vi "Position_TOTAL_R25test1111.vi"(5 "Distance Between \nCameras  (*unit)":sgl=2.3) -> (12 "dX, dY\nLeft Cam":cluster{"X":sgl[], "Y":sgl[]}={"X"=[-1.0065897, 0.099401906, 1.1628555, 2.2500029, 0.0], "Y"=[10.716516, 10.801518, 10.883252, 10.9668045, 0.0]}, 13 "Position Valid":bool=TRUE, 14 "Left Camera Real Coordinates":cluster{"X":sgl, "Y":sgl}={"X"=10.842023, "Y"=1.3735824}, 16 "dX, dY\nRight Cam":cluster{"X":sgl[], "Y":sgl[]}={"X"=[-2.8840373, -1.7780458, -0.7145921, 0.3725553, -1.8774476], "Y"=[9.387911, 9.472914, 9.554648, 9.638201, -1.3286046]}, 18 "Robot Coordinates":cluster{"X":sgl, "Y":sgl}={"X"=10.17772, "Y"=2.3123062}, 19 "Orietnation\n(current)":sgl=-30.94054 format="%#_13g")   [LabVIEW 2015]
uses:
  <vilib>/Analysis/coordinate.llb/2D Cartesian Coordinate Rotation (Array).vi
  <vilib>/myRIO/Common/Instrument Driver Framework/myRIO v1.0/DIO/vis/myRIO v1.0 Close DIO.vi
  <vilib>/myRIO/Common/Instrument Driver Framework/myRIO v1.0/DIO/vis/myRIO v1.0 Unreserve DIO.vi
  <vilib>/myRIO/Common/Instrument Driver Framework/myRIO v1.0/DIO/vis/myRIO v1.0 Build MUX Configuration DIO.vi
  <vilib>/myRIO/Common/Instrument Driver Framework/myRIO v1.0/Resource Manager/vis/myRIO v1.0 Unreserve Channel List.vi
  <vilib>/myRIO/Common/Instrument Driver Framework/myRIO v1.0/Resource Manager/vis/myRIO v1.0 Create Configuration List.vi
  <vilib>/myRIO/Common/Instrument Driver Framework/myRIO v1.0/Resource Manager/vis/myRIO v1.0 Unreserve Channel.vi
  <vilib>/myRIO/Common/Instrument Driver Framework/myRIO v1.0/Resource Manager/vis/myRIO v1.0 Build Mutex Name.vi
  <vilib>/Instr/_visa.llb/VISA Configure Serial Port (Instr).vi
  <vilib>/myRIO/Common/Instrument Driver Framework/myRIO v1.0/DIO/vis/myRIO v1.0 Shutdown DIO.vi
  <vilib>/Utility/error.llb/Error Cluster From Error Code.vi
  <vilib>/myRIO/Common/Instrument Driver Framework/myRIO v1.0/Resource Manager/vis/myRIO v1.0 Configure IO.vi
  <vilib>/myRIO/Common/Instrument Driver Framework/Utilities/vis/Configuration Manager.vi
  <vilib>/myRIO/Common/Instrument Driver Framework/Utilities/vis/IO Manager.vi
  <vilib>/myRIO/Common/Instrument Driver Framework/myRIO v1.0/myRIO v1.0 Close.vi
  <vilib>/Analysis/NI_AALPro.lvlib
  <vilib>/myRIO/Instrument Drivers/Onboard IO/DIO/DIO.lvlib
panel:
  in  "Boolean":bool
  in  "Skip Startup - LEFT":bool[](array[boolean])=[FALSE, TRUE, FALSE, FALSE, TRUE, FALSE, FALSE, TRUE]
  in  "Startup GP per Case - LEFT 2":u16[](array[numeric])=[920, 0, 260, 700, 0, 200, 650, 0, 358]
  in  "Start up Template State\n- LEFT":i32=1
  out "Current Template - Right":T1(ring)
  out "Current Template - Left":T1(ring)
  in  "Tab Control 2":T2(tab)
  out "Beacon Coordinates - Right Image":T3={"Beacon Position - X px"=[88.975365, 121.85722, 157.60713, 192.74931, 229.82234], "Beacon Position - Y px"=[106.21975, 102.49595, 103.61968, 103.22959, 103.920715]}
  out "Beacon Coordinates - Left Image":T3={"Beacon Position - X px"=[96.57839, 127.0317, 159.93825, 190.94315, 221.86247], "Beacon Position - Y px"=[111.67795, 107.306076, 106.92789, 105.73433, 104.09002]}
  in  "Image Width (px)":sgl=320.0
  in  "Image Height (px)":sgl=240.0
  in  "Cam AOV Horizontal (deg)":sgl=58.0
  in  "Cam AOV Vertical (deg)":sgl=45.0
  out "Angle to Pixel Ratios":T4={"Angle to Pixel\nRatio - Horizontal"=0.18125, "Angle to Pixel\nRatio - Vertical"=0.1875} {"Angle to Pixel\nRatio - Vertical" format="%#_13g"; "Angle to Pixel\nRatio - Horizontal" format="%#_13g"}
  in  "Num of Beacons (Total)":i8=5
  out "Left Data\nInput Flag\n- Internal":bool
  out "Right Data\nInput Flag\n- Internal":bool
  out "This Servo \nAngle - Left":sgl=52.96875
  in  "Valid Angles - L":bool[](array[boolean])=[TRUE, TRUE, TRUE, TRUE, TRUE]
  in  "Valid Angles -R":bool[](array[boolean])=[TRUE, TRUE, TRUE, TRUE, TRUE]
  in  "Beacon Angles - L":sgl[](array[numeric])=[64.19745, 58.642975, 52.682835, 47.05908, 41.446476]
  in  "Beacon Angles -R":sgl[](array[numeric])=[71.43643, 65.46979, 58.9926, 52.62266, 45.904842]
  out "This Servo \nAngle - Right":sgl=58.76953
  in  "Position Calc\nReady":bool=TRUE
  out "Array":sgl[](array[numeric])=[9.555056, 8.575206, 8.036942, 7.810829, 6.6351933]
  out "Array 2":sgl[](array[numeric])=[5.5039287, 6.210328, 7.1312, 8.266513, 8.73579]
  out "Array 3":sgl[](array[numeric])=[3.2039287, 3.9103284, 4.8311996, 5.9665127, 6.4357905]
  in  "stop":bool
  in  "Startup GP per Case - RIGHT":u16[](array[numeric])
  in  "Startup GP per Case - LEFT":u16[](array[numeric])
  in  "Servo Algorithm\nCycle Time(ms)":i32=25
  in  "Move Servo\nThreshold (deg)":sgl=2.0 format="%#_13g"
  in  "SERVO ENABLE":bool=TRUE
  in  "Max Write\nTx Attempts":u8=3
  in  "Max Read\nTx Attempts":u8=3
  in  "close comms":bool
  in  "Servo Comm\nLoop Time (ms)":i32=20
  out "dT - Comm Loop":u32=21
  in  "Left Servo\nID":string="\u0000"
  in  "Servo Comm\nWait Time - (ms)":i32
  in  "Right Servo\nID":string="\u0001"
  in  "Search Step Size\n(deg)":sgl=15.0 format="%#_13g"
  out "Last Orientation":sgl=-35.285717
  out "Last Position":cluster{"X":sgl, "Y":sgl}={"X"=10.147585, "Y"=2.64441}
  in  "Compliance Slope":u8=128
  in  "Search Step Size":u16=50
  in  "Mounting Offset - Left":sgl=-45.0
  in  "Minimum Delta \nServo Threshold":i16=3
  in  "Maximum Move \nServo Threshold":i16=300
  in  "Wait Tick Threshold":i32=10
  in  "Min Num Frames\nper Search":i32=5
  in  "Middle Beacon\nCoordinates":cluster{"X":sgl, "Y":sgl}={"X"=0.0, "Y"=2.5}
  in  "Max Recovery\nSearch Attempts":u16=3
  in  "Max Recovery Count\n(Recovery Search)":u16=20
  in  "Mounting Offset - Right":sgl=45.0
  in  "Tracking Timeout\nThreshold":i32=10
  in  "Timeout to \nEnable Reactive Predict":u16=5
  out "Beacon Scales - Right":sgl[](array[numeric])=[50.81787, 54.150085, 54.01553, 51.723366, 54.605507]
  out "Beacon Scales - Left":sgl[](array[numeric])=[46.59789, 48.180458, 47.842606, 46.504417, 45.297752]
  in  "Recovery Parallel\nSearch Offset":u16=50
  in  "Max # Pan Moves":u16=20
  in  "Current Angle\n - Right (internal)":sgl=58.76953
  in  "Current Angle\n - Left (internal)":sgl=52.96875
  in  "Servo Goal Position\n - Left":u16=360
  in  "Servo Goal Position\n - Right":u16=667
  out "Move Servo - R":bool
  out "Move Servo - L":bool
  out "Current L (10bit)":u16=232
  out "Servo Moving - L":bool
  out "Servo Moving - R":bool
  out "Current R (10bit)":u16=559
  out "deltaMoveServo\n- L":i16
  out "Move Respond - L":bool
  out "Move Respond - R":bool
  out "deltaMoveServo\n- R":i16
  out "Current Main State - Left":T5(ring)=enum."Tracking"
  in  "Initial Main State - Left":T5(ring)
  in  "Image Lock - Left":bool=TRUE
  in  "Track Angle Valid - Left":bool=TRUE
  out "New Data  Flag\nLeft Servo":bool
  in  "Tracking Angle - Left":sgl=52.933372
  in  "Search Direction - in - L":bool
  out "Frames Processed\nCount - in -L":i32
  out "Recovery Mode Count - in Left":u16
  in  "Image Lock - Right":bool
  out "Recovery Search\nmove Count - in - L":u16
  out "Recovery Search\nAttempt Count - in - L":u16
  out "Current Move Delta - L":u16
  out "Next Main State - Left":T5(ring)=enum."Tracking"
  in  "Recovery Search\nDirection - L":bool=TRUE
  out "Last Track Angle - L":sgl=52.96875
  in  "Initial Main State- Right":T5(ring)
  out "Current Main State - Right":T5(ring)=enum."Tracking"
  in  "Track Angle Valid  - Right":bool
  out "New Data  Flag\nRight Servo":bool
  in  "Tracking Angle - Right":sgl=58.953144
  out "Recovery Search\nAttempt Count - Right":u16
  out "Recovery Search\nmove Count - Right":u16
  out "Frames Processed\nCount - in Right":i32
  out "Recovery Mode Count in Right":i32
  in  "Recovery Search\nDirection - R":bool
  out "Next Main State - Right":T5(ring)=enum."Tracking"
  in  "Search Direction - in - Right":bool=TRUE
  out "Tracking Timeout\nCount - L":i32
  out "Tracking Timeout\nCount - R":i32
  out "Current Tracking State - Left":enum16{"Track", "Reactive Predict", ""}(ring)
  in  "Initial Tracking State - Left":enum16{"Track", "Reactive Predict", ""}(ring)
  out "Next Tracking State - Left":enum16{"Track", "Reactive Predict", ""}(ring)
  in  "Initial Tracking State - Right":enum16{"Track", "Reactive Predict", ""}(ring)
  out "Current Tracking State - Right 2":enum16{"Track", "Reactive Predict", ""}(ring)
  out "Next Tracking State - Right":enum16{"Track", "Reactive Predict", ""}(ring)
  in  "Initial Recovery State - L":enum16{"Generic Sweep", "Recovery Search"}(ring)=enum."Recovery Search"
  in  "Initial Recovery State  - Right":enum16{"Generic Sweep", "Recovery Search"}(ring)=enum."Recovery Search"
  out "Current Recovery State - Right":enum16{"Generic Sweep", "Recovery Search"}(ring)=enum."Recovery Search"
  out "Next Recovery State - Right":enum16{"Generic Sweep", "Recovery Search"}(ring)=enum."Recovery Search"
  out "Next Recovery State - Left":enum16{"Generic Sweep", "Recovery Search"}(ring)=enum."Recovery Search"
  out "Current Recovery State -L":enum16{"Generic Sweep", "Recovery Search"}(ring)=enum."Recovery Search"
  out "Current Move Delta - R":u16
  in  "Mining Alignment\nEnabled":bool
  in  "Real Beacon\n - Coordinates":cluster{"X":dbl[], "Y":dbl[]}={"X"=[0.0, 0.0, 0.0, 0.0, 0.0, 0.0], "Y"=[0.5, 1.5, 2.5, 3.5, 4.5, 0.0]}
  out "LOCAL\nBeacon Coordinates\nRelative to Robot":cluster{"dX_beacon":sgl[], "dY_beacon":sgl[]}={"dX_beacon"=[5.5039287, 6.210328, 7.1312, 8.266513, 8.73579], "dY_beacon"=[9.555056, 8.575206, 8.036942, 7.810829, 6.6351933]}
  out "Local Coordinates - Calculated":cluster{sgl[], sgl[]}(graph)={[5.5039287, 6.210328, 7.1312, 8.266513, 8.73579], [9.555056, 8.575206, 8.036942, 7.810829, 6.6351933]}
  out "Distance to LBF":sgl[](array[numeric])=[0.024284193, 0.015691843, 0.008273765, 0.028971607, 0.03291407]
  out "Right Camera Real Coordinate":cluster{"X":sgl, "Y":sgl}={"X"=9.513418, "Y"=3.25103}
  out "Post Filtering\n- Valid Beacons":bool[](array[boolean])=[TRUE, TRUE, TRUE, TRUE, FALSE]
  in  "Distance\nBetween Beacons":sgl=1.0 format="%#_13g"
  in  "Distance\nBetween Beacons \n- Tolerance":sgl=0.5 format="%#_13g"
  in  "Distance Threshold\nRef Triangles (*unit)":sgl=30.0
  out "All Object Coordinates \n- Local":cluster{"X":sgl[], "Y":sgl[]}={"X"=[2.3, 5.368779, 6.320682, 7.235974, 8.171657, 0.0], "Y"=[0.0, 9.329155, 8.759661, 8.21207, 7.6522775, 0.0]}
  out "Local Coordinates - Normalized":cluster{sgl[], dbl[]}(graph)={[2.3, 5.368779, 6.320682, 7.235974, 8.171657, 0.0], [0.0, 9.329154968261719, 8.759660720825195, 8.21207046508789, 7.65227746963501, 0.0]}
  out "All Object Coordinates \n- Local - Rotated":cluster{"X":sgl[], "Y":sgl[]}={"X"=[1.8774476, -1.0065897, 0.099401906, 1.1628555, 2.2500029, 0.0], "Y"=[1.3286046, 10.716516, 10.801518, 10.883252, 10.9668045, 0.0]}
  out "Local Coordinates - Rotated":cluster{dbl[], dbl[]}(graph)={[1.8774476489648846, -1.0065896210507148, 0.09940190570174412, 1.1628555490135675, 2.250002943734801, 0.0], [1.3286045709883498, 10.716515276262749, 10.801518262128845, 10.883252530212562, 10.966804865321656, 0.0]}
  out "Right_Flag 2":bool
  out "Beacons Found\n- Right (Bool Array)":bool[](array[boolean])=[TRUE, TRUE, TRUE, TRUE, TRUE]
  out "RIGHT Beacon Position - Y px (IN)":sgl[](array[numeric])=[106.21975, 102.49595, 103.61968, 103.22959, 103.920715]
  out "RIGHT Beacon Coord - X px (IN)":sgl[](array[numeric])=[88.975365, 121.85722, 157.60713, 192.74931, 229.82234]
  out "Left_Flag 2":bool
  out "Beacons Found\n- Left (Bool Array) 2":bool[](array[boolean])=[TRUE, TRUE, TRUE, TRUE, TRUE]
  out "LEFT Beacon Coord - X px (IN) 2":sgl[](array[numeric])=[96.57839, 127.0317, 159.93825, 190.94315, 221.86247]
  out "LEFT Beacon Position - Y px (IN) 2":sgl[](array[numeric])=[111.67795, 107.306076, 106.92789, 105.73433, 104.09002]
  in  "Fetch Input\n(mSec)":u32=20 caption="Update Camera Input\n(mSec)"
  in  "Max Std Dev (5)":sgl=0.1 format="%#_13g"
  out "Position \nLock Status":bool=TRUE
  out "Real Position in Course 2":cluster{"X":dbl[], "Y":dbl[]}(graph)={"X"=[10.147584990557128], "Y"=[2.644409845240164]}
  out "Robot Coordinates - Avgd":cluster{"X":sgl, "Y":sgl}={"X"=10.147585, "Y"=2.64441}
  in  "Max Std Dev (4)":sgl=0.1 format="%#_13g"
  in  "Max Std Dev (3)":sgl=0.2 format="%#_13g"
  in  "New Position\nWeight (X coord)":sgl=0.8 format="%#_13g"
  in  "Max X (arena)":sgl=35.0
  in  "Max Y (arena)":sgl=15.0
  in  "History Size":u8=15
  out "Orientation Avgd":sgl=-35.285717
  in  "New Position \nThreshold":sgl=2.0
  out "Robot Coordinates\nHistory":cluster{sgl, sgl}[](array[cluster])=[{10.147585, 2.64441}, {10.056327, 2.8351064}, {10.020484, 2.7815769}, {10.034186, 2.7172103}, {0.0, 0.0}, {10.036168, 2.7859242}, {9.938812, 2.8961887}, {10.1160965, 2.6632404}, {10.016709, 2.7454932}, {10.037537, 2.8544023}, {10.017025, 2.7817721}, {9.997087, 2.8064857}, {10.065648, 2.6537364}, {10.084976, 2.6750228}, {10.082739, 2.688601}]
  out "Orientation\nHistory":sgl[](array[numeric])=[-35.285717, -36.86449, -36.153664, -35.44657, 0.0, -37.6105, -36.02637, -35.82032, -36.08894, -37.01076, -36.293255, -36.40525, -35.738438, -35.683483, -35.770218]
  out "Position Valid\nHistory":bool[](array[boolean])=[TRUE, TRUE, TRUE, TRUE, FALSE, TRUE, TRUE, TRUE, TRUE, TRUE, TRUE, TRUE, TRUE, TRUE, TRUE]
  in  "Moving Average\nWindow Length":u8=10
  in  "New Orientation \nThreshold":sgl=10.0
  in  "Triangle Based\nWeight":sgl format="%#_13g"
  out "Scale Based\nWeight":sgl=1.0 format="%#_13g"
  out "New Position\nWeight (Y coord)":sgl=0.3 format="%#_13g"
  out "New Orientation\nWeight":sgl=0.2
  out "dT":dbl=144.111
  in  "Position Calc\nTimer":u32=100 caption="Position Calc Timer"
  out "inches":dbl
  out "dA2 3":sgl=44.126 format="%#_13g"
  out "Valid Beacon Sets_":bool[](array[boolean])=[TRUE, TRUE, TRUE, TRUE, TRUE]
  in  "Check Shared Var Timer":u32=50 caption="Main Loop\n Timer (ms)"
  out "dA2 2":sgl=48.543114 format="%#_13g"
  out "dA2 4":sgl=48.543114 format="%#_13g"
  out "Last Track Angle - R":sgl=59.941406
  in  "Recovery Search\nDirection - L 2":bool
  in  "Max Recovery Count\n(Recovery Search) 2":u16
  in  "Max Recovery\nSearch Attempts 2":u16
  in  "Image Lock - Right 2":bool
  # "SETTINGS"
  # "IMAGE TO ANGLE VARIABLES"
  # "INPUTS"
  # "OUTPUT VALUES"
  # "CONFIG"
  # "SERVO CONTROL VARIABLES"
  # "SERVO CONTROL VARIABLES"
  # "CONFIG"
  # "SHARED VARIABLE INPUTS"
  # "LOCAL VARIABLE INPUTS"
  # "INTERNRAL VARIABLES"
  # "MISC"
  # "SERVO IDs"
  # "CONTROL DELAYS"
  # "COMM LOOP DELAY"
  # "COMM PROTOCOL"
  # "INDEX Correspondance: \n\n0 - 3  --> Side 1 / N, S, E, W\n4 - 7 -->  Side 2 / N, S, E, W\n9 --> Straight ahead (90deg)"
  # "Make function of distance^^"
  # "LEFT SERVO"
  # "RIGHT SERVO"
  # "Main State Machine"
  # "Recovery State Machine"
  # "Current Track Angle Inputs"
  # "Servo Status Inputs"
  # "Main State Machine Inputs"
  # "Recovery State Machine Inputs"
  # "Current Track Angle Inputs"
  # "Servo Status Inputs"
  # "Tracking State Machine Inputs"
  # "Tracking State Machine Inputs"
  # "POSITION CALCULATION VARIABLES"
  # "OUTPUT VALUES"
  # "CONFIG VALUES"
  # "FILTER CONFIG VALUES"
  # "FEEDBACK INPUT VALUES"
  # "INPUT VALUES"
  # "INTERMEDIATE VALUES"
  # "Use moving average for previous orientation thresholds"
  # "*********************"
  # "unfiltered"
  # "Inter Beacon Distance Filtering"
  # "NOTE: Must be 1 bigger than amount of beacons"
  # "NOTE: Must be 1 bigger than amount of beacons"
  # "VISION PROCESSEING INPUTS"
  # "update to coordinate outlier filtering R2"
  # "NEW FILTER VALS"
  # "MOVING AVERAGE\nVARIABLES"
  # "DISTANCE SOURCE WEIGHT"
  # "*****  I made this 0\n         bc it seems to be \n        more stable"
  # "Recovery State Machine Feedback"
  # "SEARCH ROUTINE VARIABLES"
types:
  T1 = enum16{"Range 1", "Range 2", "Range 3", "Range 0"}
  T2 = enum32{"image to angle ", "Empty", "servo control - Config", "left and right servo - Status", "Position Calc - Debug Data", "Position Calc - Debug Data 2", "Vision Processing INputs", "ROBOT POSITION", "Random"}
  T3 = cluster{"Beacon Position - X px":sgl[], "Beacon Position - Y px":sgl[]}
  T4 = cluster{"Angle to Pixel\nRatio - Horizontal":sgl, "Angle to Pixel\nRatio - Vertical":sgl}
  T5 = enum16{"Start Up Search", "Tracking", "Recovery Mode", ""}
  T6 = cluster{"Lock":bool, "Current Valid":bool, "Current Template":enum16{"Range 1", "Range 2", "Range 3", "Range 0"}, "Tracking Coordinates":cluster{"X":dbl, "Y":dbl}, "Setting Values":cluster{"Min Score":dbl, "Min Scale":dbl, "Max Scale":dbl, "Curve Parameters":cluster{"Min Length":i32, "Row Search Step":i32, "Col Search Step":i32}}}
  T7 = cluster{"Array of Double":dbl[], "Array of Double":dbl[]}
  T8 = enum16{"Sub - 2", "Sub - 3", "Sub - 4", "Normal - 5"}
  T9 = typedef "DIO.lvlib/DIO Reference.ctl" = cluster{"myRIO Reference":T10, "DIO Channels List":T14}
  T10 = typedef "myRIO Generic Hardware Reference.ctl" = cluster{"myRIO Model":T11, "myRIO Hardware Reference":T12}
  T11 = typedef "Hardware Version Enum.ctl" = enum16{"Unknown", "myRIO-1900", "myRIO-1950", "roboRIO"}
  T12 = typedef "myRIO v1.0 Reference.ctl" = cluster{"Generic FPGA Reference":T13, "Allow multiple opens":bool}
  T13 = typedef "Generic FPGA Reference.ctl" = refnum<k20>
  T14 = typedef "DIO Channels List.ctl" = T15[]
  T15 = typedef "DIO Channels Enum.ctl" = enum16{"Not Connected", "C/DIO0", "C/DIO1", "C/DIO2", "C/DIO3", "C/DIO4", "C/DIO5", "C/DIO6", "C/DIO7", "A/DIO0", "A/DIO1", "A/DIO2", "A/DIO3", "A/DIO4", "A/DIO5", "A/DIO6", "A/DIO7", "A/DIO8", "A/DIO9", "A/DIO10", "A/DIO11", "A/DIO12", "A/DIO13", "A/DIO14", "A/DIO15", "B/DIO0", "B/DIO1", "B/DIO2", "B/DIO3", "B/DIO4", "B/DIO5", "B/DIO6", "B/DIO7", "B/DIO8", "B/DIO9", "B/DIO10", "B/DIO11", "B/DIO12", "B/DIO13", "B/DIO14", "B/DIO15", "LED0", "LED1", "LED2", "LED3", "Button0", "DIO/DIO0", "DIO/DIO1", "DIO/DIO2", "DIO/DIO3", "DIO/DIO4", "DIO/DIO5", "DIO/DIO6", "DIO/DIO7", "DIO/DIO8", "DIO/DIO9", "SPI/CS0", "SPI/CS1", "SPI/CS2", "SPI/CS3", "LED RADIO (Green)", "LED RADIO (Red)", "LED COMM (Green)", "LED COMM (Red)", "LED MODE (Green)", "LED MODE (Red)"}
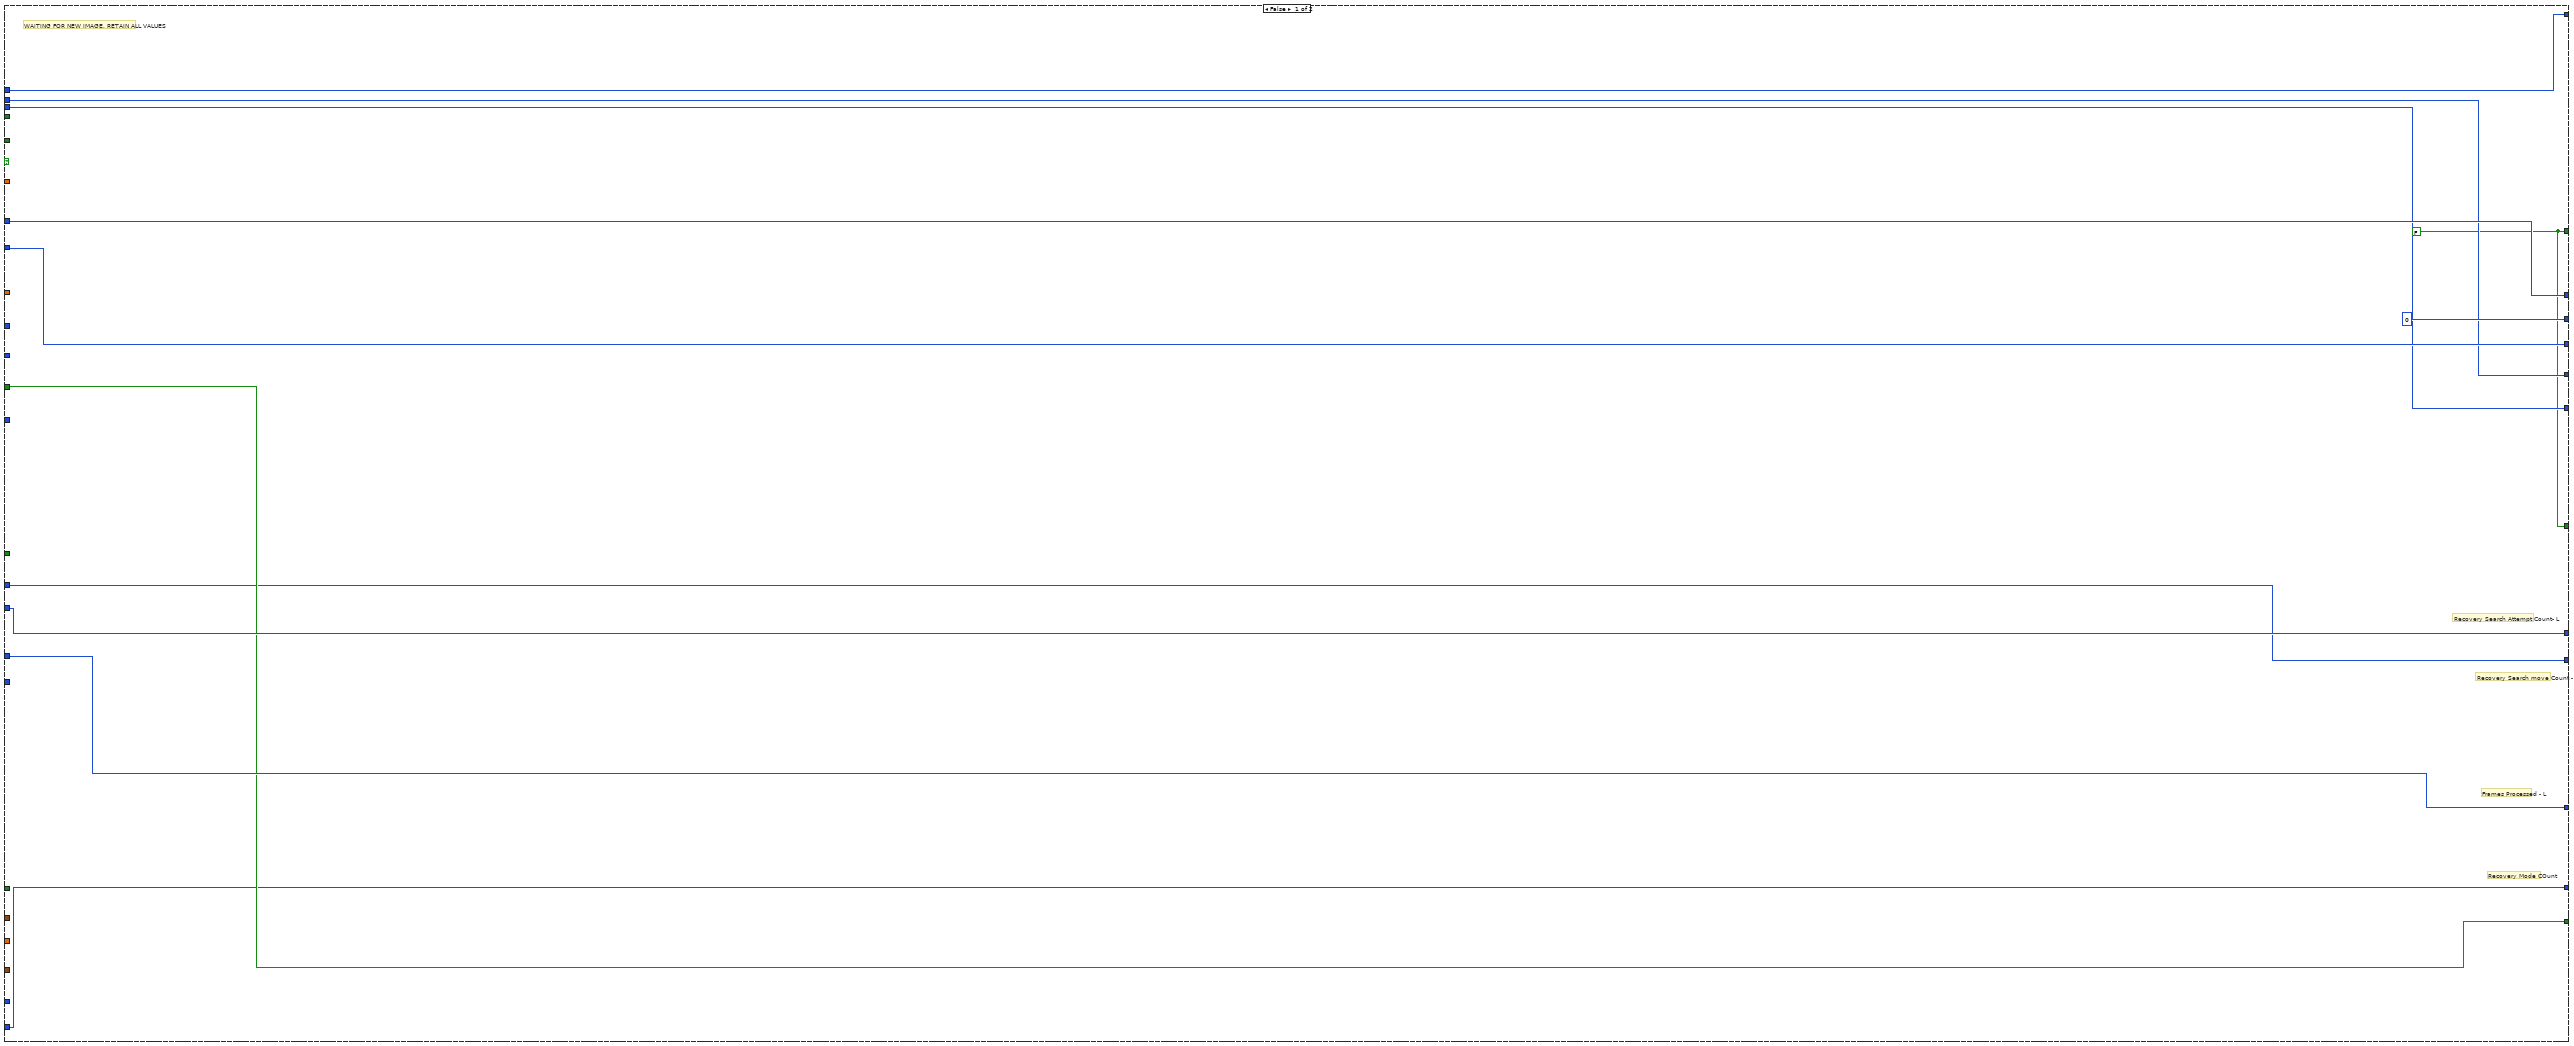
[diagram p2: hidden frame]
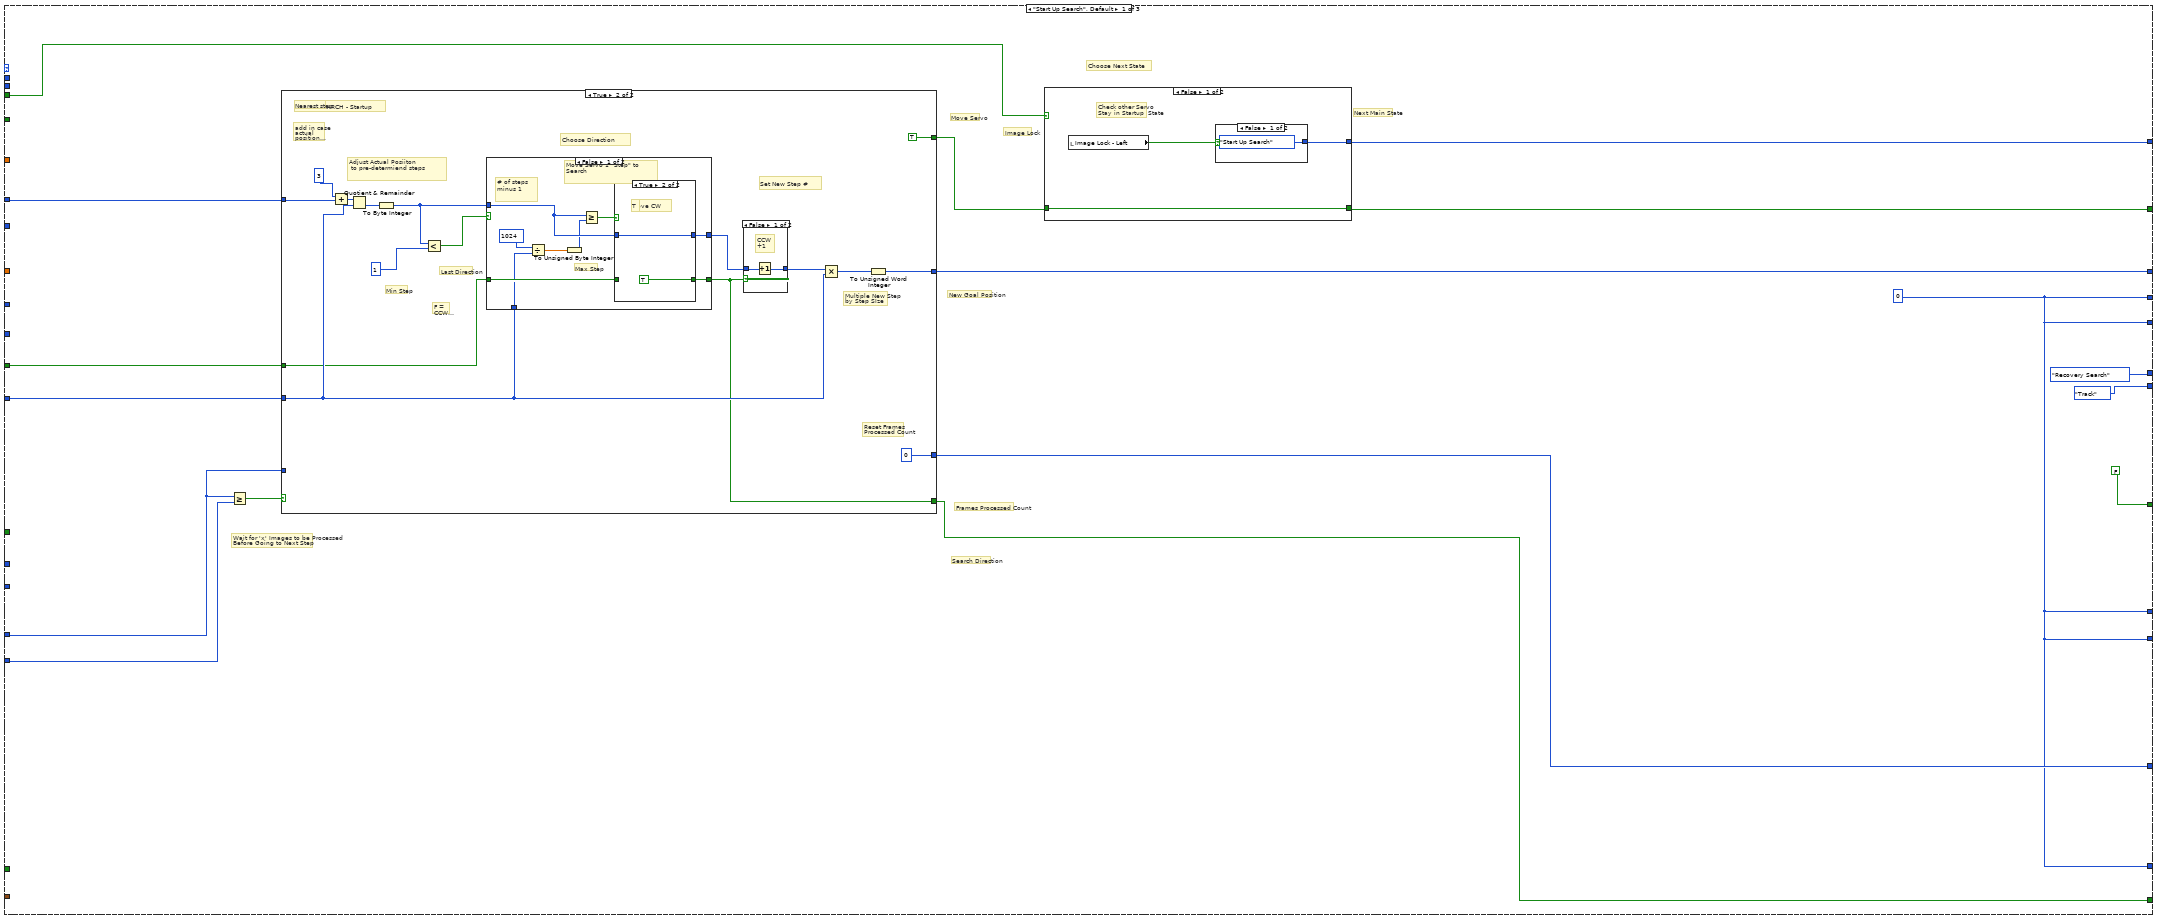
[diagram p3: hidden frame]
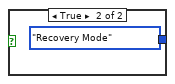
[diagram p4: hidden frame]
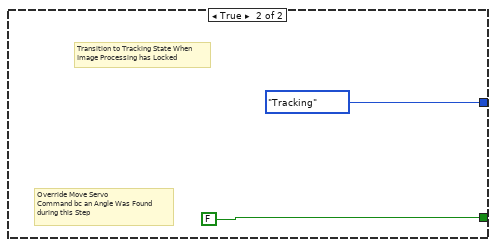
[diagram p5: hidden frame]
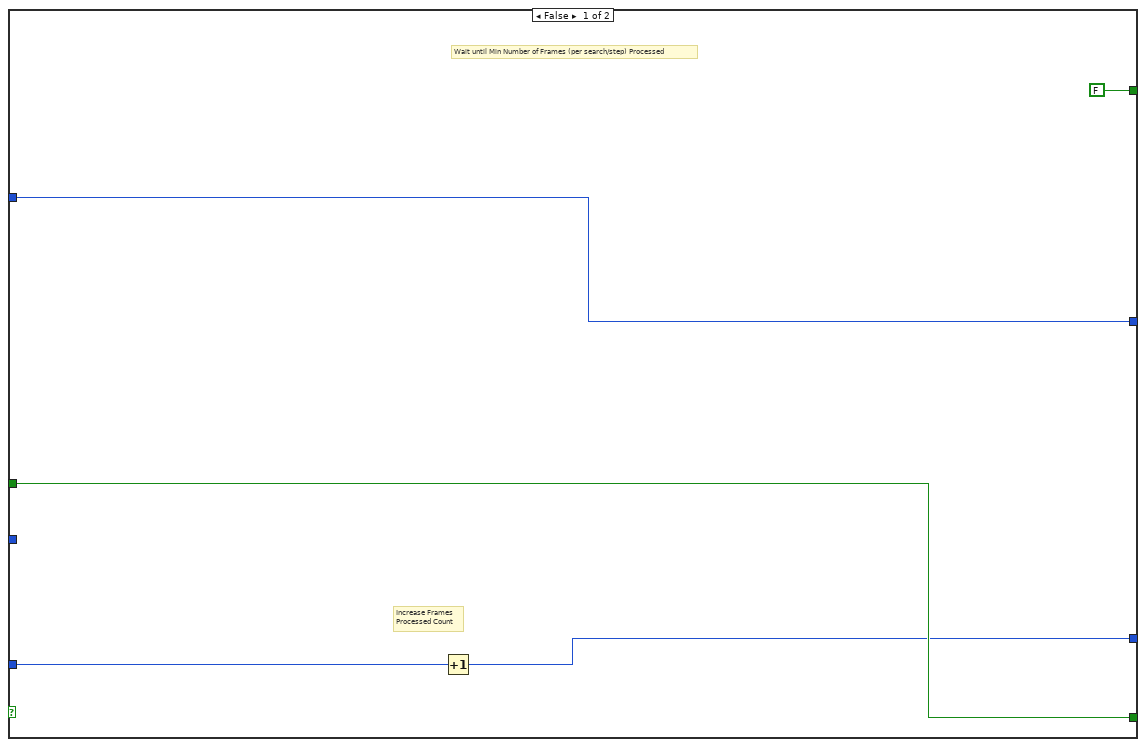
[diagram p6: hidden frame]
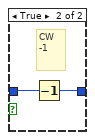
[diagram p7: hidden frame]
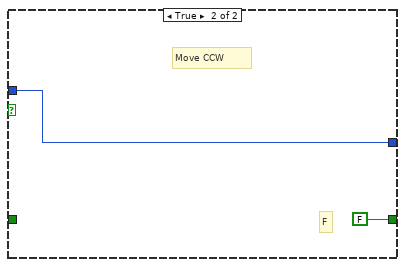
[diagram p9: hidden frame]
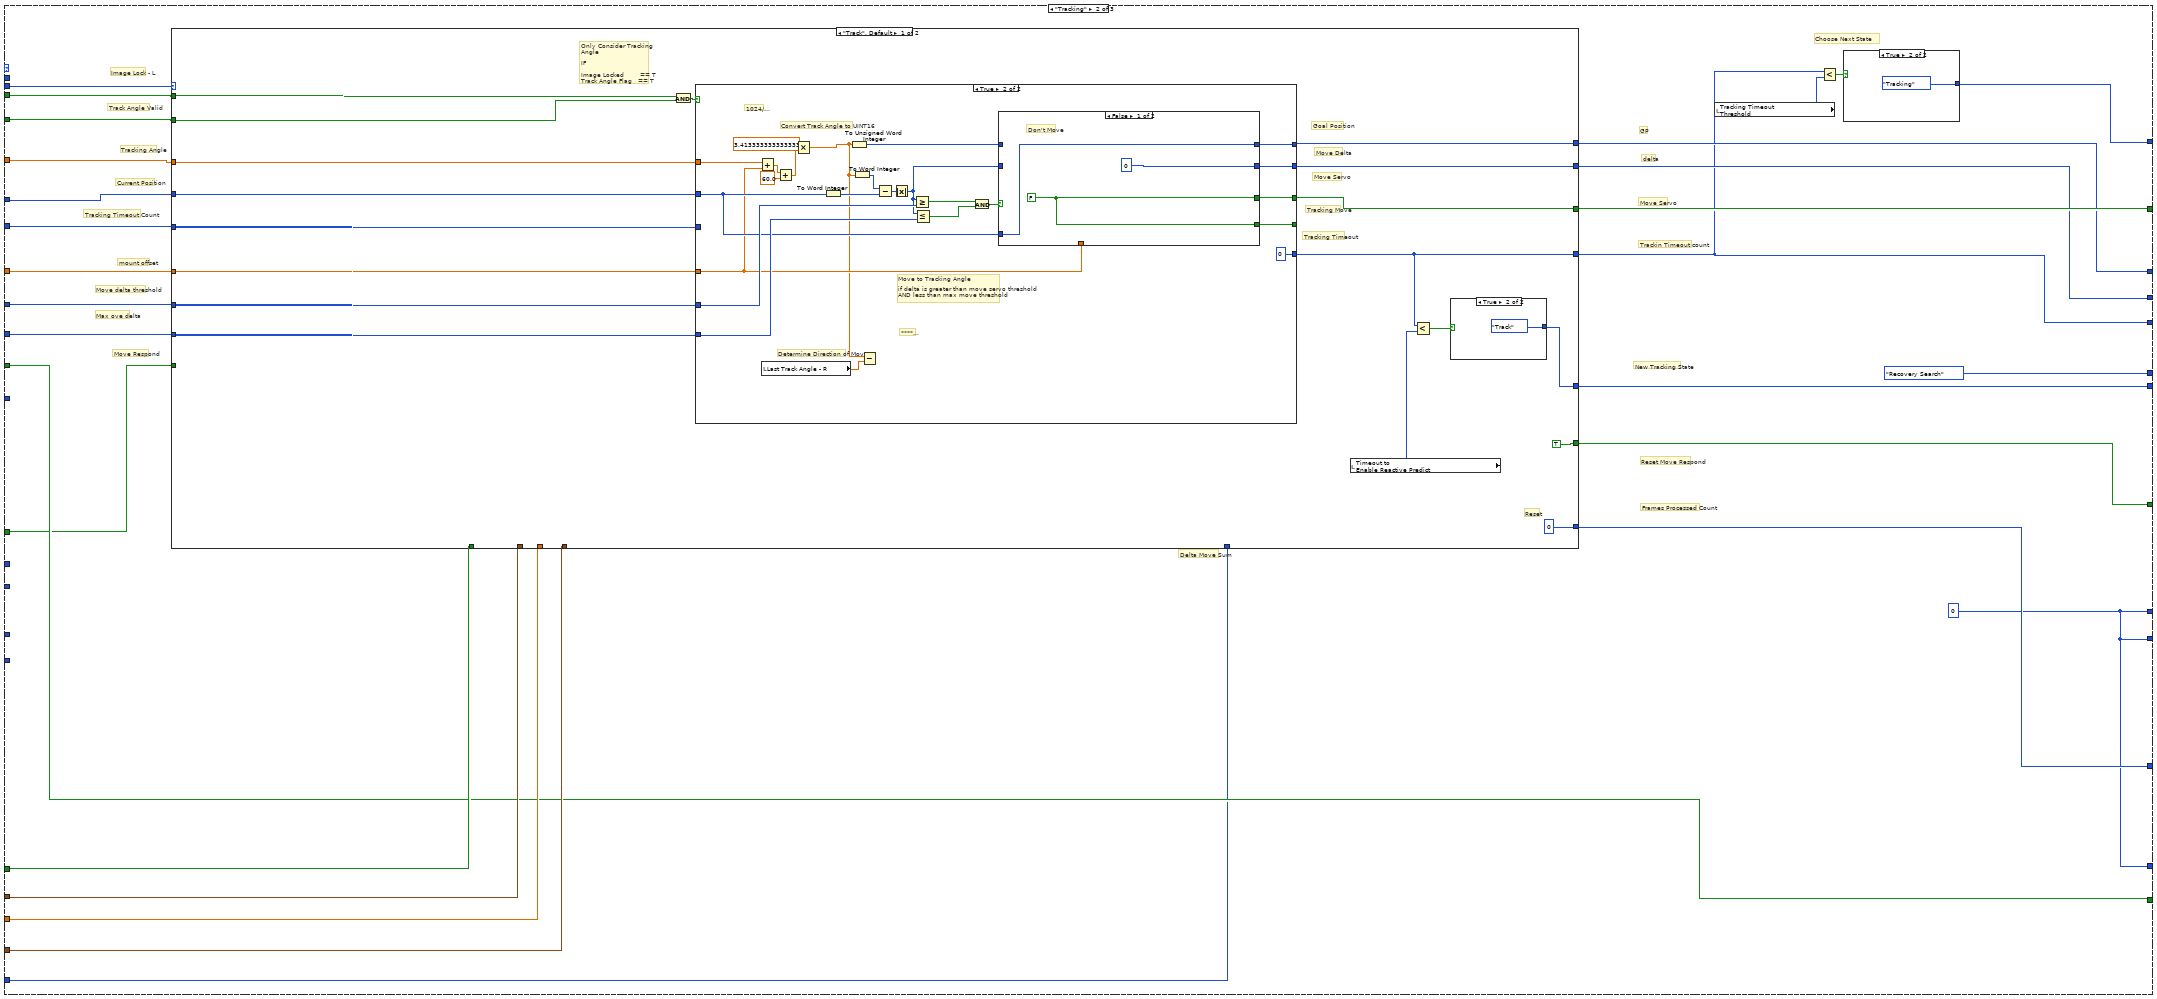
[diagram p10: hidden frame]
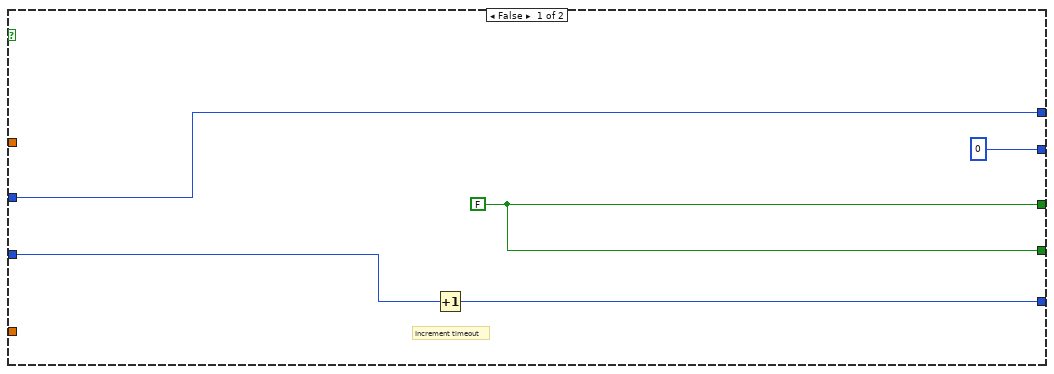
[diagram p11: hidden frame]
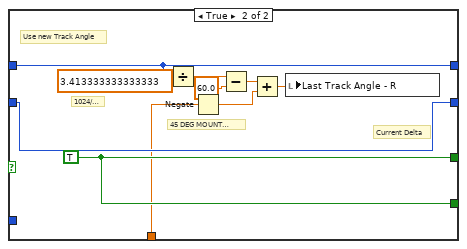
[diagram p12: hidden frame]
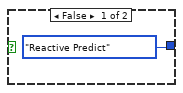
[diagram p13: hidden frame]
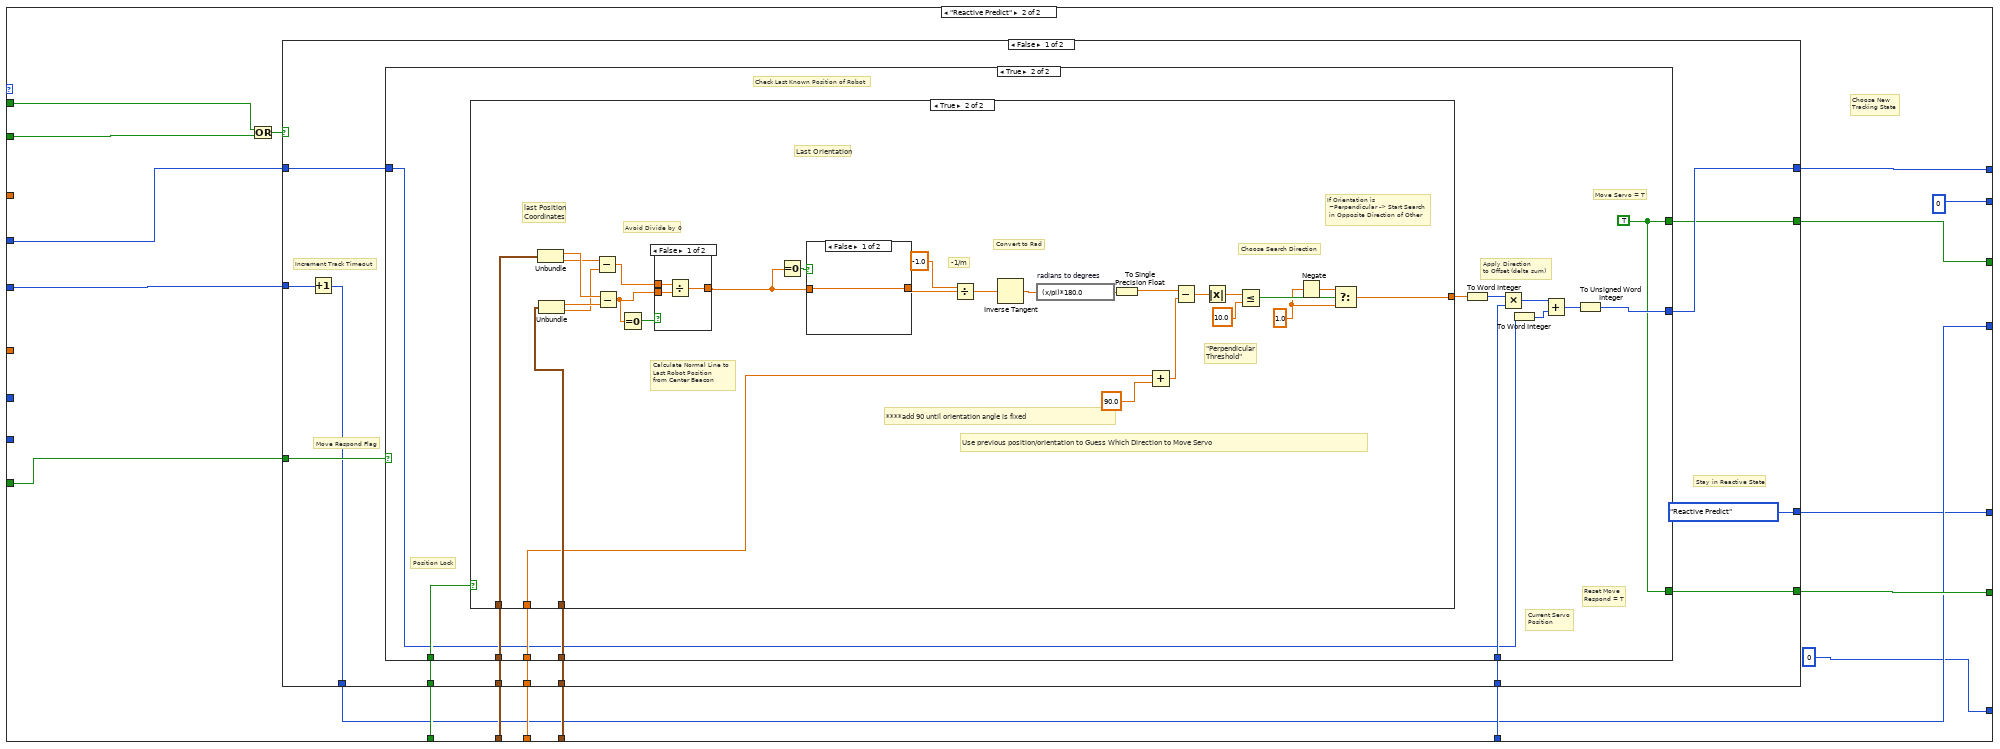
[diagram p14: hidden frame]
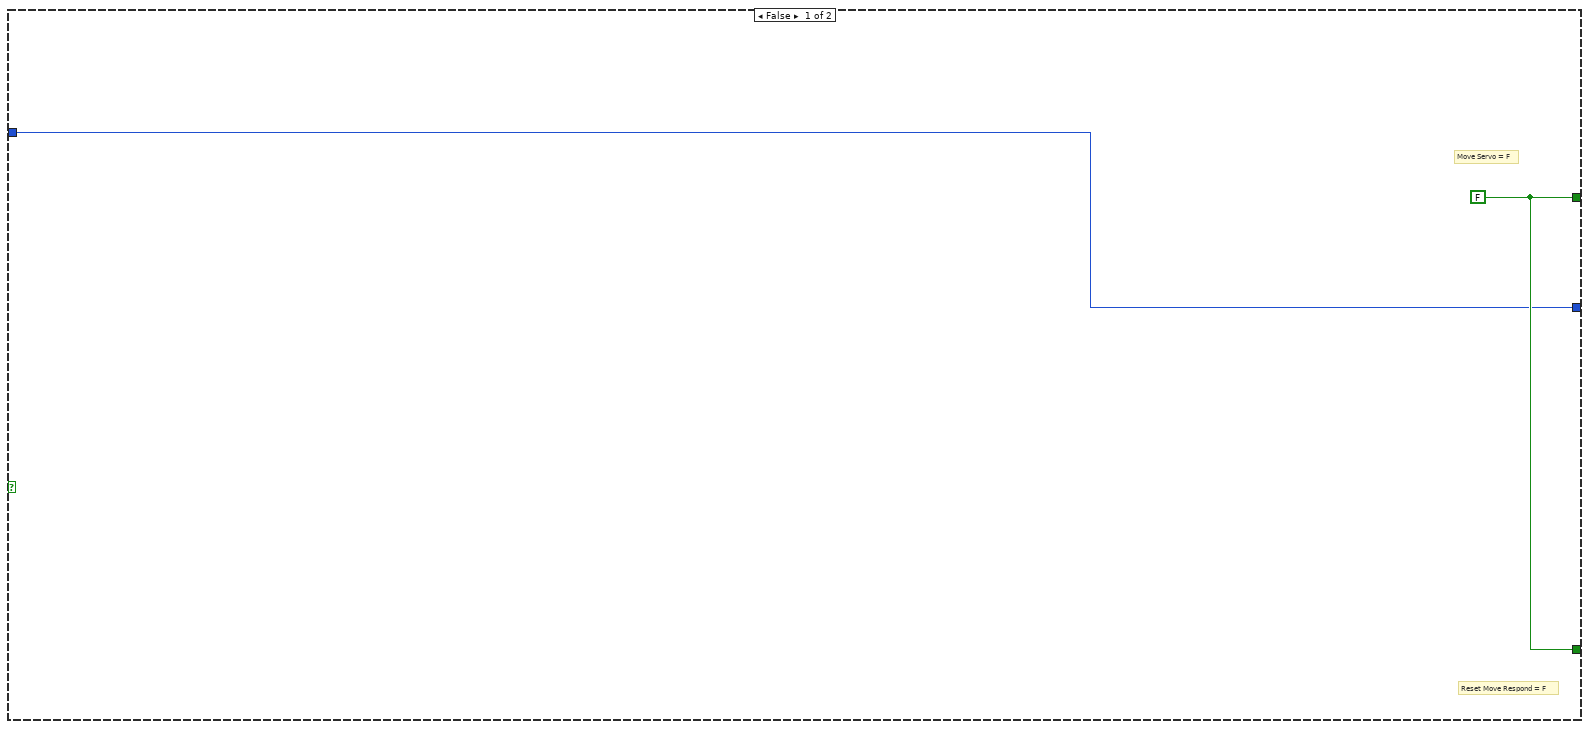
[diagram p15: hidden frame]
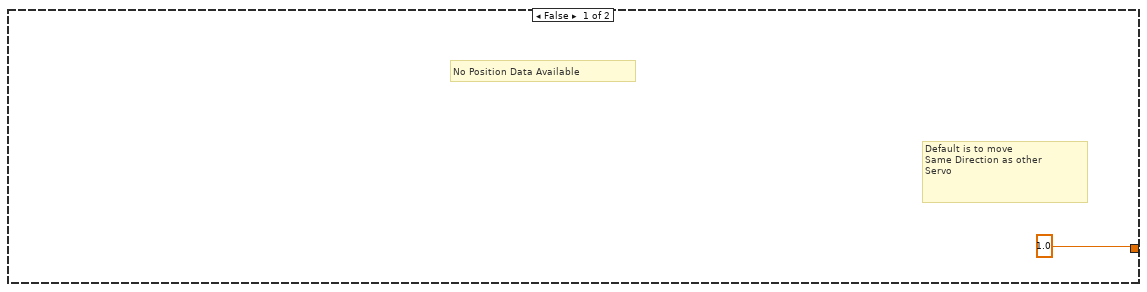
[diagram p16: hidden frame]
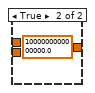
[diagram p17: hidden frame]
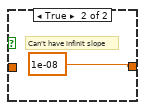
[diagram p18: hidden frame]
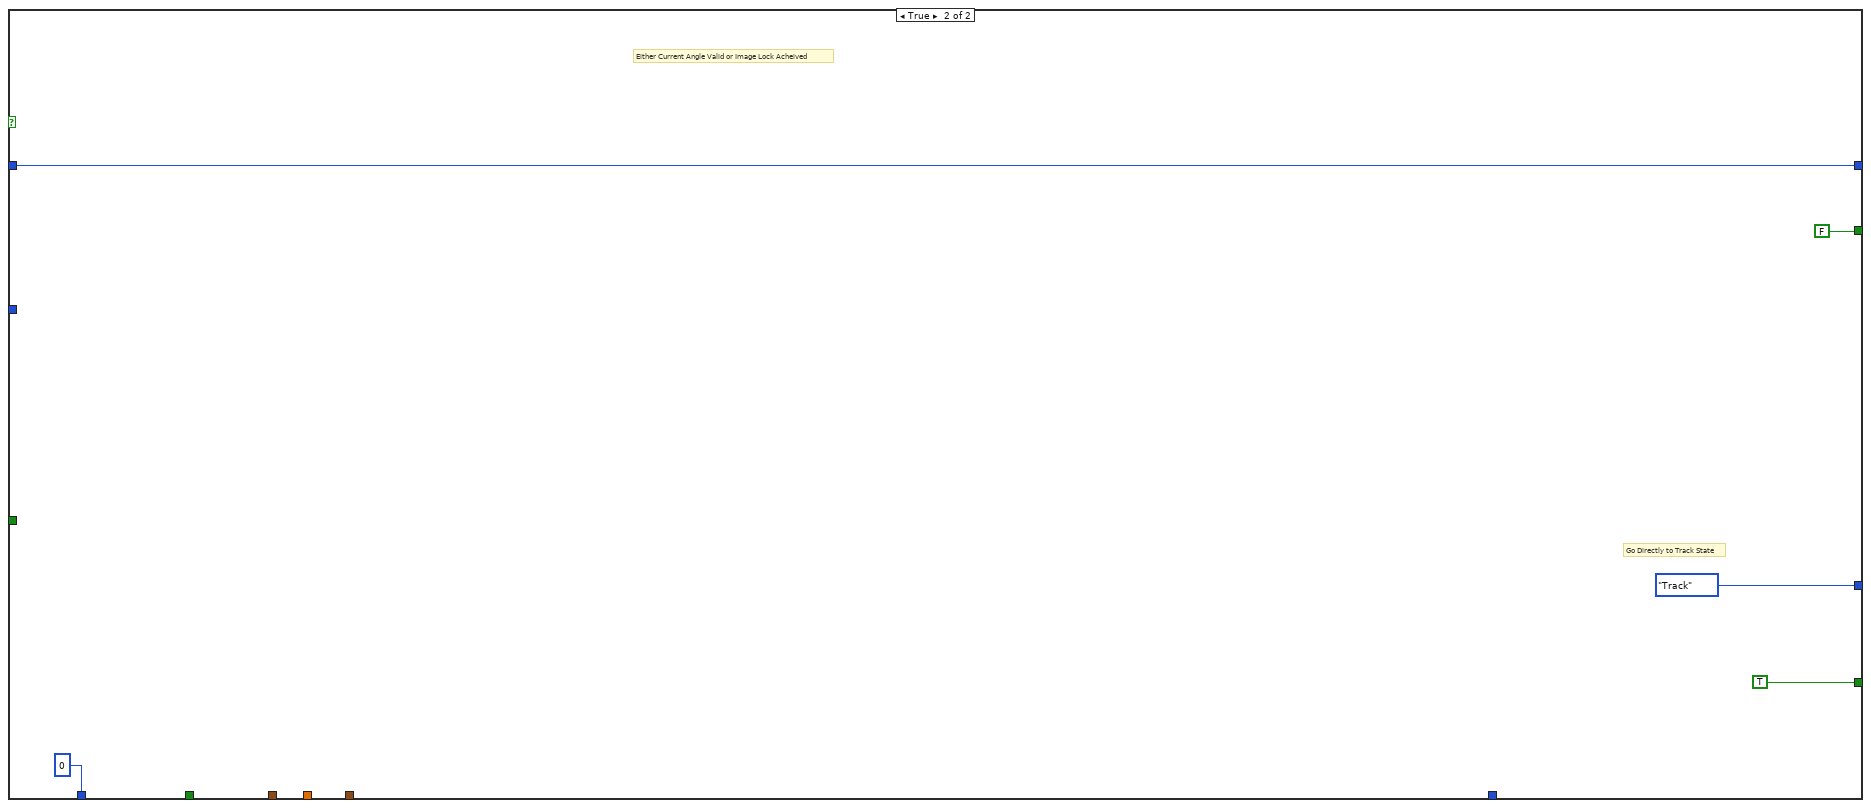
[diagram p19: hidden frame]
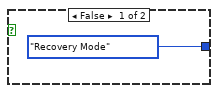
[diagram p20: hidden frame]
diagram:
  (unwired) enum16{"Generic Sweep", "Recovery Search"}."Recovery Search"
  w12 = 0 ("Frames Processed\nCount - in")
  w13 = 0 ("Frames Processed\nCount - in")
  w2 = FALSE
  w34 = sgl 0.0
  # "SERVO CONTROL FLAGS"
  # "***"
  # "Next Tracking State"
  # "Tracking Timeout Count"
  # "Search Direction - L"
  # "Next Recovery State"
  # "Move Respond"
  # "Recovery Mode Count - L"
  # "Delta Move Sum - L"
  # "Wait Tick Count - L"
  # "Frames Processed - L"
  # "Recovery Search move Count - L"
  # "Recovery Search Attempt Count- L"
  # "Next Main State"
  # "Search Direction - L"
  # "Next Recovery State"
  # "INPUTS - Local vars"
  # "Recovery Mode Count - L"
  # "Delta Move Sum - L"
  # "Frames Processed\nLeft"
  # "Move Respond - R"
  # "Initial Search Direction\n- Right"
  # "Move Respond"
  # "Recovery Mode Count - L"
  # "Delta Move Sum - L"
  # "Wait Tick Count - L"
  # "Frames Processed - L"
  # "Recovery Search move Count - L"
  # "Recovery Search Attempt Count- L"
  # "Next Main State"
  # "Settings -- Update in a slow loop"
  # "Recovery Mode Count - L"
  # "Delta Move Sum - L"
  # "Frames Processed\nLeft"
  # "Move Respond - L"
  # "Replace these with\nconstants"
  # "Initial Search Direction\n- Left"
  # "Read Inputs when Available"
  # "# of Physical Beacons"
  # "Right Data Internal Falg"
  # "Left Data Internal Falg"
  # "Initialize Shift Arrays"
  # "Robot Position (cluster)\nShift Array"
  # "Robot Position (cluster)\nShift Array"
  # "Position Valid Shift Array"
  # "Orientation Shift Array"
  # "Position Valid Shift Array"
  # "Orientation Shift Array"
  # "Servo Communication (to Servo- UART))"
  # "Internal Local Variables"
  # "Servo Control Logic"
  # "Local Variables"
  # "Images to Robot Position Calculation Process"
  # "SERVO MOTOR CONTROL"
  # "SERVO MOTOR CONTROL"
  n1 = Divide(x="Cam AOV Horizontal (deg)", y="Image Width (px)") -> (x/y=w25:sgl)
  n2 = Divide(x="Cam AOV Vertical (deg)", y="Image Height (px)") -> (x/y=w26:sgl)
  n3 = Bundle(w25, w26) -> (w20:cluster{sgl, sgl})  [unwired: 1 in]
  "Angle to Pixel Ratios" <- w20
  n4 = disable-structure shown="Disabled" {
    frame Disabled {
      # "Always Read Incoming Flags & Store"
      n5 = while {
        tunnel: "Check Shared Var Timer" -> [w46]
        stop <- FALSE stop-if-true
        n6 = shared-variable "myRIO-1900\\Lib1.lvlib\\RIGHT_FLAG"() -> (→"Right_Flag 2":bool)  [unwired: 1 in, 1 out]
        n7 = shared-variable "myRIO-1900\\Lib1.lvlib\\Left_Flag"() -> (→"Left_Flag 2":bool)  [unwired: 1 in, 1 out]
        n8 = call "Wait8"("Count(mSec)"=w46) -> ()  [unwired: 1 out]
      }
    }
    frame Enabled {
    }
  }
  n9 = while {
    shift-right: [w55] -> _
    shift-left: w2 -> [w60]
    shift-right: [w54] -> _
    shift-left: w2 -> [w58]
    tunnel: w20 -> [w56]
    tunnel: "Num of Beacons (Total)" -> [w57]
    stop <- FALSE stop-if-true
    # "Wait for Both Internal Flags"
    n10 = call "Wait6"("Count(mSec)"="Fetch Input\n(mSec)") -> ()  [unwired: 1 out]
    n11 = shared-variable "RT myRIO Target - Overlord\\Localization_Variables_r0.lvlib\\RIGHT_FLAG"() -> (w51:bool)  [unwired: 1 in, 1 out]
    n12 = shared-variable "RT myRIO Target - Overlord\\Localization_Variables_r0.lvlib\\Left_Flag"() -> (w52:bool)  [unwired: 1 in, 1 out]
    n13 = case shown="True" w51 {
      tunnel: w57 -> [_ w79]
      tunnel: w56 -> [_ w77]
      tunnel: [w61 w67] -> w49
      tunnel: w58 -> [w61 _]
      frame False {
        # "Don't Update Servo Position\nbc we're waiting on new Data to\ncome in and the servo position\nwas set at the previous set of data"
      }
      frame True {
        w67 = TRUE
        # "Store Values"
        # "Raise Internal Flag"
        # "If New Data Available"
        # "From Shift Reg"
        # "Perforrm Indivudual Angle Calculation"
        # "Pull Down Individual Flag"
        n14 = shared-variable "RT myRIO Target - Overlord\\Localization_Variables_r0.lvlib\\RIGHT_BEACON_X_array"() -> (w73:dbl[])  [unwired: 1 in, 1 out]
        "RIGHT Beacon Coord - X px (IN)" <- w73
        n15 = shared-variable "RT myRIO Target - Overlord\\Localization_Variables_r0.lvlib\\Image Lock - R"() -> (w68:bool)  [unwired: 1 in, 1 out]
        n16 = shared-variable "RT myRIO Target - Overlord\\Localization_Variables_r0.lvlib\\RIGHT_BEACON_Scales"() -> (→"Beacon Scales - Right":sgl[])  [unwired: 1 in, 1 out]
        n17 = shared-variable "RT myRIO Target - Overlord\\Localization_Variables_r0.lvlib\\Info - Right"() -> (w65:T6)  [unwired: 1 in, 1 out]
        n18 = shared-variable "RT myRIO Target - Overlord\\Localization_Variables_r0.lvlib\\RIGHT_BEACON_Y_array"() -> (w72:dbl[])  [unwired: 1 in, 1 out]
        "RIGHT Beacon Position - Y px (IN)" <- w72
        n19 = shared-variable "RT myRIO Target - Overlord\\Localization_Variables_r0.lvlib\\RIGHT_BEACON_BOOL_array"() -> (w71:bool[])  [unwired: 1 in, 1 out]
        "Beacons Found\n- Right (Bool Array)" <- w71
        n20 = Unbundle By Name(w65) -> ("Tracking Coordinates"=w64:cluster{"X":dbl, "Y":dbl}, "Current Valid"=w63:bool, "Current Template"=→"Current Template - Right":T1)
        n21 = local write "Image Lock - Right"(w68) -> ()
        n22 = Bundle("Array of Double"=w73, "Array of Double"=w72) -> (w70:T7)  [unwired: 1 in]
        "Beacon Coordinates - Right Image" <- w70
        n23 = shared-variable "RT myRIO Target - Overlord\\Localization_Variables_r0.lvlib\\Right Servo Angle_Image"() -> (w69:dbl)  [unwired: 1 in, 1 out]
        "This Servo \nAngle - Right" <- w69
        n24 = shared-variable "RT myRIO Target - Overlord\\Localization_Variables_r0.lvlib\\RIGHT_FLAG"(FALSE) -> ()  [unwired: 1 in, 1 out]
        n25 = feedback #1() -> (w81:sgl[])  [unwired: 1 in]
        n26 = feedback #2() -> (w80:bool[])  [unwired: 1 in]
        n27 = call "Angle Calc_Individual Process R4.vi"("Angle to Pixel Ratios"=w77, "Previous Angles"=w81, "Num of Beacons"=w79, "Beacon Coordinates - Image"=w70, "Current Servo Angle"=w69, "Beacons Found (Bool Array)"=w71, "Previous Valid Angles"=w80, "Tracking Coordinates"=w64) -> ("Servo Goal Angle"=w76:sgl, "Valid Beacons (Bool Array)\nPosition Calc"=w75:bool[], "Angle Of Beacons \nRelative to Robot"=w74:sgl[])  [unwired: 4 in, 1 out]
        n28 = feedback-in #1(w74) -> ()
        n29 = feedback-in #2(w75) -> ()
        n30 = local write "Tracking Angle - Right"(w76) -> ()
        n31 = local write "Beacon Angles -R"(w74) -> ()
        n32 = local write "Valid Angles -R"(w75) -> ()
        n33 = local write "Track Angle Valid  - Right"(w63) -> ()
        n34 = local write "New Data  Flag\nRight Servo"(w67) -> ()
      }
    }
    "Right Data\nInput Flag\n- Internal" <- w49
    n35 = case shown="True" w52 {
      tunnel: [w82 w88] -> w48
      tunnel: w60 -> [w82 _]
      tunnel: w56 -> [_ w92]
      tunnel: w57 -> [_ w91]
      frame False {
        # "Don't Update Servo Position\nbc we're waiting on new Data to\ncome in and the servo position\nwas set at the previous set of data"
      }
      frame True {
        w88 = TRUE
        # "Store Values"
        # "Raise Internal Flag"
        # "If New Data Available"
        # "Perforrm Indivudual Angle Calculation"
        # "Pull Down Individual Flag"
        n36 = shared-variable ".\\Localization_Variables_r0.lvlib\\LEFT_BEACON_X_array"() -> (w98:dbl[])  [unwired: 1 in, 1 out]
        "LEFT Beacon Coord - X px (IN) 2" <- w98
        n37 = shared-variable "RT myRIO Target - Overlord\\Localization_Variables_r0.lvlib\\LEFT_BEACON_Scales"() -> (→"Beacon Scales - Left":sgl[])  [unwired: 1 in, 1 out]
        n38 = shared-variable "RT myRIO Target - Overlord\\Localization_Variables_r0.lvlib\\LEFT_BEACON_Y_array"() -> (w99:dbl[])  [unwired: 1 in, 1 out]
        "LEFT Beacon Position - Y px (IN) 2" <- w99
        n39 = shared-variable "RT myRIO Target - Overlord\\Localization_Variables_r0.lvlib\\LEFT_BEACON_BOOL_array"() -> (w100:bool[])  [unwired: 1 in, 1 out]
        "Beacons Found\n- Left (Bool Array) 2" <- w100
        n40 = shared-variable "RT myRIO Target - Overlord\\Localization_Variables_r0.lvlib\\Image Lock - L"() -> (w89:bool)  [unwired: 1 in, 1 out]
        n41 = shared-variable "RT myRIO Target - Overlord\\Localization_Variables_r0.lvlib\\Info - Left"() -> (w86:T6)  [unwired: 1 in, 1 out]
        n42 = Unbundle By Name(w86) -> ("Tracking Coordinates"=w85:cluster{"X":dbl, "Y":dbl}, "Current Valid"=w84:bool, "Current Template"=→"Current Template - Left":T1)
        n43 = local write "Image Lock - Left"(w89) -> ()
        n44 = Bundle("Array of Double"=w98, "Array of Double"=w99) -> (w96:T7)  [unwired: 1 in]
        "Beacon Coordinates - Left Image" <- w96
        n45 = shared-variable "RT myRIO Target - Overlord\\Localization_Variables_r0.lvlib\\Left Servo Angle_Image"() -> (w90:dbl)  [unwired: 1 in, 1 out]
        "This Servo \nAngle - Left" <- w90
        n46 = shared-variable "RT myRIO Target - Overlord\\Localization_Variables_r0.lvlib\\Left_Flag"(FALSE) -> ()  [unwired: 1 in, 1 out]
        n47 = feedback #3() -> (w102:sgl[])  [unwired: 1 in]
        n48 = feedback #4() -> (w101:bool[])  [unwired: 1 in]
        n49 = call "Angle Calc_Individual Process R4.vi"("Angle to Pixel Ratios"=w92, "Previous Angles"=w102, "Num of Beacons"=w91, "Beacon Coordinates - Image"=w96, "Current Servo Angle"=w90, "Beacons Found (Bool Array)"=w100, "Previous Valid Angles"=w101, "Tracking Coordinates"=w85) -> ("Servo Goal Angle"=w95:sgl, "Valid Beacons (Bool Array)\nPosition Calc"=w94:bool[], "Angle Of Beacons \nRelative to Robot"=w93:sgl[])  [unwired: 4 in, 1 out]
        n50 = feedback-in #3(w93) -> ()
        n51 = feedback-in #4(w94) -> ()
        n52 = local write "Beacon Angles - L"(w93) -> ()
        n53 = local write "Valid Angles - L"(w94) -> ()
        n54 = local write "Tracking Angle - Left"(w95) -> ()
        n55 = local write "Track Angle Valid - Left"(w84) -> ()
        n56 = local write "New Data  Flag\nLeft Servo"(w88) -> ()
      }
    }
    "Left Data\nInput Flag\n- Internal" <- w48
    n57 = And(x=w48, y=w49) -> (x .and. y?=w59:bool)
    n58 = case shown="True" w59 {
      selector: w59 -> [_ w105]
      tunnel: w48 -> [w104 _]
      tunnel: [w104 w106] -> w55
      tunnel: [w103 w106] -> w54
      tunnel: w49 -> [w103 _]
      frame False {
      }
      frame True {
        w106 = FALSE
        # "Reset Internal Data Flags"
        # "Position Data\nReady Enabled"
        n59 = local write "Position Calc\nReady"(w105) -> ()
      }
    }
  }
  n60 = Bundle(w34, w34) -> (w37:cluster{sgl, sgl})  [unwired: 1 in]
  n61 = Initialize Array(w34, "History Size") -> (w32:sgl[])
  n62 = Initialize Array(w37, "History Size") -> (w33:cluster{sgl, sgl}[])
  n63 = Initialize Array(FALSE, "History Size") -> (w31:bool[])
  n64 = call "Tick Count4"() -> ("Tick Count(uSec)"=w30:u32)
  n65 = while {
    shift-right: [w117] -> _
    shift-left: w32 -> [w114]
    shift-right: [w116] -> _
    shift-left: w31 -> [w115]
    shift-right: [w118] -> _
    shift-left: w33 -> [w109]
    shift-right: [w110] -> _
    shift-left: w30 -> [w111]
    stop <- "stop" stop-if-true
    n66 = call "Wait5"("Count(mSec)"="Position Calc\nTimer") -> ()  [unwired: 1 out]
    n67 = case shown="True" "Position Calc\nReady" {
      selector: "Position Calc\nReady" -> [_ w209]
      tunnel: w109 -> [_ w227]
      tunnel: w109 -> [w127 w222]
      tunnel: w114 -> [w129 w221]
      tunnel: w115 -> [w128 w220]
      tunnel: [w129 w226] -> w117
      tunnel: [w128 w224] -> w116
      tunnel: [w127 w225] -> w118
      tunnel: w115 -> [_ w219]
      tunnel: w114 -> [_ w218]
      tunnel: [w126 w214] -> w112
      tunnel: w111 -> [_ w214]
      tunnel: [FALSE TRUE] -> w113
      tunnel: w109 -> [_ w211]
      frame False {
        n68 = call "Tick Count5"() -> ("Tick Count(uSec)"=w126:u32)
      }
      frame True {
        w147 = 0.0 ("y")
        # "***************************"
        # "dY"
        # "dX"
        # "Valid"
        # "Find Local Coordinates"
        # "Valid COunt"
        # "Make sure 2+ Data Sets are Still available"
        # "Check 1st element\nwith rest of elements"
        # "Make Sure all Pointed \nIn Same Direction"
        # "For Each Valid Beacon\nCalculate Distance from Each Camera to Each Beacon"
        # "Find Common Beacons\nAmong Cameras"
        # "Currently will only\ncalculate position if 2+ \nbeacons are available \nfrom both cameras"
        # "System is in Normal (long range) State"
        # "Average Both Data Sets"
        # "Estimate Distance for each Available Beacon Angle\nPER Camera, indivduallly"
        # "At least 2+ Avaialbe"
        # "CALCULATE AVERAGE ORIENTATION"
        # "Update Outputs\nif Current Calc is Invalid\n(shouldn't matter)"
        # "Estimate Orienation Based on Previous Position"
        # "****# of previous in history that must be true\nin order for position to be considered \"locked\""
        # "New Position is Valid if both \nOrientation and Positions\nis within range of previous"
        # "Robot Position\n Shift Array"
        # "Position Valid Shift Array"
        # "Orientation Shift Array"
        # "Orientation Value"
        # "Shift & Insert Current Position Valid"
        # "Position Valid\n(orientation)"
        # "Position Valid\n(position)"
        # "Update Shift Registers"
        # "Shift & Insert Current Calculated Orientation"
        # "Shift & Insert Current Robot Position"
        # "UPDATE FINAL OUTPUT\n VALUES"
        n69 = local read "Num of Beacons (Total)"() -> (w192:i8)
        n70 = Not(x=w209) -> (.not. x?=w210:bool)
        n71 = local write "Position Calc\nReady"(w210) -> ()
        n72 = disable-structure shown="Disabled" {
          frame Disabled {
            w274 = T8."Normal - 5" ("Initial State")
            # "***********do for both"
            # "sTATE"
            n73 = local read item#-1() -> (w278)
            n74 = local read item#-1() -> (w277)
            n75 = Equal?(x=w278, y=w274) -> (x = y?=w276:bool)
            n76 = Equal?(x=w277, y=w274) -> (x = y?=w275:bool)
            n77 = And(x=w276, y=w275) -> ()  [unwired: 1 out]
          }
          frame Enabled {
          }
        }
        n78 = local read "Current Template - Left"() -> (w151:T1)
        n79 = local read "Current Template - Right"() -> (w150:T1)
        n80 = local read "Beacon Scales - Left"() -> (w198:sgl[])
        n81 = local read "Beacon Scales - Right"() -> (w195:sgl[])
        n82 = for {
          N: w192 -> [_]
          tunnel: "Valid Angles - L" -> [w412] mode=indexing
          tunnel: "Beacon Angles - L" -> [w419] mode=indexing
          tunnel: w198 -> [w420] mode=indexing
          tunnel: "Valid Angles -R" -> [w405] mode=indexing
          tunnel: "Beacon Angles -R" -> [w418] mode=indexing
          tunnel: w195 -> [w417] mode=indexing
          tunnel: "Distance Between \nCameras  (*unit)" -> [w416]
          tunnel: [w411] -> w189 mode=indexing
          tunnel: [w410] -> w188 mode=indexing
          tunnel: [w409] -> w190 mode=indexing
          tunnel: [w408] -> w155 mode=indexing
          tunnel: [w407] -> w154 mode=indexing
          tunnel: [w406] -> w153 mode=indexing
          tunnel: w151 -> [w404]
          tunnel: w150 -> [w403]
          # "dY"
          # "dX"
          # "Valid"
          # "If Both Cameras are using Same Beacon Data,\nAverage the 2 independently esitmated positions"
          # "dY"
          # "dX"
          # "dY"
          # "dX"
          n83 = case shown="True" w412 {
            tunnel: w419 -> [_ w497]
            tunnel: [w484 w488] -> w414
            tunnel: [w484 w489] -> w413
            tunnel: w420 -> [_ w487]
            tunnel: w404 -> [_ w486]
            frame False {
              w484 = sgl 0.0
              # "Current Data Set Was Not Valid\nFill with 0\nWill not be used later"
            }
            frame True {
              # "Estimate Distance"
              # "Negate dX if A2>90"
              # "Find LOCAL Coordinate of Each Beacon"
              # "Current - Valid Data Set"
              n84 = call "Beacon_Scale_to_Distance_R0.vi"("Scale - In"=w487, "Current Template - In"=w486) -> ("Distance - Out"=w485:sgl)  [unwired: 9 in]
              n85 = Less?(x=w497, y=sgl 90.0) -> (x < y?=w499:bool)
              n86 = case shown="False" w499 {
                tunnel: w497 -> [w506 w508]
                tunnel: [w504 w509] -> w496
                tunnel: [FALSE TRUE] -> w491
                frame False {
                  # "Negative Y"
                  # "A2 is > 90"
                  n87 = Subtract(x=w506, y=sgl 90.0) -> (x-y=w504:sgl)
                }
                frame True {
                  # "Positive Y"
                  # "A2 is < 90"
                  n88 = Subtract(x=sgl 90.0, y=w508) -> (x-y=w509:sgl)
                }
              }
              "dA2 2" <- w496
              n89 = expression code="(x/180.0)*pi" "degrees to radians"(w496) -> (w494:sgl)
              n90 = expression code="(x/180.0)*pi" "degrees to radians"(w496) -> (w495:sgl)
              n91 = Cosine(x=w494) -> (cos(x)=w492:sgl)
              n92 = Sine(x=w495) -> (sin(x)=w493:sgl)
              n93 = Multiply(x=w485, y=w492) -> (x*y=w489:sgl)
              n94 = Multiply(x=w485, y=w493) -> (x*y=w490:sgl)
              n95 = case shown="True" w491 {
                tunnel: w490 -> [w501 w502]
                tunnel: [w500 w502] -> w488
                frame False {
                  n96 = Negate(x=w501) -> (-x=w500:sgl)
                }
                frame True {
                }
              }
            }
          }
          n97 = case shown="True" w405 {
            tunnel: w418 -> [_ w470]
            tunnel: [w455 w461] -> w407
            tunnel: [w455 w460] -> w408
            tunnel: w417 -> [_ w457]
            tunnel: w416 -> [_ w462]
            tunnel: [w455 w459] -> w406
            tunnel: w403 -> [_ w458]
            frame False {
              w455 = sgl 0.0
              # "Current Data Set Was Not Valid\nFill with 0\nWill not be used later"
            }
            frame True {
              # "Add delta for\nRIGHT camera ONLY"
              # "Estimate Distance"
              # "Negate dX if A2>90"
              # "Find LOCAL Coordinate of Each Beacon"
              # "Current - Valid Data Set"
              n98 = call "Beacon_Scale_to_Distance_R0.vi"("Scale - In"=w457, "Current Template - In"=w458) -> ("Distance - Out"=w456:sgl)  [unwired: 9 in]
              n99 = Less?(x=w470, y=sgl 90.0) -> (x < y?=w472:bool)
              n100 = case shown="False" w472 {
                tunnel: w470 -> [w479 w481]
                tunnel: [w477 w482] -> w469
                tunnel: [FALSE TRUE] -> w464
                frame False {
                  # "Negative Y"
                  # "A2 is > 90"
                  n101 = Subtract(x=w479, y=sgl 90.0) -> (x-y=w477:sgl)
                }
                frame True {
                  # "Positive Y"
                  # "A2 is < 90"
                  n102 = Subtract(x=sgl 90.0, y=w481) -> (x-y=w482:sgl)
                }
              }
              "dA2 3" <- w469
              n103 = expression code="(x/180.0)*pi" "degrees to radians"(w469) -> (w467:sgl)
              n104 = expression code="(x/180.0)*pi" "degrees to radians"(w469) -> (w468:sgl)
              n105 = Cosine(x=w467) -> (cos(x)=w465:sgl)
              n106 = Sine(x=w468) -> (sin(x)=w466:sgl)
              n107 = Multiply(x=w456, y=w465) -> (x*y=w460:sgl)
              n108 = Multiply(x=w456, y=w466) -> (x*y=w463:sgl)
              n109 = case shown="True" w464 {
                tunnel: w463 -> [w474 w475]
                tunnel: [w473 w475] -> w459
                frame False {
                  n110 = Negate(x=w474) -> (-x=w473:sgl)
                }
                frame True {
                }
              }
              n111 = Add(x=w462, y=w459) -> (x+y=w461:sgl)
            }
          }
          n112 = And(x=w412, y=w405) -> (x .and. y?=w415:bool)
          n113 = case shown="False" w415 {
            tunnel: w414 -> [w428 w454]
            tunnel: w413 -> [w425 w453]
            tunnel: w407 -> [w427 w452]
            tunnel: w408 -> [w426 w451]
            tunnel: [w423 w447] -> w411
            tunnel: [w422 w446] -> w410
            tunnel: w412 -> [w424 _]
            tunnel: w405 -> [w429 _]
            tunnel: [w421 TRUE] -> w409
            frame False {
              n114 = Exclusive Or(1:w429, 2:w424) -> (0:w430:bool)
              n115 = case shown="True" w430 {
                tunnel: w428 -> [_ w438]
                tunnel: w427 -> [_ w435]
                tunnel: w426 -> [_ w434]
                tunnel: w425 -> [_ w436]
                tunnel: w424 -> [_ w440]
                tunnel: [w431 w439] -> w423
                tunnel: [w431 w437] -> w422
                tunnel: [FALSE TRUE] -> w421
                frame False {
                  w431 = sgl 0.0
                  # "None are valid,"
                }
                frame True {
                  # "Only 1 beacon is valid,\nUse the valid beacon"
                  n116 = case shown="False" w440 {
                    tunnel: [w442 w444] -> w439
                    tunnel: w438 -> [_ w444]
                    tunnel: [w441 w443] -> w437
                    tunnel: w436 -> [_ w443]
                    tunnel: w435 -> [w442 _]
                    tunnel: w434 -> [w441 _]
                    frame False {
                      # "Left is invalid,\nRight MUST be valid"
                    }
                    frame True {
                      # "Left is Valid"
                    }
                  }
                }
              }
            }
            frame True {
              w448 = sgl 2.0 ("y")
              # "Both are Valid"
              n117 = Add(x=w454, y=w452) -> (x+y=w449:sgl)
              n118 = Add(x=w453, y=w451) -> (x+y=w450:sgl)
              n119 = Divide(x=w450, y=w448) -> (x/y=w446:sgl)
              n120 = Divide(x=w449, y=w448) -> (x/y=w447:sgl)
            }
          }
        }
        "Array" <- w155
        "Array 2" <- w154
        "Array 3" <- w153
        n121 = And(x="Valid Angles - L", y="Valid Angles -R") -> (x .and. y?=w180:bool[])
        n122 = Boolean To (0,1)(Boolean=w180) -> (0, 1=w177:i16[])
        n123 = Add Array Elements(numeric array=w177) -> (sum=w178:i16)
        n124 = Greater?(x=w178, y=1) -> (0:w176:bool)
        n125 = for {
          N: w192 -> [_]
          tunnel: w176 -> [w339]
          tunnel: "Beacon Angles - L" -> [w338] mode=indexing
          tunnel: "Beacon Angles -R" -> [w337] mode=indexing
          tunnel: "Distance Between \nCameras  (*unit)" -> [w336]
          tunnel: "Distance Threshold\nRef Triangles (*unit)" -> [w335]
          tunnel: [w334] -> w163 mode=indexing
          tunnel: [w333] -> _ mode=indexing
          tunnel: [w332] -> w162 mode=indexing
          tunnel: [w331] -> _ mode=indexing
          tunnel: [w330] -> w164 mode=indexing
          tunnel: [w329] -> w170 mode=indexing
          n126 = case shown="True" w339 {
            tunnel: w338 -> [w344 w354]
            tunnel: w337 -> [w343 w353]
            tunnel: w336 -> [_ w345]
            tunnel: w335 -> [_ w346]
            tunnel: [w344 w352] -> w334
            tunnel: [w343 w351] -> w333
            tunnel: [FALSE w350] -> w332
            tunnel: [w341 w349] -> w331
            tunnel: [w341 w348] -> w330
            tunnel: [0 w347] -> w329
            frame False {
              w341 = sgl 1.0
            }
            frame True {
              # "Build Reference Triangle"
              n127 = call "Position Calc_Build Reference Triangle_R1.vi"("A2_in"=w354, "A3_in"=w353, "S1 (Length Between\n Cameras - inches)"=w345, "Distance\nThreshold"=w346) -> ("S2"=w349:sgl, "S3"=w348:sgl, "Direction"=w347:i8, "A2"=w352:sgl, "A3"=w351:sgl, "Accept"=w350:bool)  [unwired: 6 in]
            }
          }
        }
        n128 = for {
          N: w192 -> [_]
          tunnel: w162 -> [w324] mode=indexing
          tunnel: w170 -> [w328] mode=indexing
          tunnel: [w328] -> w172 mode=indexing if=w324
          shift-right: [w327] -> w166
          shift-left: 0 -> [w325]
          # "Only add to array\nif valid distance"
          n129 = Increment(x=w325) -> (x+1=w326:i32)
          n130 = Select(t=w326, s=w324, f=w325) -> (s? t:f=w327:i32)
        }
        n131 = Index Array(array=w172, index=0) -> (element=w173:i32)
        n132 = Equal?(x=w172, y=w173) -> (x = y?=w174:bool[])
        n133 = And Array Elements(Boolean array=w174) -> (logical AND=w168:bool)
        n134 = Greater?(x=w166, y=1) -> (0:w167:bool)
        n135 = And(x=w168, y=w167) -> (x .and. y?=w161:bool)
        n136 = case shown="True" w161 {
          tunnel: w192 -> [w281 w290]
          tunnel: w164 -> [_ w289]
          tunnel: w163 -> [_ w288]
          tunnel: w162 -> [_ w287]
          tunnel: [w280 w286] -> w191
          tunnel: [w279 w285] -> w187
          tunnel: [w279 w284] -> w186
          frame False {
            # "Build Array for False"
            n137 = for {
              N: w281 -> [_]
              tunnel: [sgl 0.0] -> w279 mode=indexing
              tunnel: [FALSE] -> w280 mode=indexing
            }
          }
          frame True {
            n138 = for {
              N: w290 -> [_]
              tunnel: w288 -> [w296] mode=indexing
              tunnel: w289 -> [w295] mode=indexing
              tunnel: [w294] -> w285 mode=indexing
              tunnel: [w293] -> w284 mode=indexing
              tunnel: [w292] -> w286 mode=indexing
              tunnel: w287 -> [w291] mode=indexing
              n139 = case shown="True" w291 {
                selector: w291 -> [w298 w302]
                tunnel: w296 -> [_ w310]
                tunnel: [w297 w300] -> w294
                tunnel: [w297 w301] -> w293
                tunnel: w295 -> [_ w299]
                tunnel: [w298 w302] -> w292
                frame False {
                  w297 = sgl 0.0
                  # "Current Data Set Was Not Valid\nFill with 0\nWill not be used later"
                }
                frame True {
                  # "dY"
                  # "dX"
                  # "Negate dX if A2>90"
                  # "Find LOCAL Coordinate of Each Beacon"
                  # "Current - Valid Data Set"
                  n140 = Less?(x=w310, y=sgl 90.0) -> (x < y?=w312:bool)
                  n141 = case shown="False" w312 {
                    tunnel: w310 -> [w319 w321]
                    tunnel: [w317 w322] -> w309
                    tunnel: [FALSE TRUE] -> w304
                    frame False {
                      # "Negative Y"
                      # "A2 is > 90"
                      n142 = Subtract(x=w319, y=sgl 90.0) -> (x-y=w317:sgl)
                    }
                    frame True {
                      # "Positive Y"
                      # "A2 is < 90"
                      n143 = Subtract(x=sgl 90.0, y=w321) -> (x-y=w322:sgl)
                    }
                  }
                  "dA2 4" <- w309
                  n144 = expression code="(x/180.0)*pi" "degrees to radians"(w309) -> (w307:sgl)
                  n145 = expression code="(x/180.0)*pi" "degrees to radians"(w309) -> (w308:sgl)
                  n146 = Cosine(x=w307) -> (cos(x)=w305:sgl)
                  n147 = Sine(x=w308) -> (sin(x)=w306:sgl)
                  n148 = Multiply(x=w299, y=w305) -> (x*y=w301:sgl)
                  n149 = Multiply(x=w299, y=w306) -> (x*y=w303:sgl)
                  n150 = case shown="True" w304 {
                    tunnel: w303 -> [w314 w315]
                    tunnel: [w313 w315] -> w300
                    frame False {
                      n151 = Negate(x=w314) -> (-x=w313:sgl)
                    }
                    frame True {
                    }
                  }
                }
              }
            }
          }
        }
        n152 = Subtract(x=sgl 1.0, y="Triangle Based\nWeight") -> (x-y=w183:sgl)
        "Scale Based\nWeight" <- w183
        n153 = for {
          N: w192 -> [_]
          tunnel: w191 -> [w359] mode=indexing
          tunnel: w190 -> [w358] mode=indexing
          tunnel: w189 -> [w363] mode=indexing
          tunnel: w188 -> [w362] mode=indexing
          tunnel: w187 -> [w365] mode=indexing
          tunnel: w186 -> [w364] mode=indexing
          tunnel: "Triangle Based\nWeight" -> [w361]
          tunnel: w183 -> [w360]
          tunnel: [w357] -> w160 mode=indexing
          tunnel: [w356] -> w182 mode=indexing
          tunnel: [w355] -> w181 mode=indexing
          # "If Beacon info \nis available from\nboth"
          n154 = And(x=w359, y=w358) -> (x .and. y?=w366:bool)
          n155 = case shown="True" w366 {
            selector: w366 -> [_ w392]
            tunnel: w365 -> [w373 w400]
            tunnel: w364 -> [w371 w401]
            tunnel: w363 -> [w369 w399]
            tunnel: w362 -> [w368 w398]
            tunnel: w361 -> [_ w402]
            tunnel: w360 -> [_ w397]
            tunnel: [w372 w390] -> w355
            tunnel: [w374 w391] -> w356
            tunnel: w359 -> [w375 _]
            tunnel: w358 -> [w370 _]
            tunnel: [w367 w392] -> w357
            frame False {
              n156 = case shown="False" w375 {
                selector: w375 -> [_ w387]
                tunnel: [w380 w389] -> w374
                tunnel: w373 -> [_ w389]
                tunnel: [w378 w388] -> w372
                tunnel: w371 -> [_ w388]
                tunnel: w370 -> [w381 _]
                tunnel: w369 -> [w379 _]
                tunnel: w368 -> [w377 _]
                tunnel: [w376 w387] -> w367
                frame False {
                  n157 = case shown="False" w381 {
                    selector: w381 -> [w382 w384]
                    tunnel: [w383 w386] -> w380
                    tunnel: w379 -> [_ w386]
                    tunnel: [w383 w385] -> w378
                    tunnel: w377 -> [_ w385]
                    tunnel: [w382 w384] -> w376
                    frame False {
                      w383 = sgl 0.0
                      # "None avail"
                    }
                    frame True {
                    }
                  }
                }
                frame True {
                }
              }
            }
            frame True {
              n158 = Multiply(x=w400, y=w402) -> (x*y=w396:sgl)
              n159 = Multiply(x=w401, y=w402) -> (x*y=w394:sgl)
              n160 = Multiply(x=w399, y=w397) -> (x*y=w395:sgl)
              n161 = Multiply(x=w398, y=w397) -> (x*y=w393:sgl)
              n162 = Add(x=w396, y=w395) -> (x+y=w391:sgl)
              n163 = Add(x=w394, y=w393) -> (x+y=w390:sgl)
            }
          }
        }
        "Valid Beacon Sets_" <- w160
        n164 = Boolean To (0,1)(Boolean=w160) -> (0, 1=w203:i16[])
        n165 = Add Array Elements(numeric array=w203) -> (sum=w202:i16)
        n166 = Greater?(x=w202, y=i16 1) -> (0:w200:bool)
        n167 = case shown="True" w200 {
          tunnel: w227 -> [_ w601]
          tunnel: [0.0 ("f") w600] -> w223
          tunnel: [w513 w599] -> w141
          tunnel: w219 -> [_ w520]
          tunnel: w218 -> [_ w598]
          tunnel: [FALSE w597] -> w139
          tunnel: [FALSE w596] -> w137
          tunnel: w211 -> [_ w595]
          tunnel: [sgl 0.0 w593] -> w204
          tunnel: "Distance Between \nCameras  (*unit)" -> [_ w532]
          tunnel: w182 -> [_ w531]
          tunnel: w181 -> [_ w530]
          tunnel: w160 -> [_ w529]
          tunnel: w192 -> [_ w528]
          frame False {
            w512 = 0.0 ("f")
            n168 = Bundle("f"=w512, "f"=w512) -> (w513:cluster{"f":dbl, "f":dbl})  [unwired: 1 in]
          }
          frame True {
            w565 = sgl 2.0
            w582 = 0
            # "Current Orientaiton"
            # "Valid Position Ccount\n(within moving avg\nwinfow)"
            # "Valid Position Ccount"
            # "Only Apply This Filtering \nif 3 or More Beacons Still Valid"
            # "Orientation Value"
            # "Orientation Valid"
            # "Y (current)"
            # "X (current)"
            # "Number of Valid\nPrevious Orientations"
            # "More than 1 Previous\nValid Positions"
            # "More than\n2previous position\navailable"
            # "Choose Beacon Set\nwith Lowest Std Dev"
            # "Y value cannot be negative"
            # "Find New # Of Valid Beacons"
            # "Adjust/Normalize\nLocal Beacon Positions\nusing Line of Best fit"
            # "# Valid\nData Sets"
            # "cam, y"
            # "cam, x"
            # "Calculate dX and dY\nfor right cam"
            # "Average dX and dY from each (valid) beacon to find position of each camera\n\nthen average all  positions for each camera find center between"
            # "Convert Slope\nto Radians"
            # "*rotate CCW in rad"
            # "Rotate Coordinate\n System by Slope"
            n169 = Boolean To (0,1)(Boolean=w520) -> (0, 1=w549:i16[])
            n170 = Initialize Array(u8 0, "Moving Average\nWindow Length") -> (w525:u8[])
            n171 = Add Array Elements(numeric array=w549) -> (sum=w519:i16)
            n172 = Greater?(x=w519, y=0) -> (0:w522:bool)
            n173 = while {
              shift-right: [w603] -> w523
              shift-left: w525 -> [w605]
              tunnel: w520 -> [w610] mode=indexing
              shift-right: [w609] -> w521
              shift-left: u8 0 -> [w611]
              tunnel: "Moving Average\nWindow Length" -> [w602]
              i -> [w604]
              stop <- w606 stop-if-true
              # "Grab Last 2 Valid Position Indexes"
              n174 = case shown="True" w610 {
                tunnel: w611 -> [w613 w615]
                tunnel: [w613 w618] -> w609
                tunnel: w605 -> [w612 w617]
                tunnel: w604 -> [_ w616]
                tunnel: [w612 w614] -> w603
                frame False {
                }
                frame True {
                  # "Update Index\nto use"
                  # "Increment\nValid Count"
                  n175 = Replace Array Subset(array=w617, new element=w616, index=w615) -> (w614:u8[])
                  n176 = Increment(x=w615) -> (x+1=w618:u8)
                }
              }
              n177 = Greater Or Equal?(x=w609, y=w602) -> (x >= y?=w608:bool)
              n178 = Greater Or Equal?(x=w604, y=w602) -> (x >= y?=w607:bool)
              n179 = Or(x=w608, y=w607) -> (x .or. y?=w606:bool)
            }
            n180 = Bundle(w531, w530) -> (→"LOCAL\nBeacon Coordinates\nRelative to Robot" →"Local Coordinates - Calculated":cluster{sgl[], sgl[]})  [unwired: 1 in]
            n181 = call "Coordinate_Outlier_Filtering_R2.vi"("Num of Beacons"=w528, "Max Std Dev(all 5)"="Max Std Dev (5)", "X in"=w531, "Valid Data\nSets in"=w529, "Y in"=w530, "Max Std Dev( 4 )"="Max Std Dev (4)", "Max Std Dev (3)"="Max Std Dev (3)") -> ("Y out"=w542:sgl[], "X out"=w543:sgl[], "Valid Beacons\nout"=w540:bool[], "Slope out"=w548:dbl)  [unwired: 3 in, 2 out]
            n182 = Inverse Tangent(1:w548) -> (0:w561:dbl)
            n183 = expression code="(x/pi)*180.0" "radians to degrees"(w561) -> (w547:dbl)
            n184 = Boolean To (0,1)(Boolean=w540) -> (0, 1=w539:i16[])
            n185 = To Single Precision Float(number=w547) -> (single precision float=w593:sgl)
            n186 = case shown="True" w522 {
              tunnel: [w628 w649] -> w596
              tunnel: w598 -> [_ w651]
              tunnel: w593 -> [w629 w646]
              tunnel: [w627 w650] -> w600
              tunnel: w595 -> [_ _]
              tunnel: w523 -> [_ w647]
              tunnel: w521 -> [_ w638]
              frame False {
                # "Since no history available,\ncheck that current is with 0-360"
                # "Use Current Orientation bc \nPrevious are not available"
                # "New Position\nValid"
                n187 = In Range and Coerce(upper limit=sgl 360.0, x=w629, lower limit=sgl -360.0 ("upper limit")) -> (In Range?=w628:bool)  [unwired: 1 out]
                n188 = Select(t=w629, s=w628, f=sgl 0.0) -> (s? t:f=w627:sgl)
              }
              frame True {
                # "Calculate New, Weighted\nOrientation"
                # "Moving Average Out"
                n189 = local read "Last Position"() -> (w636:cluster{"X":sgl, "Y":sgl})
                n190 = Unbundle By Name(w636) -> ("X"=w633:sgl)
                n191 = call "Scaling and Mapping2"("Signals"=w633) -> ("Scaled Signals"=w635:dynamicdata)  [unwired: 9 in, 1 out]
                n192 = for {
                  N: w638 -> [_]
                  shift-right: [w675] -> w644
                  shift-left: 0.0 -> [w674]
                  tunnel: w647 -> [w673] mode=indexing
                  tunnel: w651 -> [w671]
                  # "Fetch Last Valid Values\nand Sum"
                  n193 = Index Array(array=w671, index=w673) -> (element=w672:sgl)
                  n194 = Add(x=w672, y=w674) -> (x+y=w675:dbl)
                }
                n195 = To Single Precision Float(number=w635) -> (single precision float=w634:sgl)
                "New Orientation\nWeight" <- w634
                n196 = Subtract(x=sgl 1.0, y=w634) -> (x-y=w643:sgl)
                n197 = Multiply(x=w646, y=w634) -> (x*y=w641:sgl)
                n198 = Multiply(x=w643, y=w644) -> (x*y=w639:dbl)
                n199 = To Double Precision Float(number=w638) -> (double precision float=w637:dbl)
                n200 = Divide(x=w639, y=w637) -> (x/y=w640:dbl)
                n201 = Add(x=w641, y=w640) -> (x+y=w642:dbl)
                n202 = Greater Than 0?(x=w638) -> (x > 0?=w648:bool)
                n203 = case shown="True" w648 {
                  tunnel: w642 -> [w655 w661]
                  tunnel: w647 -> [_ w668]
                  tunnel: w651 -> [_ w667]
                  tunnel: [w654 w660] -> w650
                  tunnel: [w653 w663] -> w649
                  frame False {
                    # "No Pevious is Available to Compare\ncheck that current is real angle"
                    n204 = In Range and Coerce(upper limit=sgl 360.0, x=w655, lower limit=sgl -360.0 ("upper limit")) -> (In Range?=w653:bool)  [unwired: 1 out]
                    n205 = Select(t=w655, s=w653, f=sgl 0.0) -> (s? t:f=w654:dbl)
                  }
                  frame True {
                    # "Check That New Value\nis within Range of Old\n(avg)"
                    # "(X1 - X2)^2"
                    # "Previous"
                    # "Pevious is Available to Compare"
                    n206 = Index Array(array=w668, index=u8 0) -> (element=w669:u8)
                    n207 = Index Array(array=w667, index=w669) -> (element=w666:sgl)
                    n208 = Subtract(x=w666, y=w661) -> (x-y=w665:dbl)
                    n209 = Absolute Value(x=w665) -> (abs(x)=w664:dbl)
                    n210 = Less Or Equal?(x=w664, y="New Orientation \nThreshold") -> (x <= y?=w663:bool)
                    n211 = Select(t=w661, s=w663, f=sgl 0.0) -> (s? t:f=w660:dbl)
                  }
                }
              }
            }
            n212 = Add Array Elements(numeric array=w539) -> (sum=w538:i16)
            n213 = Greater?(x=w538, y=i16 2) -> (0:w536:bool)
            n214 = case shown="True" w536 {
              tunnel: w528 -> [_ w626]
              tunnel: w540 -> [w619 w625]
              tunnel: w543 -> [_ w624]
              tunnel: w542 -> [_ w623]
              tunnel: [w619 w622] -> w541
              tunnel: "Distance\nBetween Beacons" -> [_ w621]
              tunnel: "Distance\nBetween Beacons \n- Tolerance" -> [_ w620]
              frame False {
                # "Don't apply filtering,\nnot enough data points"
              }
              frame True {
                # "This will filter beacons if they are calculate to be \ntoo close to each other. The beacon(s) that is\n discarded is chosen based distance between each/every\nbeacon,. Capable of filtering as long as 1/2 of sample\nset has uniform distances (between beacons)."
                # "Validate Distance Between\nEach Beacon"
                n215 = call "Beacon_Filtering_Inter_Beacon_Distance_R1.vi"("Num of Beacons"=w626, "Inter Beacon\nReal Distance"=w621, "X in"=w624, "Inter Beacon\ndelta Threshold"=w620, "Y in"=w623, "Valid Data\nSets in"=w625) -> ("Beacons Valid - Out"=w622:bool[])  [unwired: 9 in]
              }
            }
            "Post Filtering\n- Valid Beacons" <- w541
            n216 = Increment(x=w528) -> (x+1=w583:i8)
            n217 = for {
              N: w583 -> [_]
              tunnel: [w794] -> w584 mode=indexing
              tunnel: w543 -> [w790]
              tunnel: w542 -> [w793]
              tunnel: [w792] -> w585 mode=indexing
              tunnel: w532 -> [w789]
              i -> [w791]
              # "Build Array's of Coordinates\nFor All Objects"
              n218 = Greater Than 0?(x=w791) -> (x > 0?=w795:bool)
              n219 = case shown="True" w795 {
                tunnel: [w797 w803] -> w794
                tunnel: w790 -> [w800 _]
                tunnel: w793 -> [w799 _]
                tunnel: [w796 0.0] -> w792
                tunnel: w791 -> [w801 _]
                tunnel: w789 -> [_ w803]
                frame True {
                  # "Rest of Array is\nBeacon Coordinates"
                  n220 = Decrement(x=w801) -> (x-1=w798:i32)
                  n221 = Index Array(array=w800, index=w798) -> (element=w797:sgl)
                  n222 = Index Array(array=w799, index=w798) -> (element=w796:sgl)
                }
                frame False {
                  # "First object is the\nother Camera\n\nthis coordinate\nis simply:\nx = 0\ny = distance btween cams"
                }
              }
            }
            n223 = Bundle(w584, w585) -> (→"All Object Coordinates \n- Local" →"Local Coordinates - Normalized":cluster{sgl[], dbl[]})  [unwired: 1 in]
            n224 = expression code="(x/180.0)*pi" "degrees to radians"(w600) -> (w546:dbl)
            n225 = call-poly <vilib>:"2D Cartesian Coordinate Rotation.vi"("theta"=w546, "Y"=w585, "X"=w584) -> ("Y Out"=w562:dbl[], "X Out"=w563:dbl[])  [unwired: 6 in, 1 out]
            n226 = Bundle("X Out"=w563, "Y Out"=w562) -> (→"All Object Coordinates \n- Local - Rotated" →"Local Coordinates - Rotated":cluster{"X Out":dbl[], "Y Out":dbl[]})  [unwired: 1 in]
            n227 = Index Array(array=w562, index=w582) -> (element=w558:dbl)
            n228 = Index Array(array=w563, index=w582) -> (element=w581:dbl)
            n229 = for {
              N: w528 -> [_]
              tunnel: w562 -> [w785]
              tunnel: w563 -> [w786]
              tunnel: w581 -> [w784]
              tunnel: w558 -> [w783]
              tunnel: [w782] -> w555 mode=indexing
              tunnel: [w781] -> w554 mode=indexing
              tunnel: [w780] -> w533 mode=indexing
              tunnel: [w779] -> w556 mode=indexing
              i -> [w788]
              n230 = Increment(x=w788) -> (x+1=w787:i32)
              n231 = Index Array(array=w785, index=w787) -> (element=w779:dbl)
              n232 = Index Array(array=w786, index=w787) -> (element=w780:dbl)
              n233 = Subtract(x=w779, y=w783) -> (x-y=w781:dbl)
              n234 = Subtract(x=w780, y=w784) -> (x-y=w782:dbl)
            }
            n235 = Bundle(w555, w554) -> (→"dX, dY\nRight Cam":cluster{dbl[], dbl[]})  [unwired: 1 in]
            n236 = Bundle(w533, w556) -> (→"dX, dY\nLeft Cam":cluster{dbl[], dbl[]})  [unwired: 1 in]
            n237 = Unbundle("Real Beacon\n - Coordinates") -> ("X"=w579:dbl[], "Y"=w559:dbl[])
            n238 = Boolean To (0,1)(Boolean=w541) -> (0, 1=w557:i16[])
            n239 = for {
              N: w528 -> [_]
              tunnel: w541 -> [w765] mode=indexing
              tunnel: w579 -> [w762] mode=indexing
              tunnel: w559 -> [w761] mode=indexing
              tunnel: w533 -> [w764] mode=indexing
              tunnel: w556 -> [w760] mode=indexing
              tunnel: w555 -> [w763] mode=indexing
              tunnel: w554 -> [w759] mode=indexing
              tunnel: [w758] -> w578 mode=indexing
              tunnel: [w757] -> w577 mode=indexing
              tunnel: [w756] -> w576 mode=indexing
              tunnel: [w755] -> w575 mode=indexing
              n240 = case shown="True" w765 {
                tunnel: w764 -> [_ w778]
                tunnel: w763 -> [_ w777]
                tunnel: w762 -> [_ w768]
                tunnel: w761 -> [_ w767]
                tunnel: w760 -> [_ w776]
                tunnel: w759 -> [_ w769]
                tunnel: [w766 w774] -> w758
                tunnel: [w766 w773] -> w757
                tunnel: [w766 w772] -> w756
                tunnel: [w766 w771] -> w755
                frame False {
                  w766 = sgl 0.0
                  # "Add Nothing"
                }
                frame True {
                  # "realX = beaconX + dY\nrealY = beaconY + (-dx)"
                  # "Right Cam"
                  # "Left Cam"
                  # "dX = -dX\nSwap dX, dY"
                  # "Translate to Real Coordinates\nOnly Apply for Valid Beacons"
                  n241 = Negate(x=w778) -> (-x=w775:dbl)
                  n242 = Negate(x=w777) -> (-x=w770:dbl)
                  n243 = Add(x=w768, y=w776) -> (x+y=w774:dbl)
                  n244 = Add(x=w767, y=w775) -> (x+y=w773:dbl)
                  n245 = Add(x=w768, y=w769) -> (x+y=w772:dbl)
                  n246 = Add(x=w767, y=w770) -> (x+y=w771:dbl)
                }
              }
            }
            n247 = Add Array Elements(numeric array=w557) -> (sum=w560:i16)
            n248 = Add Array Elements(numeric array=w578) -> (sum=w574:dbl)
            n249 = Add Array Elements(numeric array=w577) -> (sum=w573:dbl)
            n250 = Add Array Elements(numeric array=w576) -> (sum=w572:dbl)
            n251 = Add Array Elements(numeric array=w575) -> (sum=w571:dbl)
            n252 = Divide(x=w574, y=w560) -> (x/y=w570:dbl)
            n253 = Divide(x=w573, y=w560) -> (x/y=w568:dbl)
            n254 = Divide(x=w572, y=w560) -> (x/y=w569:dbl)
            n255 = Divide(x=w571, y=w560) -> (x/y=w567:dbl)
            n256 = Bundle(w570, w568) -> (→"Left Camera Real Coordinates":cluster{dbl, dbl})  [unwired: 1 in]
            n257 = Bundle(w569, w567) -> (→"Right Camera Real Coordinate":cluster{dbl, dbl})  [unwired: 1 in]
            n258 = Add(x=w570, y=w569) -> (x+y=w566:dbl)
            n259 = Add(x=w568, y=w567) -> (x+y=w564:dbl)
            n260 = Divide(x=w566, y=w565) -> (x/y=w517:dbl)
            n261 = Divide(x=w564, y=w565) -> (x/y=w518:dbl)
            n262 = Bundle(w517, w518) -> (→"Robot Coordinates":cluster{dbl, dbl})  [unwired: 1 in]
            n263 = Less Than 0?(x=w518) -> ()  [unwired: 1 out]
            n264 = case shown="True" w522 {
              tunnel: w519 -> [_ _]
              tunnel: w517 -> [w680 w704]
              tunnel: [w681 w714] -> w597
              tunnel: w601 -> [_ w708]
              tunnel: w518 -> [w679 w691]
              tunnel: [w678 w718] -> w599
              tunnel: "Max X (arena)" -> [w677 w713]
              tunnel: "Max Y (arena)" -> [w676 w712]
              tunnel: w523 -> [_ w710]
              tunnel: w521 -> [_ w709]
              frame False {
                # "New Position\nValid"
                # "Since no history available,\ncheck that current is within\nthe bounds of the arena size"
                # "Use Current Position bc \nPrevious are not available"
                n265 = In Range and Coerce(upper limit=w677, x=w680, lower limit=sgl 0.0 ("upper limit")) -> (In Range?=w683:bool)  [unwired: 1 out]
                n266 = In Range and Coerce(upper limit=w676, x=w679, lower limit=sgl 0.0 ("upper limit")) -> (In Range?=w682:bool)  [unwired: 1 out]
                n267 = Bundle(w680, w679) -> (w678:cluster{dbl, dbl})  [unwired: 1 in]
                n268 = And(x=w683, y=w682) -> (x .and. y?=w681:bool)
              }
              frame True {
                w711 = 0.0
                # "Change Y weight depending\non previous X position in course"
                # "If needed, make seperate FOR Loop for \nY only... Using more previous values than X"
                # "New Y"
                # "New X"
                # "Only consider if velocity is\ngreater than certain speed"
                # "Weighted Robot \nCoordinates"
                # "Position\nValid\n(current)"
                n269 = local read "Last Position"() -> (w689:cluster{"X":sgl, "Y":sgl})
                n270 = Unbundle By Name(w689) -> ("X"=w688:sgl)
                n271 = for {
                  N: w709 -> [_]
                  shift-right: [w727] -> w707
                  shift-left: w711 -> [w726]
                  shift-right: [w725] -> w692
                  shift-left: w711 -> [w724]
                  tunnel: w710 -> [w722] mode=indexing
                  tunnel: w708 -> [w720]
                  # "Fetch Last Valid Values\nand Sum"
                  n272 = Index Array(array=w720, index=w722) -> (element=w721:cluster{sgl, sgl})
                  n273 = Unbundle(w721) -> (w723:sgl, w719:sgl)
                  n274 = Add(x=w719, y=w724) -> (x+y=w725:dbl)
                  n275 = Add(x=w723, y=w726) -> (x+y=w727:dbl)
                }
                n276 = call "Scaling and Mapping"("Signals"=w688) -> ("Scaled Signals"=w687:dynamicdata)  [unwired: 9 in, 1 out]
                n277 = To Single Precision Float(number=w687) -> (single precision float=w686:sgl)
                "New Position\nWeight (Y coord)" <- w686
                n278 = Subtract(x=sgl 1.0, y="New Position\nWeight (X coord)") -> (x-y=w706:sgl)
                n279 = Subtract(x=sgl 1.0, y=w686) -> (x-y=w690:sgl)
                n280 = To Single Precision Float(number=w709) -> (single precision float=w698:sgl)
                n281 = Multiply(x=w706, y=w707) -> (x*y=w699:dbl)
                n282 = Multiply(x=w692, y=w690) -> (x*y=w700:dbl)
                n283 = Divide(x=w699, y=w698) -> (x/y=w696:dbl)
                n284 = Divide(x=w700, y=w698) -> (x/y=w697:dbl)
                n285 = Multiply(x="New Position\nWeight (X coord)", y=w704) -> (x*y=w702:dbl)
                n286 = Multiply(x=w691, y=w686) -> (x*y=w701:dbl)
                n287 = Add(x=w702, y=w696) -> (x+y=w695:dbl)
                n288 = Add(x=w701, y=w697) -> (x+y=w694:dbl)
                n289 = Greater Than 0?(x=w709) -> (x > 0?=w717:bool)
                n290 = case shown="True" w717 {
                  tunnel: w695 -> [w732 w739]
                  tunnel: w694 -> [w731 w738]
                  tunnel: w710 -> [_ w751]
                  tunnel: w708 -> [_ w750]
                  tunnel: [w729 w739] -> w716
                  tunnel: [w728 w738] -> w715
                  tunnel: [w733 w740] -> w714
                  tunnel: w713 -> [w735 _]
                  tunnel: w712 -> [w734 _]
                  frame False {
                    w730 = sgl 0.0 ("upper limit")
                    # "Check that within bounds of arena"
                    # "No Pevious is Available to Compare"
                    n291 = In Range and Coerce(upper limit=w735, x=w732, lower limit=w730) -> (In Range?=w737:bool)  [unwired: 1 out]
                    n292 = In Range and Coerce(upper limit=w734, x=w731, lower limit=w730) -> (In Range?=w736:bool)  [unwired: 1 out]
                    n293 = And(x=w737, y=w736) -> (x .and. y?=w733:bool)
                    n294 = Select(t=w732, s=w733, f=w730) -> (s? t:f=w729:dbl)
                    n295 = Select(t=w731, s=w733, f=w730) -> (s? t:f=w728:dbl)
                  }
                  frame True {
                    # "New"
                    # "(Y1 - Y2)^2"
                    # "(X1 - X2)^2"
                    # "Previous"
                    # "Pevious is Available to Compare"
                    n296 = Index Array(array=w751, index=u8 0) -> (element=w753:u8)
                    n297 = Index Array(array=w750, index=w753) -> (element=w752:cluster{sgl, sgl})
                    n298 = Unbundle(w752) -> (w742:sgl, w741:sgl)
                    n299 = Subtract(x=w742, y=w739) -> (x-y=w747:dbl)
                    n300 = Subtract(x=w738, y=w741) -> (x-y=w746:dbl)
                    n301 = Square(x=w747) -> (x^2=w745:dbl)
                    n302 = Square(x=w746) -> (x^2=w744:dbl)
                    n303 = Add(x=w745, y=w744) -> (x+y=w748:dbl)
                    n304 = Square Root(x=w748) -> (sqrt(x)=w743:dbl)
                    n305 = Less Or Equal?(x=w743, y="New Position \nThreshold") -> (x <= y?=w740:bool)
                  }
                }
                n306 = Bundle("upper limit"=w716, "upper limit"=w715) -> (w718:cluster{"upper limit":dbl, "upper limit":dbl})  [unwired: 1 in]
              }
            }
          }
        }
        "Orietnation\n(current)" <- w204
        n307 = local read "Current Template - Left"() -> (w135:T1)
        n308 = local read "Current Template - Left"() -> (w133:T1)
        n309 = Equal?(x=w135, y=w133) -> (x = y?=w131:bool)
        n310 = Equal?(x=w133, y=T1."Range 0" ("Current Template - Left")) -> (x = y?=w130:bool)
        n311 = And(x=w131, y=w130) -> (x .and. y?=w132:bool)
        n312 = case shown="False" w132 {
          tunnel: [w230 w248] -> w138
          tunnel: [w229 w247] -> w136
          tunnel: w139 -> [w230 _]
          tunnel: w137 -> [w229 _]
          tunnel: [w228 w244] -> w140
          tunnel: w141 -> [w228 _]
          frame False {
            # "Disabled  -- ignore and pass all values thru"
          }
          frame True {
            w256 = 0 ("index")
            # "At Least 1?"
            # "# valid (0,1,2)"
            # "Only Stores in index\n0 for this special case"
            # "Curve Fitting for Range 0"
            # "Latch Y position"
            n313 = local read "Beacons Found\n- Left (Bool Array) 2"() -> (w265:bool[])
            n314 = local read "Beacons Found\n- Right (Bool Array)"() -> (w266:bool[])
            n315 = local read "Beacon Scales - Right"() -> (w257:sgl[])
            n316 = local read "Beacon Scales - Left"() -> (w258:sgl[])
            n317 = Index Array(array=w265, index=w256) -> (element=w264:bool)
            n318 = Index Array(array=w266, index=w256) -> (element=w259:bool)
            n319 = Index Array(array=w258, index=w256) -> (element=w237:sgl)
            n320 = Index Array(array=w257, index=w256) -> (element=w232:sgl)
            n321 = Equal To 0?(x=w232) -> (x = 0?=w234:bool)
            n322 = Select(t=1.0, s=w234, f=w232) -> (s? t:f=w231:dbl)
            n323 = Power Of X(1:w231, 2:-0.826) -> (0:w243:dbl)
            n324 = Select(t=sgl 1.0, s=w264, f=sgl 0.0) -> (s? t:f=w255:sgl)
            n325 = Power Of X(1:w237, 2:-0.826) -> (0:w238:dbl)
            n326 = Select(t=sgl 1.0, s=w259, f=sgl 0.0) -> (s? t:f=w254:sgl)
            n327 = Multiply(x=93.909, y=w243) -> (x*y=w236:dbl)
            n328 = Multiply(x=w254, y=w236) -> (x*y=w252:dbl)
            n329 = Multiply(x=93.909, y=w238) -> (x*y=w235:dbl)
            n330 = Multiply(x=w255, y=w235) -> (x*y=w253:dbl)
            n331 = Add(x=w255, y=w254) -> (x+y=w249:sgl)
            n332 = Add(x=w253, y=w252) -> (x+y=w251:dbl)
            n333 = local read "Last Position"() -> (w267:cluster{"X":sgl, "Y":sgl})
            n334 = Greater Than 0?(x=w249) -> (x > 0?=w250:bool)
            n335 = case shown="False" w250 {
              selector: w250 -> [w268 w270]
              tunnel: w251 -> [_ w273]
              tunnel: w249 -> [_ w272]
              tunnel: [sgl 0.0 w271] -> w245
              tunnel: [w268 w270] -> w248
              tunnel: [w268 w270] -> w247
              frame False {
              }
              frame True {
                # "Avg Values"
                n336 = Divide(x=w273, y=w272) -> (x/y=w271:dbl)
              }
            }
            n337 = Unbundle(w267) -> ("Y"=w246:sgl)  [unwired: 1 out]
            n338 = Bundle(w245, "Y"=w246) -> (w244:cluster{dbl, "Y":sgl})  [unwired: 1 in]
          }
        }
        n339 = And(x=w138, y=w136) -> (x .and. y?=w156:bool)
        "Position Valid" <- w156
        n340 = Exclusive Or(1:w136, 2:w138) -> (0:w212:bool)
        n341 = case shown="True" w156 {
          tunnel: [w810 w813] -> w157
          tunnel: [w811 w812] -> w149
          tunnel: w223 -> [_ w813]
          tunnel: w140 -> [_ w812]
          tunnel: w212 -> [_ _]
          frame False {
            w810 = sgl 0.0 ("f")
            n342 = Bundle("f"=w810, "f"=w810) -> (w811:cluster{"f":sgl, "f":sgl})  [unwired: 1 in]
          }
          frame True {
            # "For Servos"
            "Last Orientation" <- w813
            "Last Position" <- w812
          }
        }
        "Robot Coordinates - Avgd" <- w149
        "Orientation Avgd" <- w157
        n343 = local read "History Size"() -> (w206:u8)
        n344 = Decrement(x=w206) -> (x-1=w207:u8)
        n345 = for {
          N: w206 -> [_]
          shift-right: [w851] -> w225
          shift-left: w222 -> [w850]
          tunnel: w149 -> [w849]
          tunnel: w207 -> [w848]
          i -> [w847]
          n346 = Subtract(x=w848, y=w847) -> (x-y=w846:i32)
          n347 = Equal To 0?(x=w846) -> (x = 0?=w845:bool)
          n348 = case shown="False" w845 {
            tunnel: w846 -> [w853 w858]
            tunnel: w850 -> [w856 w859]
            tunnel: [w854 w860] -> w851
            tunnel: w849 -> [_ w857]
            frame False {
              n349 = Decrement(x=w853) -> (x-1=w852:i32)
              n350 = Index Array(array=w856, index=w852) -> (element=w855:cluster{sgl, sgl})
              n351 = Replace Array Subset(array=w856, new element=w855, index=w853) -> (w854:cluster{sgl, sgl}[])
            }
            frame True {
              n352 = Replace Array Subset(array=w859, new element=w857, index=w858) -> (w860:cluster{sgl, sgl}[])
            }
          }
        }
        n353 = Unbundle(w149) -> ("upper limit"=w159:dbl, "upper limit"=w158:dbl)
        n354 = shared-variable "RT myRIO Target - Overlord\\Localization_Variables_r0.lvlib\\loc_x"(w159) -> ()  [unwired: 1 in, 1 out]
        n355 = shared-variable "RT myRIO Target - Overlord\\Localization_Variables_r0.lvlib\\loc_y"(w158) -> ()  [unwired: 1 in, 1 out]
        n356 = shared-variable "RT myRIO Target - Overlord\\Localization_Variables_r0.lvlib\\loc_theta"(w157) -> ()  [unwired: 1 in, 1 out]
        n357 = shared-variable "RT myRIO Target - Overlord\\Localization_Variables_r0.lvlib\\loc_flag"(w156) -> ()  [unwired: 1 in, 1 out]
        n358 = Decrement(x=w206) -> (x-1=w208:u8)
        n359 = for {
          N: w206 -> [_]
          shift-right: [w835] -> w226
          shift-left: w221 -> [w834]
          tunnel: w157 -> [w833]
          tunnel: w208 -> [w832]
          i -> [w831]
          n360 = Subtract(x=w832, y=w831) -> (x-y=w829:i32)
          n361 = Equal To 0?(x=w829) -> (x = 0?=w830:bool)
          n362 = case shown="False" w830 {
            tunnel: w829 -> [w837 w842]
            tunnel: w834 -> [w840 w843]
            tunnel: [w838 w844] -> w835
            tunnel: w833 -> [_ w841]
            frame False {
              # "Shift"
              n363 = Decrement(x=w837) -> (x-1=w836:i32)
              n364 = Index Array(array=w840, index=w836) -> (element=w839:sgl)
              n365 = Replace Array Subset(array=w840, new element=w839, index=w837) -> (w838:sgl[])
            }
            frame True {
              # "insert new"
              n366 = Replace Array Subset(array=w843, new element=w841, index=w842) -> (w844:sgl[])
            }
          }
        }
        n367 = Decrement(x=w206) -> (x-1=w205:u8)
        n368 = for {
          N: w206 -> [_]
          shift-right: [w820] -> w224
          shift-left: w220 -> [w819]
          tunnel: w156 -> [w818]
          tunnel: w205 -> [w817]
          i -> [w816]
          n369 = Subtract(x=w817, y=w816) -> (x-y=w814:i32)
          n370 = Equal To 0?(x=w814) -> (x = 0?=w815:bool)
          n371 = case shown="False" w815 {
            tunnel: w819 -> [w825 w827]
            tunnel: [w823 w828] -> w820
            tunnel: w818 -> [_ w826]
            tunnel: w814 -> [w821 _]
            frame False {
              n372 = Decrement(x=w821) -> (x-1=w822:i32)
              n373 = Index Array(array=w825, index=w822) -> (element=w824:bool)
              n374 = Replace Array Subset(array=w825, new element=w824, index=w821) -> (w823:bool[])
            }
            frame True {
              n375 = Replace Array Subset(array=w827, new element=w826) -> (w828:bool[])  [unwired: 1 in]
            }
          }
        }
        n376 = Boolean To (0,1)(Boolean=w224) -> (0, 1=w217:i16[])
        n377 = Add Array Elements(numeric array=w217) -> (sum=w216:i16)
        n378 = Greater Or Equal?(x=w216, y=i16 2) -> (x >= y?=w152:bool)
        "Position \nLock Status" <- w152
        n379 = shared-variable "RT myRIO Target - Overlord\\Localization_Variables_r0.lvlib\\Position_Lock"(w152) -> ()  [unwired: 1 in, 1 out]
        n380 = case shown="True" w156 {
          tunnel: w149 -> [_ w809]
          frame False {
          }
          frame True {
            # "update debug graph\nif current is valid"
            n381 = Unbundle(w809) -> ("upper limit"=w808:dbl, "upper limit"=w807:dbl)
            n382 = Build Array(w807) -> (w805:dbl[])
            n383 = Build Array(w808) -> (w806:dbl[])
            n384 = Bundle(w806, w805) -> (→"Real Position in Course 2":cluster{dbl[], dbl[]})  [unwired: 1 in]
          }
        }
        n385 = Unbundle By Name(w149) -> ("upper limit"=w146:dbl, "upper limit"=w148:dbl)
        n386 = Multiply(x=w146, y=w147) -> ()  [unwired: 1 out]
        n387 = Multiply(x=w148, y=w147) -> ()  [unwired: 1 out]
        n388 = Round Toward -Infinity(1:w146) -> (0:w145:dbl)
        n389 = Subtract(x=w146, y=w145) -> (x-y=w144:dbl)
        n390 = Multiply(x=w144, y=12.0) -> (x*y=→"inches":dbl)
      }
    }
    n391 = case shown="True" w113 {
      tunnel: w112 -> [_ w120]
      frame False {
      }
      frame True {
        n392 = call "Tick Count3"() -> ("Tick Count(uSec)"=w121:u32)
        n393 = Subtract(x=w121, y=w120) -> (x-y=w124:u32)
        n394 = Divide(x=w124, y=u32 1000 ("x")) -> (x/y=→"dT":dbl)
      }
    }
    n395 = call "Tick Count6"() -> ("Tick Count(uSec)"=w110:u32)
    "Robot Coordinates\nHistory" <- w109
    "Orientation\nHistory" <- w114
    "Position Valid\nHistory" <- w115
  }
  n396 = disable-structure shown="Enabled" {
    disable-tunnel: [w863 _] -> _
    disable-tunnel: ["Search Step Size\n(deg)" _] -> _
    frame Enabled {
      n397 = Multiply(x=3.413333333333333, y="Search Step Size\n(deg)") -> (x*y=w861:dbl)
      n398 = To Unsigned Word Integer(number=w861) -> (unsigned 16bit integer=w863:u16)
    }
    frame Disabled {
    }
  }
  n399 = Multiply(x="Move Servo\nThreshold (deg)", y=3.413333333333333) -> (x*y=w18:dbl)
  n400 = To Unsigned Word Integer(number=w18) -> ()  [unwired: 1 out]
  n401 = call "Tick Count8"() -> ()  [unwired: 1 out]
  n402 = flat-sequence {
    tunnel: [w867] -> w42
    tunnel: [w866] -> w41
    tunnel: [w871] -> w40
    tunnel: ["Left Servo\nID"] -> w29
    tunnel: ["Right Servo\nID"] -> w28
    tunnel: ["Compliance Slope"] -> w27
    tunnel: [w911] -> w39
    tunnel: [w910] -> w38
    tunnel: w42 -> [w909]
    tunnel: w41 -> [w908]
    tunnel: w40 -> [w907]
    tunnel: w29 -> [w905]
    tunnel: w28 -> [w904]
    tunnel: w27 -> [w903]
    tunnel: w39 -> [w1184]
    tunnel: w38 -> [w1183]
    frame #0 {
      # "BAUD RATE"
      # "Initialize UART and DIO"
      n403 = call-poly "VISA Configure Serial Port"("VISA resource name"=refnum<visa-resource-name> "ASRL1::INSTR", "Enable Termination\nChar (T)"=FALSE ("Enable Termination\nChar (T)"), "baud rate (9600)"=u32 115200) -> ("VISA resource name out"=w867:refnum<visa-resource-name>)  [unwired: 11 in, 1 out]
      n404 = call <vilib>:"Smart Open.vi"("Channel Names"=tag[] ["A/DIO2"]) -> ("DIO Ref Out"=w866:T9)  [unwired: 9 in, 1 out]
      n405 = flat-sequence {
        tunnel: w867 -> [w879]
        tunnel: w866 -> [w878]
        tunnel: "Left Servo\nID" -> [w880]
        tunnel: [w877] -> w868
        tunnel: "Compliance Slope" -> [w876]
        tunnel: "Right Servo\nID" -> [w893]
        tunnel: w868 -> [w892]
        tunnel: "Compliance Slope" -> [w891]
        tunnel: w867 -> [w890]
        tunnel: w866 -> [w889]
        frame #0 {
          w877 = 3
          n406 = while {
            tunnel: w877 -> [w886]
            tunnel: w879 -> [w884]
            tunnel: w878 -> [w883]
            tunnel: w880 -> [w882]
            tunnel: w876 -> [w881]
            i -> [w887]
            stop <- w885 stop-if-true
            n407 = call "Set_Compliance_Slope_R2.vi"("Compliance Slope"=w881, "DIO Ref Out"=w883, "VISA resource name"=w884, "Servo ID"=w882) -> ()  [unwired: 6 in, 2 out]
            n408 = Increment(x=w887) -> (x+1=w888:i32)
            n409 = Greater Or Equal?(x=w888, y=w886) -> (x >= y?=w885:bool)
          }
        }
        frame #1 {
          n410 = while {
            tunnel: w892 -> [w899]
            tunnel: w893 -> [w897]
            tunnel: w890 -> [w896]
            tunnel: w889 -> [w895]
            tunnel: w891 -> [w894]
            i -> [w900]
            stop <- w898 stop-if-true
            n411 = call "Set_Compliance_Slope_R2.vi"("Compliance Slope"=w894, "DIO Ref Out"=w895, "VISA resource name"=w896, "Servo ID"=w897) -> ()  [unwired: 6 in, 2 out]
            n412 = Increment(x=w900) -> (x+1=w901:i32)
            n413 = Greater Or Equal?(x=w901, y=w899) -> (x >= y?=w898:bool)
          }
        }
      }
      n414 = call "Tick Count"() -> ("Tick Count(uSec)"=w871:u32)
    }
    frame #1 {
      # "Service Count"
      n415 = while {
        shift-right: [w914] -> _
        shift-left: w907 -> [w931]
        tunnel: "Max Write\nTx Attempts" -> [w926]
        tunnel: "Max Read\nTx Attempts" -> [w925]
        shift-right: [w921] -> w911
        shift-left: w909 -> [w924]
        shift-right: [w920] -> w910
        shift-left: w908 -> [w923]
        tunnel: w905 -> [w919]
        tunnel: w904 -> [w918]
        tunnel: w903 -> [w917]
        shift-right: [w915] -> _
        shift-left: u16 0 -> [w916]
        stop <- "close comms" stop-if-true
        # "Loop Timer"
        n416 = local read "SERVO ENABLE"() -> (w913:bool)
        n417 = call "Tick Count2"() -> ("Tick Count(uSec)"=w914:u32)
        n418 = Subtract(x=w914, y=w931) -> (x-y=w930:u32)
        n419 = call "Wait4"("Count(mSec)"="Servo Comm\nLoop Time (ms)") -> ()  [unwired: 1 out]
        n420 = Divide(x=w930, y=u32 1000) -> (x/y=→"dT - Comm Loop":dbl)
        n421 = case shown="True" w913 {
          tunnel: w926 -> [_ w940]
          tunnel: w925 -> [_ w971]
          tunnel: w924 -> [w934 w935]
          tunnel: w923 -> [w933 w964]
          tunnel: [w934 w937] -> w921
          tunnel: [w933 w936] -> w920
          tunnel: w919 -> [_ w943]
          tunnel: w918 -> [_ w942]
          tunnel: w917 -> [_ w941]
          tunnel: w916 -> [_ w939]
          tunnel: [u16 100 w938] -> w915
          frame False {
            # "Restart at same value\nUsed to Periodically update \nCompliance Slope"
          }
          frame True {
            n422 = flat-sequence {
              tunnel: [w977] -> w975
              tunnel: [w978] -> w974
              tunnel: [w976] -> w973
              tunnel: w971 -> [w979]
              tunnel: [w981] -> w962
              tunnel: [w980] -> w960
              tunnel: w935 -> [w981]
              tunnel: w964 -> [w980]
              tunnel: w943 -> [w976]
              tunnel: w975 -> [w999]
              tunnel: w974 -> [w1000]
              tunnel: w973 -> [w998]
              tunnel: [w998] -> w972
              tunnel: [w997] -> w965
              tunnel: [w996] -> w963
              tunnel: w962 -> [w996]
              tunnel: [w995] -> w961
              tunnel: w960 -> [w995]
              tunnel: w972 -> [w1021]
              tunnel: w940 -> [w1020]
              tunnel: w965 -> [w1015]
              tunnel: w963 -> [w1017]
              tunnel: w961 -> [w1016]
              tunnel: [w1017] -> w958
              tunnel: [w1016] -> w956
              tunnel: [w1054] -> w959
              tunnel: w958 -> [w1054]
              tunnel: [w1053] -> w957
              tunnel: w956 -> [w1053]
              tunnel: ["Servo Comm\nWait Time - (ms)"] -> w948
              tunnel: w971 -> [w1061]
              tunnel: [w1060] -> w970
              tunnel: [w1059] -> w969
              tunnel: [w1055] -> w967
              tunnel: w959 -> [w1058]
              tunnel: w957 -> [w1057]
              tunnel: [w1058] -> w955
              tunnel: [w1057] -> w952
              tunnel: [w1056] -> w949
              tunnel: w948 -> [w1056]
              tunnel: w942 -> [w1055]
              tunnel: w970 -> [w1081]
              tunnel: w969 -> [w1080]
              tunnel: [w1079] -> w968
              tunnel: w967 -> [w1079]
              tunnel: [w1078] -> w966
              tunnel: w955 -> [w1077]
              tunnel: [w1077] -> w954
              tunnel: [w1076] -> w953
              tunnel: w952 -> [w1076]
              tunnel: w949 -> [w1075]
              tunnel: [w1075] -> w947
              tunnel: w968 -> [w1103]
              tunnel: w966 -> [w1101]
              tunnel: w940 -> [w1102]
              tunnel: w954 -> [w1100]
              tunnel: w953 -> [w1099]
              tunnel: [w1100] -> w951
              tunnel: [w1099] -> w950
              tunnel: w947 -> [w1096]
              tunnel: [w1096] -> w946
              tunnel: w951 -> [w1136]
              tunnel: w950 -> [w1135]
              tunnel: w946 -> [w1134]
              tunnel: [w1136] -> w945
              tunnel: [w1135] -> w944
              tunnel: w945 -> [w1140]
              tunnel: w944 -> [w1139]
              tunnel: w943 -> [w1145]
              tunnel: w942 -> [w1144]
              tunnel: w941 -> [w1143]
              tunnel: w939 -> [w1138]
              tunnel: w940 -> [w1142]
              tunnel: [w1141] -> w938
              tunnel: [w1140] -> w937
              tunnel: [w1139] -> w936
              frame #0 {
                n423 = while {
                  tunnel: [w994] -> w977
                  tunnel: w976 -> [w993]
                  tunnel: [w986] -> w978
                  tunnel: w979 -> [w984]
                  tunnel: w981 -> [w983]
                  tunnel: w980 -> [w982]
                  i -> [w985]
                  stop <- w987 stop-if-true
                  # "Attemp to Read Until\nMax Read Tx Attemps Limit"
                  n424 = call "ReadServo_R3.vi"("DIO Ref In"=w982, "VISA resource name out"=w983, "Servo ID"=w993) -> ("Error"=w990:u8, "Valid Checksum"=w991:bool, "Current Position"=w994:u64)  [unwired: 6 in]
                  n425 = Increment(x=w985) -> (x+1=w988:i32)
                  n426 = Equal To 0?(x=w990) -> (x = 0?=w992:bool)
                  n427 = Greater Or Equal?(x=w988, y=w984) -> (x >= y?=w989:bool)
                  n428 = And(x=w991, y=w992) -> (x .and. y?=w986:bool)
                  n429 = Or(x=w986, y=w989) -> (x .or. y?=w987:bool)
                }
              }
              frame #1 {
                # "Read Position First"
                n430 = local read "Servo Goal Position\n - Left"() -> (w997:u16)
                n431 = case shown="True" w1000 {
                  tunnel: w999 -> [_ w1005]
                  tunnel: w997 -> [_ w1003]
                  frame False {
                  }
                  frame True {
                    # "Convert Received Position to Angle Relative to Robot"
                    # "45 DEG MOUNT OFFSET"
                    # "1024/300"
                    n432 = local write "Current L (10bit)"(w1005) -> ()
                    n433 = To Word Integer(number=w1005) -> (16bit integer=w1009:i16)
                    n434 = To Word Integer(number=w1003) -> (16bit integer=w1008:i16)
                    n435 = Subtract(x=w1008, y=w1009) -> (x-y=w1007:i16)
                    n436 = Divide(x=w1005, y=3.413333333333333) -> (x/y=w1013:dbl)
                    n437 = Absolute Value(x=w1007) -> (abs(x)=w1006:i16)
                    n438 = Subtract(x=w1013, y=sgl 60.0) -> (x-y=w1011:dbl)
                    n439 = Greater?(x=w1006, y=u16 5) -> (0:w1002:bool)
                    n440 = Add(x=w1011, y=sgl 45.0) -> (x+y=w1001:dbl)
                    n441 = local write "Servo Moving - L"(w1002) -> ()
                    n442 = local write "Move Servo - L"(w1002) -> ()
                    n443 = local write "Current Angle\n - Left (internal)"(w1001) -> ()
                    n444 = shared-variable "RT myRIO Target - Overlord\\Localization_Variables_r0.lvlib\\Left Servo Angle_Current"(w1001) -> ()  [unwired: 1 in, 1 out]
                  }
                }
              }
              frame #2 {
                n445 = local read "Move Servo - L"() -> (w1018:bool)
                n446 = case shown="True" w1018 {
                  tunnel: w1021 -> [_ w1036]
                  tunnel: w1015 -> [_ w1023]
                  tunnel: [TRUE w1034] -> w1019
                  tunnel: w1020 -> [_ w1026]
                  tunnel: w1017 -> [_ w1025]
                  tunnel: w1016 -> [_ w1024]
                  frame False {
                    # "Only Send if Current Position is far enough"
                  }
                  frame True {
                    w1032 = 1
                    # "High Byte"
                    # "Low Byte"
                    n447 = Type Cast(type="", x=w1023) -> (*(type *) &x=w1033:string)
                    n448 = local write "Servo Moving - L"(TRUE) -> ()
                    n449 = String Subset(string=w1033, offset (0)=1, length (rest)=w1032) -> (substring=w1028:string)
                    n450 = String Subset(string=w1033, offset (0)=0, length (rest)=w1032) -> (substring=w1027:string)
                    n451 = while {
                      tunnel: w1036 -> [w1050]
                      tunnel: [w1042] -> w1034
                      tunnel: w1028 -> [w1046]
                      tunnel: w1027 -> [w1045]
                      tunnel: w1026 -> [w1039]
                      tunnel: w1025 -> [w1038]
                      tunnel: w1024 -> [w1037]
                      i -> [w1040]
                      stop <- w1041 stop-if-true
                      # "Attemp to Write Until\nMax Write Tx Attemps Limit"
                      n452 = call "MoveServo_R3.vi"("DIO Ref Out"=w1037, "VISA resource name out"=w1038, "GP - Low Byte"=w1046, "GP - High Byte"=w1045, "Servo ID"=w1050) -> ("Valid Checksum"=w1047:bool, "Error"=w1049:u64)  [unwired: 5 in]
                      n453 = Equal To 0?(x=w1049) -> (x = 0?=w1048:bool)
                      n454 = And(x=w1047, y=w1048) -> (x .and. y?=w1042:bool)
                      n455 = Increment(x=w1040) -> (x+1=w1044:i32)
                      n456 = Greater Or Equal?(x=w1044, y=w1039) -> (x >= y?=w1043:bool)
                      n457 = Or(x=w1042, y=w1043) -> (x .or. y?=w1041:bool)
                    }
                  }
                }
                n458 = case shown="True" w1019 {
                  frame False {
                  }
                  frame True {
                    # "Update Servo flag"
                    n459 = local write "Move Servo - L"(FALSE) -> ()
                  }
                }
              }
              frame #3 {
                n460 = call "Wait2"("Count(mSec)"="Servo Comm\nWait Time - (ms)") -> ()  [unwired: 1 out]
              }
              frame #4 {
                n461 = while {
                  tunnel: [w1074] -> w1060
                  tunnel: w1055 -> [w1073]
                  tunnel: [w1066] -> w1059
                  tunnel: w1061 -> [w1064]
                  tunnel: w1058 -> [w1063]
                  tunnel: w1057 -> [w1062]
                  i -> [w1065]
                  stop <- w1067 stop-if-true
                  # "Attemp to Read Until\nMax Read Tx Attemps Limit"
                  n462 = call "ReadServo_R3.vi"("DIO Ref In"=w1062, "VISA resource name out"=w1063, "Servo ID"=w1073) -> ("Error"=w1070:u8, "Valid Checksum"=w1071:bool, "Current Position"=w1074:u64)  [unwired: 6 in]
                  n463 = Increment(x=w1065) -> (x+1=w1068:i32)
                  n464 = Equal To 0?(x=w1070) -> (x = 0?=w1072:bool)
                  n465 = Greater Or Equal?(x=w1068, y=w1064) -> (x >= y?=w1069:bool)
                  n466 = And(x=w1071, y=w1072) -> (x .and. y?=w1066:bool)
                  n467 = Or(x=w1066, y=w1069) -> (x .or. y?=w1067:bool)
                }
              }
              frame #5 {
                n468 = local read "Servo Goal Position\n - Right"() -> (w1078:u16)
                n469 = case shown="True" w1080 {
                  tunnel: w1081 -> [_ w1085]
                  tunnel: w1078 -> [_ w1084]
                  frame False {
                    # "Don't update current position"
                  }
                  frame True {
                    # "Convert Received Position to Angle Relative to Robot"
                    # "45 DEG MOUNT OFFSET"
                    # "1024/300"
                    n470 = local write "Current R (10bit)"(w1085) -> ()
                    n471 = Divide(x=w1085, y=3.413333333333333) -> (x/y=w1094:dbl)
                    n472 = Subtract(x=w1094, y=sgl 60.0) -> (x-y=w1092:dbl)
                    n473 = Subtract(x=w1092, y=sgl 45.0) -> (x-y=w1082:dbl)
                    n474 = To Word Integer(number=w1084) -> (16bit integer=w1089:i16)
                    n475 = local write "Current Angle\n - Right (internal)"(w1082) -> ()
                    n476 = To Word Integer(number=w1085) -> (16bit integer=w1090:i16)
                    n477 = shared-variable "RT myRIO Target - Overlord\\Localization_Variables_r0.lvlib\\Right Servo Angle_Current"(w1082) -> ()  [unwired: 1 in, 1 out]
                    n478 = Subtract(x=w1089, y=w1090) -> (x-y=w1088:i16)
                    n479 = Absolute Value(x=w1088) -> (abs(x)=w1087:i16)
                    n480 = Greater?(x=w1087, y=u16 5) -> (0:w1083:bool)
                    n481 = local write "Servo Moving - R"(w1083) -> ()
                    n482 = local write "Move Servo - R"(w1083) -> ()
                  }
                }
              }
              frame #6 {
                n483 = local read "Move Servo - R"() -> (w1097:bool)
                n484 = case shown="True" w1097 {
                  tunnel: w1101 -> [_ w1106]
                  tunnel: w1103 -> [_ w1113]
                  tunnel: [TRUE w1114] -> w1098
                  tunnel: w1102 -> [_ w1109]
                  tunnel: w1100 -> [_ w1108]
                  tunnel: w1099 -> [_ w1107]
                  frame False {
                  }
                  frame True {
                    w1116 = 1
                    # "High Byte"
                    # "Low Byte"
                    n485 = Type Cast(type="", x=w1106) -> (*(type *) &x=w1115:string)
                    n486 = local write "Servo Moving - R"(TRUE) -> ()
                    n487 = String Subset(string=w1115, offset (0)=1, length (rest)=w1116) -> (substring=w1112:string)
                    n488 = String Subset(string=w1115, offset (0)=0, length (rest)=w1116) -> (substring=w1111:string)
                    n489 = while {
                      tunnel: [w1125] -> w1114
                      tunnel: w1113 -> [w1130]
                      tunnel: w1112 -> [w1129]
                      tunnel: w1111 -> [w1128]
                      tunnel: w1109 -> [w1123]
                      tunnel: w1108 -> [w1121]
                      tunnel: w1107 -> [w1120]
                      i -> [w1124]
                      stop <- w1122 stop-if-true
                      # "Attemp to Write Until\nMax Write Tx Attemps Limit"
                      n490 = call "MoveServo_R3.vi"("DIO Ref Out"=w1120, "VISA resource name out"=w1121, "GP - Low Byte"=w1129, "GP - High Byte"=w1128, "Servo ID"=w1130) -> ("Valid Checksum"=w1132:bool, "Error"=w1131:u64)  [unwired: 5 in]
                      n491 = Increment(x=w1124) -> (x+1=w1126:i32)
                      n492 = Greater Or Equal?(x=w1126, y=w1123) -> (x >= y?=w1127:bool)
                      n493 = Equal To 0?(x=w1131) -> (x = 0?=w1133:bool)
                      n494 = And(x=w1132, y=w1133) -> (x .and. y?=w1125:bool)
                      n495 = Or(x=w1125, y=w1127) -> (x .or. y?=w1122:bool)
                    }
                  }
                }
                n496 = case shown="True" w1098 {
                  frame False {
                  }
                  frame True {
                    # "Update Servo flag"
                    n497 = local write "Move Servo - R"(FALSE) -> ()
                  }
                }
              }
              frame #7 {
                n498 = call "Wait3"("Count(mSec)"=w1134) -> ()  [unwired: 1 out]
              }
              frame #8 {
                # "Increment Service Count"
                # "Update Compliance Slope\nEvery x loops"
                n499 = Equal?(x=w1138, y=u16 1000) -> (x = y?=w1147:bool)
                n500 = case shown="True" w1147 {
                  tunnel: w1143 -> [_ w1157]
                  tunnel: w1140 -> [_ w1156]
                  tunnel: w1139 -> [_ w1155]
                  tunnel: w1140 -> [_ w1154]
                  tunnel: w1139 -> [_ w1153]
                  tunnel: w1145 -> [_ w1152]
                  tunnel: w1144 -> [_ w1151]
                  tunnel: w1138 -> [w1148 _]
                  tunnel: [w1148 u16 0] -> w1146
                  tunnel: w1142 -> [_ w1149]
                  frame False {
                  }
                  frame True {
                    # "Reset Service\nCount"
                    n501 = flat-sequence {
                      tunnel: w1156 -> [w1162]
                      tunnel: w1155 -> [w1161]
                      tunnel: w1152 -> [w1163]
                      tunnel: [w1159] -> w1158
                      tunnel: w1157 -> [w1160]
                      tunnel: w1149 -> [w1159]
                      tunnel: w1151 -> [w1175]
                      tunnel: w1158 -> [w1174]
                      tunnel: w1157 -> [w1173]
                      tunnel: w1154 -> [w1172]
                      tunnel: w1153 -> [w1171]
                      frame #0 {
                        n502 = while {
                          tunnel: w1159 -> [w1170]
                          tunnel: w1162 -> [w1168]
                          tunnel: w1161 -> [w1167]
                          tunnel: w1163 -> [w1166]
                          tunnel: w1160 -> [w1165]
                          i -> [w1164]
                          stop <- w1169 stop-if-true
                          n503 = call "Set_Compliance_Slope_R2.vi"("Compliance Slope"=w1165, "DIO Ref Out"=w1167, "VISA resource name"=w1168, "Servo ID"=w1166) -> ()  [unwired: 6 in, 2 out]
                          n504 = Greater Or Equal?(x=w1164, y=w1170) -> (x >= y?=w1169:bool)
                        }
                      }
                      frame #1 {
                        n505 = while {
                          tunnel: w1174 -> [w1182]
                          tunnel: w1175 -> [w1180]
                          tunnel: w1172 -> [w1179]
                          tunnel: w1171 -> [w1178]
                          tunnel: w1173 -> [w1177]
                          i -> [w1176]
                          stop <- w1181 stop-if-true
                          n506 = call "Set_Compliance_Slope_R2.vi"("Compliance Slope"=w1177, "DIO Ref Out"=w1178, "VISA resource name"=w1179, "Servo ID"=w1180) -> ()  [unwired: 6 in, 2 out]
                          n507 = Greater Or Equal?(x=w1176, y=w1182) -> (x >= y?=w1181:bool)
                        }
                      }
                    }
                  }
                }
                n508 = Increment(x=w1146) -> (x+1=w1141:u16)
              }
            }
          }
        }
      }
    }
    frame #2 {
      n509 = VISA Close(VISA resource name=w1184) -> ()  [unwired: 1 in, 1 out]
      n510 = call <vilib>:"Close.vi"("DIO Ref In"=w1183) -> ()  [unwired: 10 in, 1 out]
    }
  }
  n511 = while {
    stop <- FALSE stop-if-true
    n512 = call "Wait9"("Count(mSec)"=u32 1000) -> ()  [unwired: 1 out]
  }
  n513 = while {
    shift-right: [w1255] -> _
    shift-left: "Initial Main State - Left" -> [w1277]
    shift-right: [w1247] -> _
    shift-left: "Search Direction - in - L" -> [w1271]
    shift-right: [w1246] -> _
    shift-left: FALSE -> [w1270]
    shift-right: [w1249] -> _
    shift-left: w13 -> [w1248]
    shift-right: [w1250] -> _
    shift-left: w13 -> [w1264]
    shift-right: [w1251] -> _
    shift-left: w13 -> [w1269]
    shift-right: [w1252] -> _
    shift-left: w13 -> [w1263]
    shift-right: [w1253] -> _
    shift-left: w13 -> [w1262]
    shift-right: [w1199] -> _
    shift-left: "Search Direction - in - Right" -> [w1212]
    shift-right: [w1243] -> _
    shift-left: FALSE -> [w1210]
    shift-right: [w1244] -> _
    shift-left: w12 -> [w1201]
    shift-right: [w1198] -> _
    shift-left: w12 -> [w1200]
    shift-right: [w1197] -> _
    shift-left: w12 -> [w1207]
    shift-right: [w1196] -> _
    shift-left: w12 -> [w1209]
    shift-right: [w1195] -> _
    shift-left: w12 -> [w1208]
    shift-right: [w1187] -> _
    shift-left: "Initial Main State- Right" -> [w1224]
    shift-right: [w1239] -> _
    shift-left: 0 -> [w1241]
    shift-right: [w1191] -> _
    shift-left: 0 -> [w1216]
    shift-right: [w1238] -> _
    shift-left: "Initial Tracking State - Left" -> [w1240]
    shift-right: [w1193] -> _
    shift-left: "Initial Tracking State - Right" -> [w1222]
    shift-right: [w1192] -> _
    shift-left: "Initial Recovery State  - Right" -> [w1223]
    shift-right: [w1236] -> _
    shift-left: "Initial Recovery State - L" -> [w1237]
    stop <- FALSE stop-if-true
    w1231 = enum16{"Track", "Reactive Predict", ""}."Track" ("Initial Tracking State - Right")
    w1257 = T5."Tracking" ("Next Main State")
    # "Wait for New"
    # "ADD TRACKING TIMEOUT COUNT**********************"
    # "Service Track Angle Flag"
    # "Add Logic to Have Search Directions\nopposite if Both Searching"
    # "REMOVE LAST GOAL POSITION WITH cURRENT"
    # "Go to Current State"
    # "Add Logic to Have Search Directions\nopposite if Both Searching"
    # "Manuallly Reset\nRespond Var"
    # "Manuallly Reset\nRespond Var"
    # "Update Comm Process Variables"
    # "Both  inTracking (main state)"
    # "Current delta - L"
    # "delta move sum - R"
    # "delta move sum - L"
    # "Current delta - R"
    # "Service Move Respond Variables"
    n514 = local read "Min Num Frames\nper Search"() -> (w1245:i32)
    n515 = local read "Minimum Delta \nServo Threshold"() -> (w1261:i16)
    n516 = local read "Maximum Move \nServo Threshold"() -> (w1260:i16)
    n517 = local read "Middle Beacon\nCoordinates"() -> (w1202:cluster{"X":sgl, "Y":sgl})
    n518 = local read "Position \nLock Status"() -> (w1268:bool)
    n519 = local read "Position \nLock Status"() -> (w1205:bool)
    n520 = local read "Search Step Size"() -> (w1259:u16)
    n521 = local read "Last Orientation"() -> (w1266:sgl)
    n522 = local read "Last Orientation"() -> (w1203:sgl)
    n523 = local read "Last Position"() -> (w1267:cluster{"X":sgl, "Y":sgl})
    n524 = local read "Last Position"() -> (w1204:cluster{"X":sgl, "Y":sgl})
    n525 = local read "Min Num Frames\nper Search"() -> (w1206:i32)
    n526 = call "Wait"("Count(mSec)"="Servo Algorithm\nCycle Time(ms)") -> ()  [unwired: 1 out]
    n527 = local read "Minimum Delta \nServo Threshold"() -> (w1214:i16)
    n528 = local read "Maximum Move \nServo Threshold"() -> (w1213:i16)
    n529 = local read "Search Step Size"() -> (w1211:u16)
    n530 = local read "New Data  Flag\nRight Servo"() -> (w1219:bool)
    n531 = local read "New Data  Flag\nLeft Servo"() -> (w1235:bool)
    n532 = local read "Image Lock - Right"() -> (w1221:bool)
    n533 = local read "Tracking Angle - Right"() -> (w1218:sgl)
    n534 = local read "Image Lock - Left"() -> (w1276:bool)
    n535 = local read "Tracking Angle - Left"() -> (w1274:sgl)
    n536 = local read "Current R (10bit)"() -> (w1217:u16)
    n537 = local read "Current L (10bit)"() -> (w1273:u16)
    n538 = case shown="True" w1235 {
      tunnel: [w1806 w1844] -> w1279
      tunnel: [w1800 w1843] -> w1278
      tunnel: w1277 -> [w1801 w1842]
      tunnel: w1276 -> [_ w1841]
      tunnel: "Track Angle Valid - Left" -> [_ w1840]
      tunnel: w1274 -> [_ w1839]
      tunnel: w1273 -> [w1806 w1838]
      tunnel: "Mounting Offset - Left" -> [_ w1837]
      tunnel: w1271 -> [w1797 w1836]
      tunnel: w1270 -> [_ w1835]
      tunnel: w1269 -> [w1798 w1834]
      tunnel: w1268 -> [_ w1833]
      tunnel: w1267 -> [_ w1832]
      tunnel: w1266 -> [_ w1831]
      tunnel: "Middle Beacon\nCoordinates" -> [_ w1830]
      tunnel: w1264 -> [w1796 w1829]
      tunnel: w1263 -> [w1795 w1828]
      tunnel: w1262 -> [w1799 w1827]
      tunnel: w1261 -> [_ w1826]
      tunnel: w1260 -> [_ w1825]
      tunnel: w1259 -> [_ w1824]
      tunnel: [0 w1823] -> w1256
      tunnel: [w1801 w1822] -> w1255
      tunnel: [w1800 w1821] -> w1254
      tunnel: [w1799 w1820] -> w1253
      tunnel: [w1795 w1819] -> w1252
      tunnel: [w1798 w1818] -> w1251
      tunnel: [w1796 w1817] -> w1250
      tunnel: w1248 -> [_ w1816]
      tunnel: [w1797 w1815] -> w1247
      tunnel: w1245 -> [_ w1814]
      tunnel: w1241 -> [w1804 w1813]
      tunnel: w1240 -> [w1803 w1812]
      tunnel: [w1804 w1811] -> w1239
      tunnel: [w1803 w1810] -> w1238
      tunnel: w1237 -> [w1802 w1809]
      tunnel: [w1802 w1808] -> w1236
      frame False {
        w1800 = FALSE
        # "Recovery Mode COunt"
        # "Frames Processed - L"
        # "Recovery Search move Count - L"
        # "Recovery Search Attempt Count- L"
        # "WAITING FOR NEW IMAGE, RETAIN ALL VALUES"
      }
      frame True {
        w1846 = u16 1023
        w1849 = u16 0
        # "New Tracking State"
        # "Tracking Timeout Count"
        # "Next Main State"
        # "Next Recovery State"
        # "Reset Respond"
        # "Search Direction"
        # "Recovery Count"
        # "Recovery Search move Count"
        # "Recovery Search Attempt Count"
        # "Frames Processed"
        # "Apply Floor/Ceiling to Goal Position"
        # "Current move Delta"
        # "Service Track Angle Flag"
        # "Move Servo"
        # "Goal Position"
        # "Go to Current State"
        n539 = case shown="\"Start Up Search\", Default" w1842 {
          tunnel: w1838 -> [w1859 w1925 w2104]
          tunnel: w1839 -> [_ w1927 _]
          tunnel: w1824 -> [_ _ w2099]
          tunnel: w1836 -> [w1853 w1908 w2093]
          tunnel: [w1857 w1923 w2103] -> w1850
          tunnel: [w1867 w1924 w2102] -> w1843
          tunnel: w1840 -> [_ w1918 w2080]
          tunnel: [w1866 w1920 w2089] -> w1822
          tunnel: w1841 -> [w1860 w1919 w2078]
          tunnel: w1837 -> [_ w1928 w2100]
          tunnel: w1826 -> [_ w1926 _]
          tunnel: [w1863 w1922 w2084] -> w1823
          tunnel: w1825 -> [_ w1921 _]
          tunnel: w1834 -> [w1851 _ w2094]
          tunnel: [enum16{"Generic Sweep", "Recovery Search"}."Recovery Search" enum16{"Generic Sweep", "Recovery Search"}."Recovery Search" w2101] -> w1808
          tunnel: w1829 -> [_ _ w2098]
          tunnel: w1809 -> [_ _ w2081]
          tunnel: w1835 -> [_ w1905 w2110]
          tunnel: w1816 -> [_ w1901 w2105]
          tunnel: w1831 -> [_ w1911 w2107]
          tunnel: w1832 -> [_ w1912 w2108]
          tunnel: w1833 -> [_ w1913 w2109]
          tunnel: w1830 -> [_ w1910 w2106]
          tunnel: [FALSE w1907 w2082] -> w1821
          tunnel: w1814 -> [w1865 _ w2092]
          tunnel: [w1863 w1902 w2091] -> w1817
          tunnel: [w1863 w1902 w2097] -> w1820
          tunnel: [w1863 w1902 w2096] -> w1819
          tunnel: [w1855 w1903 w2095] -> w1818
          tunnel: w1828 -> [_ _ w2087]
          tunnel: w1827 -> [_ _ w2086]
          tunnel: [w1854 w1908 w2085] -> w1815
          tunnel: w1813 -> [_ w1917 _]
          tunnel: [w1863 w1909 w2084] -> w1811
          tunnel: w1812 -> [_ w1914 _]
          tunnel: [enum16{"Track", "Reactive Predict", ""}."Track" ("Initial Tracking State - Right") w1906 enum16{"Track", "Reactive Predict", ""}."Track" ("Initial Tracking State - Right")] -> w1810
          frame "Start Up Search", Default {
            w1863 = u16 0
            # "Image Lock"
            # "Search Direction"
            # "Wait for 'x' Images to be Processed\nBefore Going to Next Step"
            # "Next Main State"
            # "New Goal Position"
            # "Move Servo"
            # "Choose Next State"
            # "Frames Processed Count"
            n540 = Greater Or Equal?(x=w1851, y=w1865) -> (x >= y?=w1852:bool)
            n541 = case shown="True" w1852 {
              tunnel: w1859 -> [w1870 _]
              tunnel: w1853 -> [w1869 _]
              tunnel: [w1870 w1874] -> w1857
              tunnel: [w1868 0] -> w1855
              tunnel: [FALSE TRUE] -> w1856
              tunnel: w1851 -> [w1871 _]
              tunnel: [w1869 FALSE] -> w1854
              tunnel: "Start up Template State\n- LEFT" -> [_ w1878]
              frame False {
                # "Wait until Min Number of Frames (per search/step) Processed"
                # "Increase Frames\nProcessed Count"
                n542 = Increment(x=w1871) -> (x+1=w1868:i32)
              }
              frame True {
                # "left OR right"
                # "Startup FOUND"
                # "Current Cam State\n(write Shared var)"
                # "Current Cam State\n(read Shared var)"
                # "Write to Current State for Cam (shared var)"
                # "if Right or Left FOUND\n    enter 90deg case"
                # "Reset Frames\nProcessed Count"
                # "Startup - Cycle thru specific start up cases (certain angle per case) & wait 'x' # of images, determine if current case is indeed the actual case"
                # "Nearest step"
                n543 = case shown="False" "Boolean" {
                  tunnel: w1878 -> [w1883 _]
                  tunnel: [w1882 9] -> w1875
                  frame False {
                    # "Next Case (LEFT)\n\n**pre-set, see\nexcel sheet from Bill"
                    n544 = case shown="1" w1883 {
                      selector: w1883 -> [_ _ _ _ _ _ _ _ w1892]
                      tunnel: [3 3 4 6 6 7 1 1 w1892] -> w1882
                      frame 1 {
                      }
                      frame 2 {
                      }
                      frame 3 {
                      }
                      frame 4 {
                      }
                      frame 5 {
                      }
                      frame 6 {
                      }
                      frame 7 {
                      }
                      frame 8 {
                      }
                      frame 9, Default {
                        # "stay in 9"
                      }
                    }
                  }
                  frame True {
                    # "Change mode for image\nprocessing to case 9\n\nsearch for all 5 beacons individually"
                    # "Update Startup Case for Nav\nSet Startup Flag"
                  }
                }
                n545 = Decrement(x=w1875) -> (x-1=w1877:i32)
                n546 = Index Array(array="Startup GP per Case - LEFT 2", index=w1877) -> (element=w1874:u16)
                n547 = local write "Start up Template State\n- LEFT"(w1875) -> ()
              }
            }
            n548 = case shown="False" w1860 {
              tunnel: [w1895 FALSE] -> w1867
              tunnel: w1856 -> [w1895 _]
              tunnel: [w1896 T5."Tracking" ("Next Main State")] -> w1866
              frame False {
                # "Check other Servo\nStay in Startup  State"
                n549 = local read "Image Lock - Right"() -> (w1894:bool)
                n550 = case shown="False" w1894 {
                  tunnel: [T5."Start Up Search" ("Next Main State") T5."Recovery Mode" ("Next Main State")] -> w1896
                  frame False {
                  }
                  frame True {
                  }
                }
              }
              frame True {
                # "Override Move Servo\nCommand bc an Angle Was Found\nduring this Step"
                # "Transition to Tracking State When\nImage Processing has Locked"
              }
            }
          }
          frame "Tracking" {
            w1902 = 0
            # "Frames Processed Count"
            # "Image Lock - L"
            # "Track Angle Valid"
            # "Tracking Angle"
            # "Tracking Timeout Count"
            # "Max ove delta"
            # "Move delta threshold"
            # "mount offset"
            # "Current Position"
            # "Move Respond"
            # "Trackin Timeout count"
            # "Move Servo"
            # "delta"
            # "GP"
            # "Reset Move Respond"
            # "New Tracking State"
            # "Delta Move Sum"
            # "Choose Next State"
            n551 = case shown="\"Reactive Predict\"" w1914 {
              tunnel: w1928 -> [w1946 _]
              tunnel: w1927 -> [w1945 _]
              tunnel: w1926 -> [w1944 _]
              tunnel: w1925 -> [w1943 w2002]
              tunnel: [w1942 w2000] -> w1924
              tunnel: [w1941 w2008] -> w1923
              tunnel: [w1940 0] -> w1922
              tunnel: w1921 -> [w1939 _]
              tunnel: w1919 -> [w1938 w1992]
              tunnel: w1918 -> [w1937 w1995]
              tunnel: w1917 -> [w1936 w1997]
              tunnel: w1913 -> [_ w2007]
              tunnel: w1912 -> [_ w2006]
              tunnel: w1911 -> [_ w2005]
              tunnel: w1910 -> [_ w2004]
              tunnel: w1905 -> [_ w2003]
              tunnel: w1901 -> [_ w2001]
              tunnel: [TRUE w1998] -> w1907
              tunnel: [w1933 w1996] -> w1909
              tunnel: [w1931 w1994] -> w1906
              tunnel: [0 0] -> w1903
              frame "Track", Default {
                # "Reset"
                # "Tracking Timeout"
                # "Move Delta"
                # "Goal Position"
                # "Tracking Move"
                # "Move Servo"
                # "Only Consider Tracking Angle\n\nIF\n\nImage Locked        == T\nTrack Angle Flag   == T"
                n552 = And(x=w1938, y=w1937) -> (x .and. y?=w1930:bool)
                n553 = case shown="False" w1930 {
                  tunnel: w1946 -> [_ w1954]
                  tunnel: w1945 -> [_ w1971]
                  tunnel: w1944 -> [_ w1968]
                  tunnel: w1943 -> [w1949 w1958]
                  tunnel: [w1949 w1967] -> w1941
                  tunnel: [w1951 w1966] -> w1942
                  tunnel: [w1951 w1965] -> _
                  tunnel: [u16 0 w1964] -> w1940
                  tunnel: w1939 -> [_ w1960]
                  tunnel: w1936 -> [w1948 _]
                  tunnel: [w1947 0] -> w1933
                  frame False {
                    w1951 = FALSE
                    # "Increment timeout"
                    n554 = Increment(x=w1948) -> (x+1=w1947:i32)
                  }
                  frame True {
                    # "******"
                    # "Determine Direction of Move"
                    # "Convert Track Angle to UINT16"
                    # "1024/300"
                    # "Move to Tracking Angle \n\nif delta is greater than move servo threshold\nAND less than max move threshold"
                    n555 = Add(x=w1971, y=w1954) -> (x+y=w1974:sgl)
                    n556 = local read "Last Track Angle - L"() -> (w1953:sgl)
                    n557 = Add(x=w1974, y=sgl 60.0) -> (x+y=w1973:sgl)
                    n558 = Multiply(x=3.413333333333333, y=w1973) -> (x*y=w1952:dbl)
                    n559 = To Word Integer(number=w1958) -> (16bit integer=w1956:i16)
                    n560 = To Unsigned Word Integer(number=w1952) -> (unsigned 16bit integer=w1970:u16)
                    n561 = To Word Integer(number=w1952) -> (16bit integer=w1969:i16)
                    n562 = Subtract(x=w1952, y=w1953) -> ()  [unwired: 1 out]
                    n563 = Subtract(x=w1969, y=w1956) -> (x-y=w1959:i16)
                    n564 = Absolute Value(x=w1959) -> (abs(x)=w1955:i16)
                    n565 = Greater Or Equal?(x=w1955, y=w1968) -> (x >= y?=w1962:bool)
                    n566 = Less Or Equal?(x=w1955, y=w1960) -> (x <= y?=w1961:bool)
                    n567 = And(x=w1962, y=w1961) -> (x .and. y?=w1963:bool)
                    n568 = case shown="True" w1963 {
                      tunnel: w1970 -> [_ w1982]
                      tunnel: [w1977 w1982] -> w1967
                      tunnel: [w1978 w1988] -> w1966
                      tunnel: [w1978 w1988] -> w1965
                      tunnel: w1958 -> [w1977 _]
                      tunnel: w1955 -> [_ w1987]
                      tunnel: [u16 0 w1987] -> w1964
                      tunnel: w1954 -> [_ w1981]
                      frame False {
                        w1978 = FALSE
                        # "Don't Move"
                      }
                      frame True {
                        w1988 = TRUE
                        # "45 DEG MOUNT OFFSET"
                        # "1024/300"
                        # "Current Delta"
                        # "Use new Track Angle"
                        n569 = Divide(x=w1982, y=3.413333333333333) -> (x/y=w1984:dbl)
                        n570 = Negate(x=w1981) -> (-x=w1980:sgl)
                        n571 = Subtract(x=w1984, y=sgl 60.0) -> (x-y=w1986:dbl)
                        n572 = Add(x=w1986, y=w1980) -> (x+y=w1979:dbl)
                        n573 = local write "Last Track Angle - L"(w1979) -> ()
                      }
                    }
                  }
                }
                n574 = local read "Timeout to \nEnable Reactive Predict"() -> (w1934:u16)
                n575 = Less?(x=w1933, y=w1934) -> (x < y?=w1932:bool)
                n576 = case shown="True" w1932 {
                  tunnel: [enum16{"Track", "Reactive Predict", ""}."Reactive Predict" ("Initial Tracking State - Right") enum16{"Track", "Reactive Predict", ""}."Track" ("Initial Tracking State - Right")] -> w1931
                  frame False {
                  }
                  frame True {
                  }
                }
              }
              frame "Reactive Predict" {
                # "Choose New\nTracking State"
                n577 = Or(x=w1992, y=w1995) -> (x .or. y?=w1991:bool)
                n578 = case shown="False" w1991 {
                  tunnel: [w2021 w2074] -> w2008
                  tunnel: w2007 -> [w2020 _]
                  tunnel: w2006 -> [w2019 _]
                  tunnel: w2005 -> [w2018 _]
                  tunnel: w2004 -> [w2017 _]
                  tunnel: w2003 -> [w2016 _]
                  tunnel: w2001 -> [w2015 _]
                  tunnel: [w2014 FALSE] -> w2000
                  tunnel: [w2013 TRUE] -> w1998
                  tunnel: w1997 -> [w2012 _]
                  tunnel: [w2011 0] -> w1996
                  tunnel: [enum16{"Track", "Reactive Predict", ""}."Reactive Predict" ("Initial Tracking State - Right") enum16{"Track", "Reactive Predict", ""}."Track" ("Initial Tracking State - Right")] -> w1994
                  tunnel: w2002 -> [w2009 w2074]
                  frame False {
                    # "Stay in Reactive State"
                    # "Increment Track Timeout"
                    # "Move Respond Flag"
                    n579 = Increment(x=w2012) -> (x+1=w2011:i32)
                    n580 = case shown="False" w2016 {
                      tunnel: w2020 -> [_ w2036]
                      tunnel: w2019 -> [_ w2035]
                      tunnel: w2018 -> [_ w2034]
                      tunnel: w2017 -> [_ w2033]
                      tunnel: w2015 -> [_ w2030]
                      tunnel: [w2022 w2026] -> w2021
                      tunnel: [w2023 w2025] -> w2014
                      tunnel: [w2023 w2025] -> w2013
                      tunnel: w2009 -> [w2022 w2024]
                      frame False {
                        w2023 = FALSE
                        # "Reset Move Respond = F"
                        # "Move Servo = F"
                      }
                      frame True {
                        w2025 = TRUE
                        # "Position Lock"
                        # "Current Servo\nPosition"
                        # "Reset Move\nRespond = T"
                        # "Move Servo = T"
                        # "Apply Direction \nto Offset (delta sum)"
                        # "Check Last Known Position of Robot"
                        n581 = case shown="True" w2036 {
                          tunnel: w2035 -> [_ w2064]
                          tunnel: w2034 -> [_ w2039]
                          tunnel: w2033 -> [_ w2040]
                          tunnel: [sgl 1.0 ("y") w2038] -> w2032
                          frame False {
                            # "No Position Data Available"
                            # "Default is to move\nSame Direction as other\nServo"
                          }
                          frame True {
                            w2045 = sgl 1.0 ("y")
                            # "Use previous position/orientation to Guess Which Direction to Move Servo"
                            # "Choose Search Direction"
                            # "\"Perpendicular \nThreshold\""
                            # "If Orientation is\n ~Perpendicular -> Start Search\n in Opposite Direction of Other"
                            # "****add 90 until orientation angle is fixed"
                            # "Last Orientation"
                            # "Convert to Rad"
                            # "Avoid Divide by 0"
                            # "-1/m"
                            # "Calculate Normal Line to \nLast Robot Position\nfrom Center Beacon"
                            # "last Position \nCoordinates"
                            n582 = Unbundle(w2064) -> ("X"=w2044:sgl, "Y"=w2043:sgl)
                            n583 = Unbundle(w2040) -> ("X"=w2042:sgl, "Y"=w2041:sgl)
                            n584 = Subtract(x=w2043, y=w2041) -> (x-y=w2060:sgl)
                            n585 = Subtract(x=w2044, y=w2042) -> (x-y=w2058:sgl)
                            n586 = Equal To 0?(x=w2058) -> (x = 0?=w2059:bool)
                            n587 = case shown="False" w2059 {
                              tunnel: w2060 -> [w2067 _]
                              tunnel: w2058 -> [w2066 _]
                              tunnel: [w2065 1000000000000000.0] -> w2057
                              frame False {
                                n588 = Divide(x=w2067, y=w2066) -> (x/y=w2065:sgl)
                              }
                              frame True {
                              }
                            }
                            n589 = Equal To 0?(x=w2057) -> (x = 0?=w2062:bool)
                            n590 = case shown="False" w2062 {
                              tunnel: [w2069 1e-08] -> w2061
                              tunnel: w2057 -> [w2069 _]
                              frame False {
                              }
                              frame True {
                                # "Can't have infinit slope"
                              }
                            }
                            n591 = Divide(x=-1.0, y=w2061) -> (x/y=w2056:dbl)
                            n592 = Inverse Tangent(1:w2056) -> (0:w2054:dbl)
                            n593 = expression code="(x/pi)*180.0" "radians to degrees"(w2054) -> (w2055:dbl)
                            n594 = To Single Precision Float(number=w2055) -> (single precision float=w2052:sgl)
                            n595 = Add(x=w2039, y=sgl 90.0) -> (x+y=w2051:sgl)
                            n596 = Subtract(x=w2052, y=w2051) -> (x-y=w2050:sgl)
                            n597 = Absolute Value(x=w2050) -> (abs(x)=w2049:sgl)
                            n598 = Less Or Equal?(x=w2049, y=sgl 10.0) -> (x <= y?=w2047:bool)
                            n599 = Negate(x=w2045) -> (-x=w2046:sgl)
                            n600 = Select(t=w2046, s=w2047, f=w2045) -> (s? t:f=w2038:sgl)
                          }
                        }
                        n601 = To Word Integer(number=w2032) -> (16bit integer=w2031:i16)
                        n602 = Multiply(x=w2031, y=w2030) -> (x*y=w2029:i32)
                        n603 = To Word Integer(number=w2024) -> (16bit integer=w2028:i16)
                        n604 = Add(x=w2029, y=w2028) -> (x+y=w2027:i32)
                        n605 = To Unsigned Word Integer(number=w2027) -> (unsigned 16bit integer=w2026:u16)
                      }
                    }
                  }
                  frame True {
                    # "Either Current Angle Valid or Image Lock Acheived"
                    # "Go Directly to Track State"
                  }
                }
              }
            }
            n606 = local read "Tracking Timeout\nThreshold"() -> (w1915:i32)
            n607 = Less?(x=w1909, y=w1915) -> (x < y?=w1916:bool)
            n608 = case shown="True" w1916 {
              tunnel: [T5."Recovery Mode" ("Next Main State") T5."Tracking" ("Next Main State")] -> w1920
              frame False {
              }
              frame True {
              }
            }
          }
          frame "Recovery Mode" {
            w2084 = u16 0
            # "Recovery Search Move Count"
            # "***Compltetly resets as of R17, used to just reset to \"Max Recovery Count - 1\""
            # "Increment Recoveyr Mode Count"
            # "Frames Processed"
            # "Choose Next Main State"
            # "Reset recovery count"
            # "Recovery move\nCount"
            # "Recovery Search\nAttempt count"
            # "Move Servo = T"
            # "delta move sum"
            # "Robot Position Valid"
            n609 = local read "Image Lock - Right"() -> (w2088:bool)
            n610 = case shown="\"Recovery Search\"" w2081 {
              tunnel: w2110 -> [_ _]
              tunnel: w2109 -> [_ _]
              tunnel: w2108 -> [_ _]
              tunnel: w2107 -> [_ _]
              tunnel: w2106 -> [_ _]
              tunnel: w2105 -> [_ _]
              tunnel: w2104 -> [w2138 w2224]
              tunnel: [w2130 w2222] -> w2103
              tunnel: [w2127 w2216] -> w2102
              tunnel: [FALSE FALSE] -> w2082
              tunnel: [w2132 w2214] -> w2101
              tunnel: w2098 -> [w2136 _]
              tunnel: w2100 -> [w2139 _]
              tunnel: w2099 -> [w2137 w2219]
              tunnel: [w2129 w2213] -> w2096
              tunnel: [w2128 w2213] -> w2097
              tunnel: w2088 -> [w2126 _]
              tunnel: [w2117 w2223] -> w2095
              tunnel: w2094 -> [w2115 w2211]
              tunnel: w2093 -> [w2120 w2220]
              tunnel: w2092 -> [w2116 w2218]
              tunnel: w2078 -> [_ _]
              tunnel: w2080 -> [_ _]
              tunnel: [FALSE w2215] -> w2090
              tunnel: w2087 -> [w2124 _]
              tunnel: w2086 -> [w2123 _]
              tunnel: [w2120 w2212] -> w2085
              tunnel: w2078 -> [_ w2209]
              frame "Recovery Search" {
                # "Wait for 2 Images to be Processed\nBefore Going to Next Step"
                # "Choose Next Reovery State"
                # "Recovery Search \nAttempt Count"
                # "Move Servo"
                # "Goal Position"
                # "Recovery Search\nmove Count"
                # "Attempt Recovery Search if Other Servo has Valid Angle"
                n611 = local read "Last Track Angle - R"() -> (w2119:sgl)
                n612 = Greater Or Equal?(x=w2115, y=w2116) -> (x >= y?=w2118:bool)
                n613 = case shown="True" w2118 {
                  tunnel: w2139 -> [_ w2159]
                  tunnel: [w2144 w2158] -> w2128
                  tunnel: w2138 -> [w2147 w2157]
                  tunnel: w2137 -> [_ w2156]
                  tunnel: [w2145 w2155] -> w2129
                  tunnel: [w2147 w2154] -> w2130
                  tunnel: [FALSE w2153] -> w2127
                  tunnel: w2124 -> [w2145 w2152]
                  tunnel: w2123 -> [w2144 w2151]
                  tunnel: w2126 -> [_ w2150]
                  tunnel: w2119 -> [_ w2149]
                  tunnel: [w2142 0 ("Frames Processed\nCount - in")] -> w2117
                  tunnel: w2115 -> [w2143 _]
                  frame False {
                    # "Increment Frames Processed"
                    # "WAIT"
                    n614 = Increment(x=w2143) -> (x+1=w2142:i32)
                  }
                  frame True {
                    n615 = case shown="True" w2150 {
                      tunnel: w2149 -> [_ w2172]
                      tunnel: w2152 -> [w2160 w2168]
                      tunnel: w2159 -> [_ w2173]
                      tunnel: [w2163 w2171] -> w2154
                      tunnel: [w2161 w2170] -> w2158
                      tunnel: w2151 -> [w2161 w2169]
                      tunnel: w2157 -> [w2163 w2167]
                      tunnel: w2156 -> [_ w2166]
                      tunnel: [FALSE TRUE] -> w2153
                      tunnel: [w2160 w2164] -> w2155
                      frame False {
                        # "Don't Move bc Other Servo Doesn't Have Image Lock"
                      }
                      frame True {
                        # "Move Servo = T"
                        n616 = Greater Than 0?(x=w2168) -> (x > 0?=w2174:bool)
                        n617 = case shown="False" w2174 {
                          tunnel: w2173 -> [w2183 _]
                          tunnel: w2172 -> [w2178 _]
                          tunnel: [w2175 w2193] -> w2171
                          tunnel: [w2181 w2199] -> w2170
                          tunnel: w2169 -> [w2182 w2199]
                          tunnel: w2168 -> [w2180 w2196]
                          tunnel: [w2179 w2198] -> w2164
                          tunnel: w2167 -> [_ w2194]
                          tunnel: w2166 -> [_ w2191]
                          frame False {
                            # "************************"
                            # "Increment move count to transition\nto Pan mode"
                            # "Increment Recovery Search Attempt Count"
                            # "1024/300"
                            # "Move Parallel to Other Servo"
                            n618 = Increment(x=w2182) -> (x+1=w2181:i32)
                            n619 = Add(x=w2178, y=w2183) -> (x+y=w2189:sgl)
                            n620 = Add(x=w2189, y=sgl 60.0) -> (x+y=w2188:sgl)
                            n621 = Multiply(x=3.413333333333333, y=w2188) -> (x*y=w2186:dbl)
                            n622 = Add(x=0.5, y=w2186) -> (x+y=w2184:dbl)
                            n623 = To Unsigned Word Integer(number=w2184) -> (unsigned 16bit integer=w2176:u16)
                            n624 = Increment(x=w2180) -> (x+1=w2179:i32)
                            n625 = Add(x=w2176, y="Recovery Parallel\nSearch Offset") -> (x+y=w2175:u16)
                          }
                          frame True {
                            # "Apply Direction"
                            # "Step SIze"
                            # "Current Position"
                            # "Attempt to Pan in Steps Towards other Servo"
                            # "Could be same or function of \nregular search step size"
                            # "Max # of Pan\nMoves"
                            # "Pan Towards Other Servo"
                            n626 = Greater Or Equal?(x=w2196, y="Max # Pan Moves") -> (x >= y?=w2197:bool)
                            n627 = case shown="False" w2197 {
                              tunnel: w2196 -> [w2207 _]
                              tunnel: [w2206 u16 0] -> w2198
                              frame False {
                                # "Increment Pan Count"
                                n628 = Increment(x=w2207) -> (x+1=w2206:i32)
                              }
                              frame True {
                                # "Reset move count"
                              }
                            }
                            n629 = local read "Recovery Search\nDirection - L"() -> (w2192:bool)
                            n630 = case shown="True" w2192 {
                              tunnel: w2194 -> [w2201 w2205]
                              tunnel: w2191 -> [w2202 w2204]
                              tunnel: [w2200 w2203] -> w2193
                              frame False {
                                # "CCW"
                                n631 = Add(x=w2201, y=w2202) -> (x+y=w2200:u16)
                              }
                              frame True {
                                # "CW"
                                n632 = Subtract(x=w2205, y=w2204) -> (x-y=w2203:u16)
                              }
                            }
                          }
                        }
                      }
                    }
                  }
                }
                n633 = local read "Max Recovery Count\n(Recovery Search)"() -> (w2121:u16)
                n634 = local read "Max Recovery\nSearch Attempts"() -> (w2122:u16)
                n635 = Less Or Equal?(x=w2128, y=w2122) -> (x <= y?=w2134:bool)
                n636 = Less Or Equal?(x=w2136, y=w2121) -> (x <= y?=w2135:bool)
                n637 = And(x=w2134, y=w2135) -> (x .and. y?=w2133:bool)
                n638 = case shown="True" w2133 {
                  tunnel: [enum16{"Generic Sweep", "Recovery Search"}."Generic Sweep" enum16{"Generic Sweep", "Recovery Search"}."Recovery Search"] -> w2132
                  frame False {
                  }
                  frame True {
                  }
                }
              }
              frame "Generic Sweep" {
                w2213 = u16 0
                # "Image Locked?"
                # "Choose Next Recovery State"
                # "Wait for 2 Images to be Processed\nBefore Going to Next Step"
                # "New Goal Position"
                # "Move Servo"
                # "Frames Processed Count"
                n639 = Greater Or Equal?(x=w2211, y=w2218) -> (x >= y?=w2225:bool)
                n640 = case shown="True" w2225 {
                  tunnel: w2224 -> [w2241 w2247]
                  tunnel: w2219 -> [_ w2256]
                  tunnel: w2220 -> [w2240 w2255]
                  tunnel: [w2241 w2245] -> w2222
                  tunnel: [w2239 0] -> w2223
                  tunnel: [FALSE TRUE] -> w2217
                  tunnel: w2211 -> [w2242 _]
                  tunnel: [w2240 w2249] -> w2212
                  frame False {
                    # "Increment Frames Processed"
                    n641 = Increment(x=w2242) -> (x+1=w2239:i32)
                  }
                  frame True {
                    # "Reset Frames\nProcessed Count"
                    # "SWEEP SEARCH - Startup"
                    # "Multiple New Step\nby Step SIze"
                    # "F = CCW\nT = CW"
                    # "Last Direction"
                    # "Min Step"
                    # "add 10 in case\nactual position\nis lower than GP"
                    # "Set New Step #"
                    # "Choose Direction"
                    # "Nearest step"
                    # "Adjust Actual Posiiton\n to pre-determiend steps"
                    # "Move Servo 1 \"Step\" to\nSearch"
                    n642 = Subtract(x=w2247, y=200) -> (x-y=w2248:i32)
                    n643 = Add(x=5, y=w2248) -> (x+y=w2263:i32)
                    n644 = Quotient & Remainder(x=w2263, y=w2256) -> (floor(x/y)=w2261:i32)  [unwired: 1 out]
                    n645 = To Byte Integer(number=w2261) -> (8bit integer=w2253:i8)
                    n646 = Less?(x=w2253, y=1) -> (x < y?=w2258:bool)
                    n647 = case shown="False" w2258 {
                      tunnel: w2253 -> [w2274 w2282]
                      tunnel: [w2276 FALSE] -> w2249
                      tunnel: [w2275 w2282] -> w2260
                      tunnel: w2255 -> [w2273 _]
                      tunnel: w2256 -> [w2271 _]
                      frame False {
                        # "Max Step"
                        # "# of steps\nminus 1"
                        n648 = Divide(x=300, y=w2271) -> (x/y=w2268:dbl)
                        n649 = To Unsigned Byte Integer(number=w2268) -> (unsigned 8bit integer=w2269:u8)
                        n650 = Greater Or Equal?(x=w2274, y=w2269) -> (x >= y?=w2270:bool)
                        n651 = case shown="True" w2270 {
                          tunnel: [w2277 TRUE] -> w2276
                          tunnel: [w2278 w2279] -> w2275
                          tunnel: w2274 -> [w2278 w2279]
                          tunnel: w2273 -> [w2277 _]
                          frame False {
                            # "No Need to\nChange Direction"
                          }
                          frame True {
                            # "T"
                            # "Move CW"
                          }
                        }
                      }
                      frame True {
                        # "F"
                        # "Move CCW"
                      }
                    }
                    n652 = case shown="True" w2249 {
                      tunnel: w2260 -> [w2265 w2266]
                      tunnel: [w2264 w2267] -> w2257
                      frame False {
                        # "CCW\n+1"
                        n653 = Increment(x=w2265) -> (x+1=w2264:i8)
                      }
                      frame True {
                        # "CW\n-1"
                        n654 = Decrement(x=w2266) -> (x-1=w2267:i8)
                      }
                    }
                    n655 = Multiply(x=w2257, y=w2256) -> (x*y=w2254:u16)
                    n656 = To Unsigned Word Integer(number=w2254) -> (unsigned 16bit integer=w2252:u16)
                    n657 = Add(x=w2252, y=200) -> (x+y=w2245:i32)
                  }
                }
                n658 = local read "Image Lock - Right"() -> (w2210:bool)
                n659 = case shown="True" w2209 {
                  tunnel: [w2228 w2238] -> w2216
                  tunnel: w2217 -> [w2229 _]
                  tunnel: [w2230 enum16{"Generic Sweep", "Recovery Search"}."Generic Sweep"] -> w2214
                  tunnel: [w2227 w2238] -> w2215
                  tunnel: w2210 -> [w2226 _]
                  frame False {
                    # "Is other servo tracking?"
                    n660 = case shown="True" w2226 {
                      tunnel: [enum16{"Generic Sweep", "Recovery Search"}."Generic Sweep" enum16{"Generic Sweep", "Recovery Search"}."Recovery Search"] -> w2230
                      tunnel: w2229 -> [w2233 _]
                      tunnel: [w2233 FALSE] -> w2228
                      tunnel: [FALSE TRUE] -> w2227
                      frame False {
                        # "Stay in Sweep"
                      }
                      frame True {
                        # "G o to Recovery Search  State"
                      }
                    }
                  }
                  frame True {
                    w2238 = FALSE
                    # "Override Move Servo\nCommand bc an Angle Was Found\nduring this Step"
                    # "Stay In Sweep\nLet Main State Machine transition\ninto Tracking"
                  }
                }
              }
            }
            n661 = Increment(x=w2098) -> (x+1=w2079:i32)
            n662 = case shown="False" w2090 {
              tunnel: w2079 -> [w2113 _]
              tunnel: [w2113 0] -> w2091
              frame False {
              }
              frame True {
              }
            }
            n663 = case shown="False" w2078 {
              tunnel: [T5."Recovery Mode" ("Next Main State") T5."Tracking" ("Next Main State")] -> w2089
              frame False {
              }
              frame True {
              }
            }
          }
        }
        "Current Move Delta - L" <- w1823
        n664 = Less?(x=w1850, y=w1849) -> (x < y?=w1848:bool)
        n665 = local write "New Data  Flag\nLeft Servo"(FALSE) -> ()
        n666 = Select(t=w1849, s=w1848, f=w1850) -> (s? t:f=w1845:i32)
        n667 = Greater?(x=w1845, y=w1846) -> (0:w1847:bool)
        n668 = Select(t=w1846, s=w1847, f=w1845) -> (s? t:f=w1844:i32)
      }
    }
    "Next Main State - Left" <- w1255
    "Next Tracking State - Left" <- w1238
    "Next Recovery State - Left" <- w1236
    n669 = case shown="True" w1219 {
      tunnel: [w1304 w1342] -> w1189
      tunnel: [w1298 w1341] -> w1188
      tunnel: w1224 -> [w1299 w1340]
      tunnel: w1221 -> [_ w1339]
      tunnel: "Track Angle Valid  - Right" -> [_ w1338]
      tunnel: w1218 -> [_ w1337]
      tunnel: w1217 -> [w1304 w1336]
      tunnel: "Mounting Offset - Right" -> [_ w1335]
      tunnel: w1212 -> [w1295 w1334]
      tunnel: w1210 -> [_ w1333]
      tunnel: w1207 -> [w1296 w1332]
      tunnel: w1205 -> [_ w1331]
      tunnel: w1204 -> [_ w1330]
      tunnel: w1203 -> [_ w1329]
      tunnel: w1202 -> [_ w1328]
      tunnel: w1200 -> [w1294 w1327]
      tunnel: w1209 -> [w1293 w1326]
      tunnel: w1208 -> [w1297 w1325]
      tunnel: w1214 -> [_ w1324]
      tunnel: w1213 -> [_ w1323]
      tunnel: w1211 -> [_ w1322]
      tunnel: [0 w1321] -> w1190
      tunnel: [w1299 w1320] -> w1187
      tunnel: [w1298 w1319] -> w1194
      tunnel: [w1297 w1318] -> w1195
      tunnel: [w1293 w1317] -> w1196
      tunnel: [w1296 w1316] -> w1197
      tunnel: [w1294 w1315] -> w1198
      tunnel: w1201 -> [_ w1314]
      tunnel: [w1295 w1313] -> w1199
      tunnel: w1206 -> [_ w1312]
      tunnel: w1216 -> [w1302 w1311]
      tunnel: w1222 -> [w1301 w1310]
      tunnel: [w1302 w1309] -> w1191
      tunnel: [w1301 w1308] -> w1193
      tunnel: w1223 -> [w1300 w1307]
      tunnel: [w1300 w1306] -> w1192
      frame False {
        w1298 = FALSE
        # "Recovery Mode COunt"
        # "Frames Processed - L"
        # "Recovery Search move Count - L"
        # "Recovery Search Attempt Count- L"
        # "WAITING FOR NEW IMAGE, RETAIN ALL VALUES"
      }
      frame True {
        w1344 = u16 1023
        w1347 = u16 0
        # "New Tracking State"
        # "Tracking Timeout Count"
        # "Next Main State"
        # "Next Recovery State"
        # "Reset Respond"
        # "Search Direction"
        # "Recovery Count"
        # "Recovery Search move Count"
        # "Recovery Search Attempt Count"
        # "Frames Processed"
        # "Apply Floor/Ceiling to Goal Position"
        # "Current move Delta"
        # "Service Track Angle Flag"
        # "Move Servo"
        # "Goal Position"
        # "Go to Current State"
        n670 = case shown="\"Recovery Mode\"" w1340 {
          tunnel: w1336 -> [w1365 w1437 w1616]
          tunnel: w1337 -> [_ w1439 _]
          tunnel: w1322 -> [w1364 _ w1611]
          tunnel: w1334 -> [w1363 w1420 w1605]
          tunnel: [w1362 w1435 w1615] -> w1348
          tunnel: [w1360 w1436 w1614] -> w1341
          tunnel: w1338 -> [_ w1430 w1592]
          tunnel: [w1358 w1432 w1601] -> w1320
          tunnel: w1339 -> [w1349 w1431 w1590]
          tunnel: w1335 -> [_ w1440 w1612]
          tunnel: w1324 -> [_ w1438 _]
          tunnel: [w1352 w1434 w1596] -> w1321
          tunnel: w1323 -> [_ w1433 _]
          tunnel: w1332 -> [w1357 _ w1606]
          tunnel: [enum16{"Generic Sweep", "Recovery Search"}."Recovery Search" enum16{"Generic Sweep", "Recovery Search"}."Recovery Search" w1613] -> w1306
          tunnel: w1327 -> [_ _ w1610]
          tunnel: w1307 -> [_ _ w1593]
          tunnel: w1333 -> [_ w1417 w1622]
          tunnel: w1314 -> [_ w1413 w1617]
          tunnel: w1329 -> [_ w1423 w1619]
          tunnel: w1330 -> [_ w1424 w1620]
          tunnel: w1331 -> [_ w1425 w1621]
          tunnel: w1328 -> [_ w1422 w1618]
          tunnel: [FALSE w1419 w1594] -> w1319
          tunnel: w1312 -> [w1356 _ w1604]
          tunnel: [w1352 w1414 w1603] -> w1315
          tunnel: [w1352 w1414 w1609] -> w1318
          tunnel: [w1352 w1414 w1608] -> w1317
          tunnel: [w1355 w1415 w1607] -> w1316
          tunnel: w1326 -> [_ _ w1599]
          tunnel: w1325 -> [_ _ w1598]
          tunnel: [w1353 w1420 w1597] -> w1313
          tunnel: w1311 -> [_ w1429 _]
          tunnel: [w1352 w1421 w1596] -> w1309
          tunnel: w1310 -> [_ w1426 _]
          tunnel: [enum16{"Track", "Reactive Predict", ""}."Track" ("Initial Tracking State - Right") w1418 enum16{"Track", "Reactive Predict", ""}."Track" ("Initial Tracking State - Right")] -> w1308
          frame "Start Up Search", Default {
            w1352 = u16 0
            # "Image Lock"
            # "Search Direction"
            # "Wait for 'x' Images to be Processed\nBefore Going to Next Step"
            # "Next Main State"
            # "New Goal Position"
            # "Move Servo"
            # "Choose Next State"
            # "Frames Processed Count"
            n671 = Greater Or Equal?(x=w1357, y=w1356) -> (x >= y?=w1361:bool)
            n672 = case shown="True" w1361 {
              tunnel: w1365 -> [w1375 w1387]
              tunnel: w1364 -> [_ w1385]
              tunnel: w1363 -> [w1374 w1384]
              tunnel: [w1375 w1381] -> w1362
              tunnel: [w1373 0] -> w1355
              tunnel: [FALSE TRUE] -> w1359
              tunnel: w1357 -> [w1376 _]
              tunnel: [w1374 w1378] -> w1353
              frame False {
                # "Wait until Min Number of Frames (per search/step) Processed"
                # "Increase Frames\nProcessed Count"
                n673 = Increment(x=w1376) -> (x+1=w1373:i32)
              }
              frame True {
                # "Reset Frames\nProcessed Count"
                # "SWEEP SEARCH - Startup"
                # "Multiple New Step\nby Step SIze"
                # "F = CCW\nT = CW"
                # "Last Direction"
                # "Min Step"
                # "add in case\nactual position\nis lower than GP"
                # "Set New Step #"
                # "Choose Direction"
                # "Nearest step"
                # "Adjust Actual Posiiton\n to pre-determiend steps"
                # "Move Servo 1 \"Step\" to\nSearch"
                n674 = Add(x=3, y=w1387) -> (x+y=w1393:i32)
                n675 = Quotient & Remainder(x=w1393, y=w1385) -> (floor(x/y)=w1391:i32)  [unwired: 1 out]
                n676 = To Byte Integer(number=w1391) -> (8bit integer=w1382:i8)
                n677 = Less?(x=w1382, y=1) -> (x < y?=w1388:bool)
                n678 = case shown="False" w1388 {
                  tunnel: w1382 -> [w1404 w1412]
                  tunnel: [w1406 FALSE] -> w1378
                  tunnel: [w1405 w1412] -> w1390
                  tunnel: w1384 -> [w1403 _]
                  tunnel: w1385 -> [w1401 _]
                  frame False {
                    # "Max Step"
                    # "# of steps\nminus 1"
                    n679 = Divide(x=1024, y=w1401) -> (x/y=w1398:dbl)
                    n680 = To Unsigned Byte Integer(number=w1398) -> (unsigned 8bit integer=w1399:u8)
                    n681 = Greater Or Equal?(x=w1404, y=w1399) -> (x >= y?=w1400:bool)
                    n682 = case shown="True" w1400 {
                      tunnel: [w1407 TRUE] -> w1406
                      tunnel: [w1408 w1409] -> w1405
                      tunnel: w1404 -> [w1408 w1409]
                      tunnel: w1403 -> [w1407 _]
                      frame False {
                        # "No Need to\nChange Direction"
                      }
                      frame True {
                        # "T"
                        # "Move CW"
                      }
                    }
                  }
                  frame True {
                    # "F"
                    # "Move CCW"
                  }
                }
                n683 = case shown="False" w1378 {
                  tunnel: w1390 -> [w1395 w1396]
                  tunnel: [w1394 w1397] -> w1386
                  frame False {
                    # "CCW\n+1"
                    n684 = Increment(x=w1395) -> (x+1=w1394:i8)
                  }
                  frame True {
                    # "CW\n-1"
                    n685 = Decrement(x=w1396) -> (x-1=w1397:i8)
                  }
                }
                n686 = Multiply(x=w1386, y=w1385) -> (x*y=w1383:u16)
                n687 = To Unsigned Word Integer(number=w1383) -> (unsigned 16bit integer=w1381:u16)
              }
            }
            n688 = case shown="False" w1349 {
              tunnel: [w1367 FALSE] -> w1360
              tunnel: w1359 -> [w1367 _]
              tunnel: [w1368 T5."Tracking" ("Next Main State")] -> w1358
              frame False {
                # "Check other Servo\nStay in Startup  State"
                n689 = local read "Image Lock - Left"() -> (w1366:bool)
                n690 = case shown="False" w1366 {
                  tunnel: [T5."Start Up Search" ("Next Main State") T5."Recovery Mode" ("Next Main State")] -> w1368
                  frame False {
                  }
                  frame True {
                  }
                }
              }
              frame True {
                # "Override Move Servo\nCommand bc an Angle Was Found\nduring this Step"
                # "Transition to Tracking State When\nImage Processing has Locked"
              }
            }
          }
          frame "Tracking" {
            w1414 = 0
            # "Frames Processed Count"
            # "Image Lock - L"
            # "Track Angle Valid"
            # "Tracking Angle"
            # "Tracking Timeout Count"
            # "Max ove delta"
            # "Move delta threshold"
            # "mount offset"
            # "Current Position"
            # "Move Respond"
            # "Trackin Timeout count"
            # "Move Servo"
            # "delta"
            # "GP"
            # "Reset Move Respond"
            # "New Tracking State"
            # "Delta Move Sum"
            # "Choose Next State"
            n691 = case shown="\"Track\", Default" w1426 {
              tunnel: w1440 -> [w1458 _]
              tunnel: w1439 -> [w1457 _]
              tunnel: w1438 -> [w1456 _]
              tunnel: w1437 -> [w1455 w1514]
              tunnel: [w1454 w1512] -> w1436
              tunnel: [w1453 w1520] -> w1435
              tunnel: [w1452 0] -> w1434
              tunnel: w1433 -> [w1451 _]
              tunnel: w1431 -> [w1450 w1504]
              tunnel: w1430 -> [w1449 w1507]
              tunnel: w1429 -> [w1448 w1509]
              tunnel: w1425 -> [_ w1519]
              tunnel: w1424 -> [_ w1518]
              tunnel: w1423 -> [_ w1517]
              tunnel: w1422 -> [_ w1516]
              tunnel: w1417 -> [_ w1515]
              tunnel: w1413 -> [_ w1513]
              tunnel: [TRUE w1510] -> w1419
              tunnel: [w1445 w1508] -> w1421
              tunnel: [w1443 w1506] -> w1418
              tunnel: [0 0] -> w1415
              frame "Track", Default {
                # "Reset"
                # "Tracking Timeout"
                # "Move Delta"
                # "Goal Position"
                # "Tracking Move"
                # "Move Servo"
                # "Only Consider Tracking Angle\n\nIF\n\nImage Locked        == T\nTrack Angle Flag   == T"
                n692 = And(x=w1450, y=w1449) -> (x .and. y?=w1442:bool)
                n693 = case shown="True" w1442 {
                  tunnel: w1458 -> [_ w1466]
                  tunnel: w1457 -> [_ w1483]
                  tunnel: w1456 -> [_ w1480]
                  tunnel: w1455 -> [w1461 w1470]
                  tunnel: [w1461 w1479] -> w1453
                  tunnel: [w1463 w1478] -> w1454
                  tunnel: [w1463 w1477] -> _
                  tunnel: [u16 0 w1476] -> w1452
                  tunnel: w1451 -> [_ w1472]
                  tunnel: w1448 -> [w1460 _]
                  tunnel: [w1459 0] -> w1445
                  frame False {
                    w1463 = FALSE
                    # "Increment timeout"
                    n694 = Increment(x=w1460) -> (x+1=w1459:i32)
                  }
                  frame True {
                    # "******"
                    # "Determine Direction of Move"
                    # "Convert Track Angle to UINT16"
                    # "1024/300"
                    # "Move to Tracking Angle \n\nif delta is greater than move servo threshold\nAND less than max move threshold"
                    n695 = Add(x=w1483, y=w1466) -> (x+y=w1486:sgl)
                    n696 = local read "Last Track Angle - R"() -> (w1465:sgl)
                    n697 = Add(x=w1486, y=sgl 60.0) -> (x+y=w1485:sgl)
                    n698 = Multiply(x=3.413333333333333, y=w1485) -> (x*y=w1464:dbl)
                    n699 = To Word Integer(number=w1470) -> (16bit integer=w1468:i16)
                    n700 = To Unsigned Word Integer(number=w1464) -> (unsigned 16bit integer=w1482:u16)
                    n701 = To Word Integer(number=w1464) -> (16bit integer=w1481:i16)
                    n702 = Subtract(x=w1464, y=w1465) -> ()  [unwired: 1 out]
                    n703 = Subtract(x=w1481, y=w1468) -> (x-y=w1471:i16)
                    n704 = Absolute Value(x=w1471) -> (abs(x)=w1467:i16)
                    n705 = Greater Or Equal?(x=w1467, y=w1480) -> (x >= y?=w1474:bool)
                    n706 = Less Or Equal?(x=w1467, y=w1472) -> (x <= y?=w1473:bool)
                    n707 = And(x=w1474, y=w1473) -> (x .and. y?=w1475:bool)
                    n708 = case shown="False" w1475 {
                      tunnel: w1482 -> [_ w1494]
                      tunnel: [w1489 w1494] -> w1479
                      tunnel: [w1490 w1500] -> w1478
                      tunnel: [w1490 w1500] -> w1477
                      tunnel: w1470 -> [w1489 _]
                      tunnel: w1467 -> [_ w1499]
                      tunnel: [u16 0 w1499] -> w1476
                      tunnel: w1466 -> [_ w1493]
                      frame False {
                        w1490 = FALSE
                        # "Don't Move"
                      }
                      frame True {
                        w1500 = TRUE
                        # "45 DEG MOUNT OFFSET"
                        # "1024/300"
                        # "Current Delta"
                        # "Use new Track Angle"
                        n709 = Divide(x=w1494, y=3.413333333333333) -> (x/y=w1496:dbl)
                        n710 = Negate(x=w1493) -> (-x=w1492:sgl)
                        n711 = Subtract(x=w1496, y=sgl 60.0) -> (x-y=w1498:dbl)
                        n712 = Add(x=w1498, y=w1492) -> (x+y=w1491:dbl)
                        n713 = local write "Last Track Angle - R"(w1491) -> ()
                      }
                    }
                  }
                }
                n714 = local read "Timeout to \nEnable Reactive Predict"() -> (w1446:u16)
                n715 = Less?(x=w1445, y=w1446) -> (x < y?=w1444:bool)
                n716 = case shown="True" w1444 {
                  tunnel: [enum16{"Track", "Reactive Predict", ""}."Reactive Predict" ("Initial Tracking State - Right") enum16{"Track", "Reactive Predict", ""}."Track" ("Initial Tracking State - Right")] -> w1443
                  frame False {
                  }
                  frame True {
                  }
                }
              }
              frame "Reactive Predict" {
                # "Choose New\nTracking State"
                n717 = Or(x=w1504, y=w1507) -> (x .or. y?=w1503:bool)
                n718 = case shown="False" w1503 {
                  tunnel: [w1533 w1586] -> w1520
                  tunnel: w1519 -> [w1532 _]
                  tunnel: w1518 -> [w1531 _]
                  tunnel: w1517 -> [w1530 _]
                  tunnel: w1516 -> [w1529 _]
                  tunnel: w1515 -> [w1528 _]
                  tunnel: w1513 -> [w1527 _]
                  tunnel: [w1526 FALSE] -> w1512
                  tunnel: [w1525 TRUE] -> w1510
                  tunnel: w1509 -> [w1524 _]
                  tunnel: [w1523 0] -> w1508
                  tunnel: [enum16{"Track", "Reactive Predict", ""}."Reactive Predict" ("Initial Tracking State - Right") enum16{"Track", "Reactive Predict", ""}."Track" ("Initial Tracking State - Right")] -> w1506
                  tunnel: w1514 -> [w1521 w1586]
                  frame False {
                    # "Stay in Reactive State"
                    # "Increment Track Timeout"
                    # "Move Respond Flag"
                    n719 = Increment(x=w1524) -> (x+1=w1523:i32)
                    n720 = case shown="True" w1528 {
                      tunnel: w1532 -> [_ w1548]
                      tunnel: w1531 -> [_ w1547]
                      tunnel: w1530 -> [_ w1546]
                      tunnel: w1529 -> [_ w1545]
                      tunnel: w1527 -> [_ w1542]
                      tunnel: [w1534 w1538] -> w1533
                      tunnel: [w1535 w1537] -> w1526
                      tunnel: [w1535 w1537] -> w1525
                      tunnel: w1521 -> [w1534 w1536]
                      frame False {
                        w1535 = FALSE
                        # "Reset Move Respond = F"
                        # "Move Servo = F"
                      }
                      frame True {
                        w1537 = TRUE
                        # "Position Lock"
                        # "Current Servo\nPosition"
                        # "Reset Move\nRespond = T"
                        # "Move Servo = T"
                        # "Apply Direction \nto Offset (delta sum)"
                        # "Check Last Known Position of Robot"
                        n721 = case shown="True" w1548 {
                          tunnel: w1547 -> [_ w1576]
                          tunnel: w1546 -> [_ w1551]
                          tunnel: w1545 -> [_ w1552]
                          tunnel: [sgl 1.0 ("y") w1550] -> w1544
                          frame False {
                            # "No Position Data Available"
                            # "Default is to move\nSame Direction as other\nServo"
                          }
                          frame True {
                            w1557 = sgl 1.0 ("y")
                            # "Use previous position/orientation to Guess Which Direction to Move Servo"
                            # "Choose Search Direction"
                            # "\"Perpendicular \nThreshold\""
                            # "If Orientation is\n ~Perpendicular -> Start Search\n in Opposite Direction of Other"
                            # "****add 90 until orientation angle is fixed"
                            # "Last Orientation"
                            # "Convert to Rad"
                            # "Avoid Divide by 0"
                            # "-1/m"
                            # "Calculate Normal Line to \nLast Robot Position\nfrom Center Beacon"
                            # "last Position \nCoordinates"
                            n722 = Unbundle(w1576) -> ("X"=w1556:sgl, "Y"=w1555:sgl)
                            n723 = Unbundle(w1552) -> ("X"=w1554:sgl, "Y"=w1553:sgl)
                            n724 = Subtract(x=w1555, y=w1553) -> (x-y=w1572:sgl)
                            n725 = Subtract(x=w1556, y=w1554) -> (x-y=w1570:sgl)
                            n726 = Equal To 0?(x=w1570) -> (x = 0?=w1571:bool)
                            n727 = case shown="False" w1571 {
                              tunnel: w1572 -> [w1579 _]
                              tunnel: w1570 -> [w1578 _]
                              tunnel: [w1577 1000000000000000.0] -> w1569
                              frame False {
                                n728 = Divide(x=w1579, y=w1578) -> (x/y=w1577:sgl)
                              }
                              frame True {
                              }
                            }
                            n729 = Equal To 0?(x=w1569) -> (x = 0?=w1574:bool)
                            n730 = case shown="False" w1574 {
                              tunnel: [w1581 1e-08] -> w1573
                              tunnel: w1569 -> [w1581 _]
                              frame False {
                              }
                              frame True {
                                # "Can't have infinit slope"
                              }
                            }
                            n731 = Divide(x=-1.0, y=w1573) -> (x/y=w1568:dbl)
                            n732 = Inverse Tangent(1:w1568) -> (0:w1566:dbl)
                            n733 = expression code="(x/pi)*180.0" "radians to degrees"(w1566) -> (w1567:dbl)
                            n734 = To Single Precision Float(number=w1567) -> (single precision float=w1564:sgl)
                            n735 = Add(x=w1551, y=sgl 90.0) -> (x+y=w1563:sgl)
                            n736 = Subtract(x=w1564, y=w1563) -> (x-y=w1562:sgl)
                            n737 = Absolute Value(x=w1562) -> (abs(x)=w1561:sgl)
                            n738 = Less Or Equal?(x=w1561, y=sgl 10.0) -> (x <= y?=w1559:bool)
                            n739 = Negate(x=w1557) -> (-x=w1558:sgl)
                            n740 = Select(t=w1558, s=w1559, f=w1557) -> (s? t:f=w1550:sgl)
                          }
                        }
                        n741 = To Word Integer(number=w1544) -> (16bit integer=w1543:i16)
                        n742 = Multiply(x=w1543, y=w1542) -> (x*y=w1541:i32)
                        n743 = To Word Integer(number=w1536) -> (16bit integer=w1540:i16)
                        n744 = Add(x=w1541, y=w1540) -> (x+y=w1539:i32)
                        n745 = To Unsigned Word Integer(number=w1539) -> (unsigned 16bit integer=w1538:u16)
                      }
                    }
                  }
                  frame True {
                    # "Either Current Angle Valid or Image Lock Acheived"
                    # "Go Directly to Track State"
                  }
                }
              }
            }
            n746 = local read "Tracking Timeout\nThreshold"() -> (w1427:i32)
            n747 = Less?(x=w1421, y=w1427) -> (x < y?=w1428:bool)
            n748 = case shown="True" w1428 {
              tunnel: [T5."Recovery Mode" ("Next Main State") T5."Tracking" ("Next Main State")] -> w1432
              frame False {
              }
              frame True {
              }
            }
          }
          frame "Recovery Mode" {
            w1596 = u16 0
            # "Recovery Search Move Count"
            # "***Compltetly resets as of R17, used to just reset to \"Max Recovery Count - 1\""
            # "Increment Recoveyr Mode Count"
            # "Frames Processed"
            # "Choose Next Main State"
            # "Reset recovery count"
            # "Recovery move\nCount"
            # "Recovery Search\nAttempt count"
            # "Move Servo = T"
            # "delta move sum"
            # "Robot Position Valid"
            n749 = local read "Image Lock - Left"() -> (w1600:bool)
            n750 = case shown="\"Recovery Search\"" w1593 {
              tunnel: w1622 -> [_ _]
              tunnel: w1621 -> [_ _]
              tunnel: w1620 -> [_ _]
              tunnel: w1619 -> [_ _]
              tunnel: w1618 -> [_ _]
              tunnel: w1617 -> [_ _]
              tunnel: w1616 -> [w1650 w1736]
              tunnel: [w1642 w1734] -> w1615
              tunnel: [w1639 w1728] -> w1614
              tunnel: [FALSE FALSE] -> w1594
              tunnel: [w1644 w1726] -> w1613
              tunnel: w1610 -> [w1648 _]
              tunnel: w1612 -> [w1651 _]
              tunnel: w1611 -> [w1649 w1731]
              tunnel: [w1641 w1725] -> w1608
              tunnel: [w1640 w1725] -> w1609
              tunnel: w1600 -> [w1638 _]
              tunnel: [w1629 w1735] -> w1607
              tunnel: w1606 -> [w1627 w1723]
              tunnel: w1605 -> [w1632 w1732]
              tunnel: w1604 -> [w1628 w1730]
              tunnel: w1590 -> [_ _]
              tunnel: w1592 -> [_ _]
              tunnel: [FALSE w1727] -> w1602
              tunnel: w1599 -> [w1636 _]
              tunnel: w1598 -> [w1635 _]
              tunnel: [w1632 w1724] -> w1597
              tunnel: w1590 -> [_ w1721]
              frame "Recovery Search" {
                # "Wait for 2 Images to be Processed\nBefore Going to Next Step"
                # "Choose Next Reovery State"
                # "Recovery Search \nAttempt Count"
                # "Move Servo"
                # "Goal Position"
                # "Recovery Search\nmove Count"
                # "Attempt Recovery Search if Other Servo has Valid Angle"
                n751 = local read "Last Track Angle - L"() -> (w1631:sgl)
                n752 = Greater Or Equal?(x=w1627, y=w1628) -> (x >= y?=w1630:bool)
                n753 = case shown="True" w1630 {
                  tunnel: w1651 -> [_ w1671]
                  tunnel: [w1656 w1670] -> w1640
                  tunnel: w1650 -> [w1659 w1669]
                  tunnel: w1649 -> [_ w1668]
                  tunnel: [w1657 w1667] -> w1641
                  tunnel: [w1659 w1666] -> w1642
                  tunnel: [FALSE w1665] -> w1639
                  tunnel: w1636 -> [w1657 w1664]
                  tunnel: w1635 -> [w1656 w1663]
                  tunnel: w1638 -> [_ w1662]
                  tunnel: w1631 -> [_ w1661]
                  tunnel: [w1654 0 ("Frames Processed\nCount - in")] -> w1629
                  tunnel: w1627 -> [w1655 _]
                  frame False {
                    # "Increment Frames Processed"
                    # "WAIT"
                    n754 = Increment(x=w1655) -> (x+1=w1654:i32)
                  }
                  frame True {
                    n755 = case shown="True" w1662 {
                      tunnel: w1661 -> [_ w1684]
                      tunnel: w1664 -> [w1672 w1680]
                      tunnel: w1671 -> [_ w1685]
                      tunnel: [w1675 w1683] -> w1666
                      tunnel: [w1673 w1682] -> w1670
                      tunnel: w1663 -> [w1673 w1681]
                      tunnel: w1669 -> [w1675 w1679]
                      tunnel: w1668 -> [_ w1678]
                      tunnel: [FALSE TRUE] -> w1665
                      tunnel: [w1672 w1676] -> w1667
                      frame False {
                        # "Don't Move bc Other Servo Doesn't Have Image Lock"
                      }
                      frame True {
                        # "Move Servo = T"
                        n756 = Greater Than 0?(x=w1680) -> (x > 0?=w1686:bool)
                        n757 = case shown="False" w1686 {
                          tunnel: w1685 -> [w1695 _]
                          tunnel: w1684 -> [w1690 _]
                          tunnel: [w1688 w1706] -> w1683
                          tunnel: [w1693 w1711] -> w1682
                          tunnel: w1681 -> [w1694 w1711]
                          tunnel: w1680 -> [w1692 w1708]
                          tunnel: [w1691 w1710] -> w1676
                          tunnel: w1679 -> [_ w1707]
                          tunnel: w1678 -> [_ w1704]
                          frame False {
                            # "************************"
                            # "Increment move count to transition\nto Pan mode"
                            # "Increment Recovery Search Attempt Count"
                            # "1024/300"
                            # "Move Parallel to Other Servo"
                            n758 = Increment(x=w1694) -> (x+1=w1693:i32)
                            n759 = Add(x=w1690, y=w1695) -> (x+y=w1701:sgl)
                            n760 = Add(x=w1701, y=sgl 60.0) -> (x+y=w1700:sgl)
                            n761 = Multiply(x=3.413333333333333, y=w1700) -> (x*y=w1698:dbl)
                            n762 = Add(x=0.5, y=w1698) -> (x+y=w1696:dbl)
                            n763 = To Unsigned Word Integer(number=w1696) -> (unsigned 16bit integer=w1689:u16)
                            n764 = Increment(x=w1692) -> (x+1=w1691:i32)
                            n765 = local read "Recovery Parallel\nSearch Offset"() -> (w1687:u16)
                            n766 = Subtract(x=w1689, y=w1687) -> (x-y=w1688:u16)
                          }
                          frame True {
                            # "Apply Direction"
                            # "Step SIze"
                            # "Current Position"
                            # "Attempt to Pan in Steps Towards other Servo"
                            # "Could be same or function of \nregular search step size"
                            # "Max # of Pan\nMoves"
                            # "Pan Towards Other Servo"
                            n767 = local read "Max # Pan Moves"() -> (w1703:u16)
                            n768 = Greater Or Equal?(x=w1708, y=w1703) -> (x >= y?=w1709:bool)
                            n769 = case shown="False" w1709 {
                              tunnel: w1708 -> [w1719 _]
                              tunnel: [w1718 u16 0] -> w1710
                              frame False {
                                # "Increment Pan Count"
                                n770 = Increment(x=w1719) -> (x+1=w1718:i32)
                              }
                              frame True {
                                # "Reset move count"
                              }
                            }
                            n771 = local read "Recovery Search\nDirection - R"() -> (w1705:bool)
                            n772 = case shown="True" w1705 {
                              tunnel: w1707 -> [w1713 w1717]
                              tunnel: w1704 -> [w1714 w1716]
                              tunnel: [w1712 w1715] -> w1706
                              frame False {
                                # "CCW"
                                n773 = Add(x=w1713, y=w1714) -> (x+y=w1712:u16)
                              }
                              frame True {
                                # "CW"
                                n774 = Subtract(x=w1717, y=w1716) -> (x-y=w1715:u16)
                              }
                            }
                          }
                        }
                      }
                    }
                  }
                }
                n775 = local read "Max Recovery Count\n(Recovery Search)"() -> (w1633:u16)
                n776 = local read "Max Recovery\nSearch Attempts"() -> (w1634:u16)
                n777 = Less Or Equal?(x=w1640, y=w1634) -> (x <= y?=w1646:bool)
                n778 = Less Or Equal?(x=w1648, y=w1633) -> (x <= y?=w1647:bool)
                n779 = And(x=w1646, y=w1647) -> (x .and. y?=w1645:bool)
                n780 = case shown="True" w1645 {
                  tunnel: [enum16{"Generic Sweep", "Recovery Search"}."Generic Sweep" enum16{"Generic Sweep", "Recovery Search"}."Recovery Search"] -> w1644
                  frame False {
                  }
                  frame True {
                  }
                }
              }
              frame "Generic Sweep" {
                w1725 = u16 0
                # "Image Locked?"
                # "Choose Next Recovery State"
                # "Wait for 2 Images to be Processed\nBefore Going to Next Step"
                # "New Goal Position"
                # "Move Servo"
                # "Frames Processed Count"
                n781 = Greater Or Equal?(x=w1723, y=w1730) -> (x >= y?=w1737:bool)
                n782 = case shown="True" w1737 {
                  tunnel: w1736 -> [w1753 w1769]
                  tunnel: w1731 -> [_ w1767]
                  tunnel: w1732 -> [w1752 w1766]
                  tunnel: [w1753 w1759] -> w1734
                  tunnel: [w1751 0] -> w1735
                  tunnel: [FALSE TRUE] -> w1729
                  tunnel: w1723 -> [w1754 _]
                  tunnel: [w1752 w1760] -> w1724
                  frame False {
                    # "Increment Frames Processed"
                    n783 = Increment(x=w1754) -> (x+1=w1751:i32)
                  }
                  frame True {
                    # "Reset Frames\nProcessed Count"
                    # "SWEEP SEARCH - Startup"
                    # "Multiple New Step\nby Step SIze"
                    # "F = CCW\nT = CW"
                    # "Last Direction"
                    # "Min Step"
                    # "add 10 in case\nactual position\nis lower than GP"
                    # "Set New Step #"
                    # "Choose Direction"
                    # "Nearest step"
                    # "Adjust Actual Posiiton\n to pre-determiend steps"
                    # "Move Servo 1 \"Step\" to\nSearch"
                    n784 = Subtract(x=w1769, y=u16 524) -> (x-y=w1757:u16)
                    n785 = Add(x=5, y=w1757) -> (x+y=w1775:i32)
                    n786 = Quotient & Remainder(x=w1775, y=w1767) -> (floor(x/y)=w1773:i32)  [unwired: 1 out]
                    n787 = To Byte Integer(number=w1773) -> (8bit integer=w1764:i8)
                    n788 = Less?(x=w1764, y=1) -> (x < y?=w1770:bool)
                    n789 = case shown="False" w1770 {
                      tunnel: w1764 -> [w1786 w1794]
                      tunnel: [w1788 FALSE] -> w1760
                      tunnel: [w1787 w1794] -> w1772
                      tunnel: w1766 -> [w1785 _]
                      tunnel: w1767 -> [w1783 _]
                      frame False {
                        # "Max Step"
                        # "# of steps\nminus 1"
                        n790 = Divide(x=300, y=w1783) -> (x/y=w1780:dbl)
                        n791 = To Unsigned Byte Integer(number=w1780) -> (unsigned 8bit integer=w1781:u8)
                        n792 = Greater Or Equal?(x=w1786, y=w1781) -> (x >= y?=w1782:bool)
                        n793 = case shown="True" w1782 {
                          tunnel: [w1789 TRUE] -> w1788
                          tunnel: [w1790 w1791] -> w1787
                          tunnel: w1786 -> [w1790 w1791]
                          tunnel: w1785 -> [w1789 _]
                          frame False {
                            # "No Need to\nChange Direction"
                          }
                          frame True {
                            # "T"
                            # "Move CW"
                          }
                        }
                      }
                      frame True {
                        # "F"
                        # "Move CCW"
                      }
                    }
                    n794 = case shown="True" w1760 {
                      tunnel: w1772 -> [w1777 w1778]
                      tunnel: [w1776 w1779] -> w1768
                      frame False {
                        # "CCW\n+1"
                        n795 = Increment(x=w1777) -> (x+1=w1776:i8)
                      }
                      frame True {
                        # "CW\n-1"
                        n796 = Decrement(x=w1778) -> (x-1=w1779:i8)
                      }
                    }
                    n797 = Multiply(x=w1768, y=w1767) -> (x*y=w1765:u16)
                    n798 = To Unsigned Word Integer(number=w1765) -> (unsigned 16bit integer=w1763:u16)
                    n799 = Add(x=w1763, y=u16 524) -> (x+y=w1759:u16)
                  }
                }
                n800 = local read "Image Lock - Left"() -> (w1722:bool)
                n801 = case shown="False" w1721 {
                  tunnel: [w1740 w1750] -> w1728
                  tunnel: w1729 -> [w1741 _]
                  tunnel: [w1742 enum16{"Generic Sweep", "Recovery Search"}."Generic Sweep"] -> w1726
                  tunnel: [w1739 w1750] -> w1727
                  tunnel: w1722 -> [w1738 _]
                  frame False {
                    # "Is other servo tracking?"
                    n802 = case shown="True" w1738 {
                      tunnel: [enum16{"Generic Sweep", "Recovery Search"}."Generic Sweep" enum16{"Generic Sweep", "Recovery Search"}."Recovery Search"] -> w1742
                      tunnel: w1741 -> [w1745 _]
                      tunnel: [w1745 FALSE] -> w1740
                      tunnel: [FALSE TRUE] -> w1739
                      frame False {
                        # "Stay in Sweep"
                      }
                      frame True {
                        # "G o to Recovery Search  State"
                      }
                    }
                  }
                  frame True {
                    w1750 = FALSE
                    # "Override Move Servo\nCommand bc an Angle Was Found\nduring this Step"
                    # "Stay In Sweep\nLet Main State Machine transition\ninto Tracking"
                  }
                }
              }
            }
            n803 = Increment(x=w1610) -> (x+1=w1591:i32)
            n804 = case shown="False" w1602 {
              tunnel: w1591 -> [w1625 _]
              tunnel: [w1625 0] -> w1603
              frame False {
              }
              frame True {
              }
            }
            n805 = case shown="False" w1590 {
              tunnel: [T5."Recovery Mode" ("Next Main State") T5."Tracking" ("Next Main State")] -> w1601
              frame False {
              }
              frame True {
              }
            }
          }
        }
        "Current Move Delta - R" <- w1321
        n806 = local write "New Data  Flag\nRight Servo"(FALSE) -> ()
        n807 = Less?(x=w1348, y=w1347) -> (x < y?=w1346:bool)
        n808 = Select(t=w1347, s=w1346, f=w1348) -> (s? t:f=w1343:u16)
        n809 = Greater?(x=w1343, y=w1344) -> (0:w1345:bool)
        n810 = Select(t=w1344, s=w1345, f=w1343) -> (s? t:f=w1342:u16)
      }
    }
    "Next Main State - Right" <- w1187
    "Next Tracking State - Right" <- w1193
    "Next Recovery State - Right" <- w1192
    n811 = flat-sequence {
      tunnel: w1278 -> [w2289]
      tunnel: w1188 -> [w2288]
      tunnel: w1279 -> [w2291]
      tunnel: w1189 -> [w2290]
      tunnel: [w2289] -> w1292
      tunnel: [w2288] -> w1291
      tunnel: w1292 -> [w2297]
      tunnel: [w2296] -> w1287
      tunnel: [w2295] -> w1288
      tunnel: w1291 -> [w2294]
      frame #0 {
        # "Only Update GP if Moving Servo"
        n812 = case shown="True" w2289 {
          tunnel: w2291 -> [_ w2293]
          frame False {
          }
          frame True {
            # "Update Goal Position"
            n813 = local write "Servo Goal Position\n - Left"(w2293) -> ()
          }
        }
        n814 = case shown="True" w2288 {
          tunnel: w2290 -> [_ w2292]
          frame False {
          }
          frame True {
            # "New Direction"
            # "Update Goal Position"
            # "Update Direction"
            n815 = local write "Servo Goal Position\n - Right"(w2292) -> ()
          }
        }
      }
      frame #1 {
        # "Allow Comm Process to Take Down the Flag\nOnly Raise if not already in motion"
        n816 = local read "Servo Moving - R"() -> (w2302:bool)
        n817 = local read "Servo Moving - L"() -> (w2299:bool)
        n818 = local read "Move Servo - L"() -> (w2298:bool)
        n819 = local read "Move Servo - R"() -> (w2305:bool)
        n820 = Not(x=w2302) -> (.not. x?=w2304:bool)
        n821 = Not(x=w2299) -> (.not. x?=w2301:bool)
        n822 = And(x=w2294, y=w2304) -> (x .and. y?=w2303:bool)
        n823 = And(x=w2297, y=w2301) -> (x .and. y?=w2300:bool)
        n824 = case shown="True" w2303 {
          selector: w2303 -> [_ w2307]
          tunnel: [w2306 w2307] -> w2295
          tunnel: w2305 -> [w2306 _]
          frame False {
          }
          frame True {
          }
        }
        n825 = case shown="False" w2300 {
          selector: w2300 -> [_ w2309]
          tunnel: [w2308 w2309] -> w2296
          tunnel: w2298 -> [w2308 _]
          frame False {
          }
          frame True {
          }
        }
        n826 = local write "Move Servo - R"(w2295) -> ()
        n827 = local write "Move Servo - L"(w2296) -> ()
      }
    }
    n828 = local read "Current Tracking State - Right 2"() -> (w1232:enum16{"Track", "Reactive Predict", ""})
    n829 = local read "Current Tracking State - Left"() -> (w1234:enum16{"Track", "Reactive Predict", ""})
    n830 = local read "Current Main State - Left"() -> (w1258:T5)
    n831 = local read "Current Main State - Right"() -> (w1233:T5)
    n832 = Equal?(x=w1233, y=w1257) -> (x = y?=w1227:bool)
    n833 = Equal?(x=w1232, y=w1231) -> (x = y?=w1226:bool)
    n834 = Equal?(x=w1258, y=w1257) -> (x = y?=w1229:bool)
    n835 = Equal?(x=w1234, y=w1231) -> (x = y?=w1230:bool)
    n836 = And(x=w1227, y=w1226) -> (x .and. y?=w1225:bool)
    n837 = And(x=w1229, y=w1230) -> (x .and. y?=w1228:bool)
    n838 = And(x=w1228, y=w1287) -> (x .and. y?=w1283:bool)
    n839 = And(x=w1288, y=w1225) -> (x .and. y?=w1284:bool)
    n840 = And(x=w1228, y=w1225) -> (x .and. y?=w1282:bool)
    n841 = Exclusive Or(1:w1284, 2:w1283) -> (0:w1281:bool)
    n842 = case shown="True" w1281 {
      tunnel: [w2320 w2341] -> w1289
      tunnel: [w2321 w2340] -> w1285
      tunnel: w1190 -> [_ w2344]
      tunnel: w1248 -> [w2318 w2345]
      tunnel: w1201 -> [w2316 w2343]
      tunnel: [w2319 w2331] -> w1286
      tunnel: [w2317 w2330] -> w1290
      tunnel: w1256 -> [_ w2342]
      tunnel: w1282 -> [w2315 _]
      tunnel: w1283 -> [_ w2341]
      tunnel: w1284 -> [_ w2340]
      frame False {
        n843 = case shown="False" w2315 {
          tunnel: [w2325 w2327] -> w2321
          tunnel: [w2324 w2327] -> w2320
          tunnel: [w2323 w2326] -> w2319
          tunnel: w2318 -> [w2323 _]
          tunnel: [w2322 w2326] -> w2317
          tunnel: w2316 -> [w2322 _]
          frame False {
            # "No Movement\nRetain All Values"
            n844 = local read "Move Respond - L"() -> (w2325:bool)
            n845 = local read "Move Respond - R"() -> (w2324:bool)
          }
          frame True {
            w2326 = i16 0
            w2327 = FALSE
            # "Reset Delta Move sum\nfor both"
            # "F"
            # "Both Moved,\nMake Flags False"
          }
        }
      }
      frame True {
        w2337 = 200 ("y")
        w2328 = -200 ("y")
        # "Add/Clear Sum for \nServo That didn't move"
        # "Update Moving Servo's  Delta Position"
        # "if one Servo Moves, other should \nmove too eventually,\nUsed in Search Process"
        # "Only 1 Servo is Moving Due to Tracking --> Update delta move sum"
        n846 = case shown="True" w2340 {
          tunnel: w2345 -> [_ w2353]
          tunnel: w2344 -> [_ w2352]
          tunnel: [i16 0 w2351] -> w2338
          frame False {
          }
          frame True {
            n847 = Add(x=w2353, y=w2352) -> (x+y=w2351:i32)
          }
        }
        n848 = case shown="True" w2341 {
          tunnel: w2343 -> [_ w2349]
          tunnel: w2342 -> [_ w2348]
          tunnel: [i16 0 w2347] -> w2335
          frame False {
          }
          frame True {
            n849 = Add(x=w2349, y=w2348) -> (x+y=w2347:i32)
          }
        }
        n850 = Greater?(x=w2338, y=w2337) -> (0:w2339:bool)
        n851 = Greater?(x=w2335, y=w2337) -> (0:w2336:bool)
        n852 = Select(t=w2337, s=w2336, f=w2335) -> (s? t:f=w2332:i32)
        n853 = Select(t=w2337, s=w2339, f=w2338) -> (s? t:f=w2333:i32)
        n854 = Greater?(x=w2333, y=w2328) -> (0:w2329:bool)
        n855 = Greater?(x=w2332, y=w2328) -> (0:w2334:bool)
        n856 = Select(t=w2332, s=w2334, f=w2328) -> (s? t:f=w2330:i32)
        n857 = Select(t=w2333, s=w2329, f=w2328) -> (s? t:f=w2331:i32)
      }
    }
    n858 = case shown="True" w1194 {
      selector: w1194 -> [_ w2287]
      tunnel: [w2284 w2286] -> w1243
      tunnel: [w2283 i16 0] -> w1244
      tunnel: w1289 -> [w2284 _]
      tunnel: w1290 -> [w2283 _]
      frame False {
      }
      frame True {
        n859 = Not(x=w2287) -> (.not. x?=w2286:bool)
      }
    }
    "Move Respond - R" <- w1243
    "deltaMoveServo\n- R" <- w1244
    n860 = case shown="False" w1254 {
      selector: w1254 -> [_ w2314]
      tunnel: [w2311 w2313] -> w1246
      tunnel: [w2310 i16 0] -> w1249
      tunnel: w1285 -> [w2311 _]
      tunnel: w1286 -> [w2310 _]
      frame False {
      }
      frame True {
        n861 = Not(x=w2314) -> (.not. x?=w2313:bool)
      }
    }
    "Move Respond - L" <- w1246
    "deltaMoveServo\n- L" <- w1249
    "Current Main State - Left" <- w1277
    "Frames Processed\nCount - in -L" <- w1269
    "Recovery Mode Count - in Left" <- w1264
    "Recovery Search\nmove Count - in - L" <- w1263
    "Recovery Search\nAttempt Count - in - L" <- w1262
    "Current Main State - Right" <- w1224
    "Frames Processed\nCount - in Right" <- w1207
    "Recovery Search\nmove Count - Right" <- w1209
    "Recovery Search\nAttempt Count - Right" <- w1208
    "Recovery Mode Count in Right" <- w1200
    "Tracking Timeout\nCount - L" <- w1241
    "Tracking Timeout\nCount - R" <- w1216
    "Current Tracking State - Left" <- w1240
    "Current Tracking State - Right 2" <- w1222
    "Current Recovery State - Right" <- w1223
    "Current Recovery State -L" <- w1237
  }
